vi "TLB Native Dynamic Events ver 0.18a.vi"() -> ()   [LabVIEW 2018]
uses:
  Labview Training Phase 2/Enum Controls/States for Action Engine.ctl
  TLB Type Definitions/State Type Definitions.ctl
  TLB Type Definitions/Intruction Type Definitions.ctl
  TLB Type Definitions/Encoder cluster.ctl
  TLB Type Definitions/PING CLUSTER.ctl
  <vilib>/Studica/Studica Toolkit/NavX/NavX.lvlib
  <vilib>/Studica/Studica Toolkit/Background/DIO Channel.ctl
  Underlying VI's/NavX VI/navX type def.ctl
  <vilib>/Studica/Studica Toolkit/Background/I2C Channel.ctl
  TLB Type Definitions/Vision cluster.ctl
  <vilib>/NI_Real-Time Target Support.lvlib
  TLB Type Definitions/Stepper cluster.ctl
  Experimental VI's/Archived VI's/MOTOR CONTROL NO PID Type Def.ctl
  Underlying VI's/I2C Master VI/I2C MASTER Type Def.ctl
  Underlying VI's/I2C Master VI/I2C_MASTER_WRITE_NEW Type Def.ctl
  <vilib>/userdefined/High Color/IMAQdx.ctl
  Underlying VI's/I2C Master VI/Arduino_Interfacing.ctl
  TLB Type Definitions/Yaw Cluster.ctl
  TLB Type Definitions/Time cluster.ctl
  TLB Type Definitions/Y Stepper cluster.ctl
  Underlying VI's/Modified webcam FGV/Webcam AE.ctl
  Underlying VI's/Elasped Timer/Elapsed timer control.ctl
  Underlying VI's/Motor Control VI with PID/MOTOR CONTROL WITH PID AE DATA MODE TYPE DEF.ctl
  Underlying VI's/Motor Control VI with PID/MOTOR CONTROL WITH PID AE DIRECTION TYPE DEF.ctl
  TLB Type Definitions/IR Sensor Type Def.ctl
  <vilib>/myRIO/Common/Instrument Driver Framework/myRIO v1.0/AI/typedefs/AI Channels Enum.ctl
  <vilib>/myRIO/Common/Instrument Driver Framework/myRIO v1.0/AI/typedefs/AI Channels List.ctl
  TLB Type Definitions/Motor Speed Cluster.ctl
  Underlying VI's/IMAQ Create Reference AE/IMAQ Reference AE.ctl
  <vilib>/Utility/RT CPU Load.ctl
panel:
  out "Arm IR Sensor":dbl
  out "Table obstruct":bool
  out "x-y":dbl
  out "Left IR Sensor":dbl
  out "Obstacle detected":bool
  out "Speed & distance":T1
  out "Object Center Coordinates":cluster{"x":sgl, "y":sgl}
  out "Object detection cluster":T2
  out "Time up flag":bool
  out "Task selection":u8
  in  "Object recognition mode":enum16{"Ball", "Soap", "Gel", "Pipe", "None"}(ring)
  out "NavX Readings":T3
  out "Arduino Data":T4
  out "CPU loads":T5[](array[typedef]) {"ISR (%)" format="%#.2f"; "Idle (%)" format="%#.2f"; "Background (%)" format="%#.2f"; "Normal (%)" format="%#.2f"; "Above Normal (%)" format="%#.2f"; "High (%)" format="%#.2g"; "Timed Structures (%)" format="%#.2g"; "Time Critical (%)" format="%#.2g"; "Total (%)" format="%#.2g"}
  out "TASK ENABLE":bool
  out "Rising Edge":bool
  in  "Green LED":bool
  out "I2C Error":errorcluster
  out "State Logic":T6=enum."Startup"
  out "elements":T7[](array[typedef])
  in  "STOP TASK":bool
  in  "OK Button":bool
  in  "STOP":bool
  out "error out":errorcluster
  out "Action Queue Items":i32
  out "State Logic Queue Items":i32
  out "Action Queues items":string[](array[string])=["Hardware reset", "Software reset", ""]
  out "Action State":string
  # "System Health Status Update"
  # "VISION"
  # "TLB FRAMEWORK STATUS"
  # "Test Programme written by Calvin Loke    Dated: 28 Aug 2019\nTest Programme revised by Dr Alex See   Dated 30 Aug 2019\n\nRevision date: 20/03/2020\nProgramme version:   TLB Native Dynamic Events ver 0.14a"
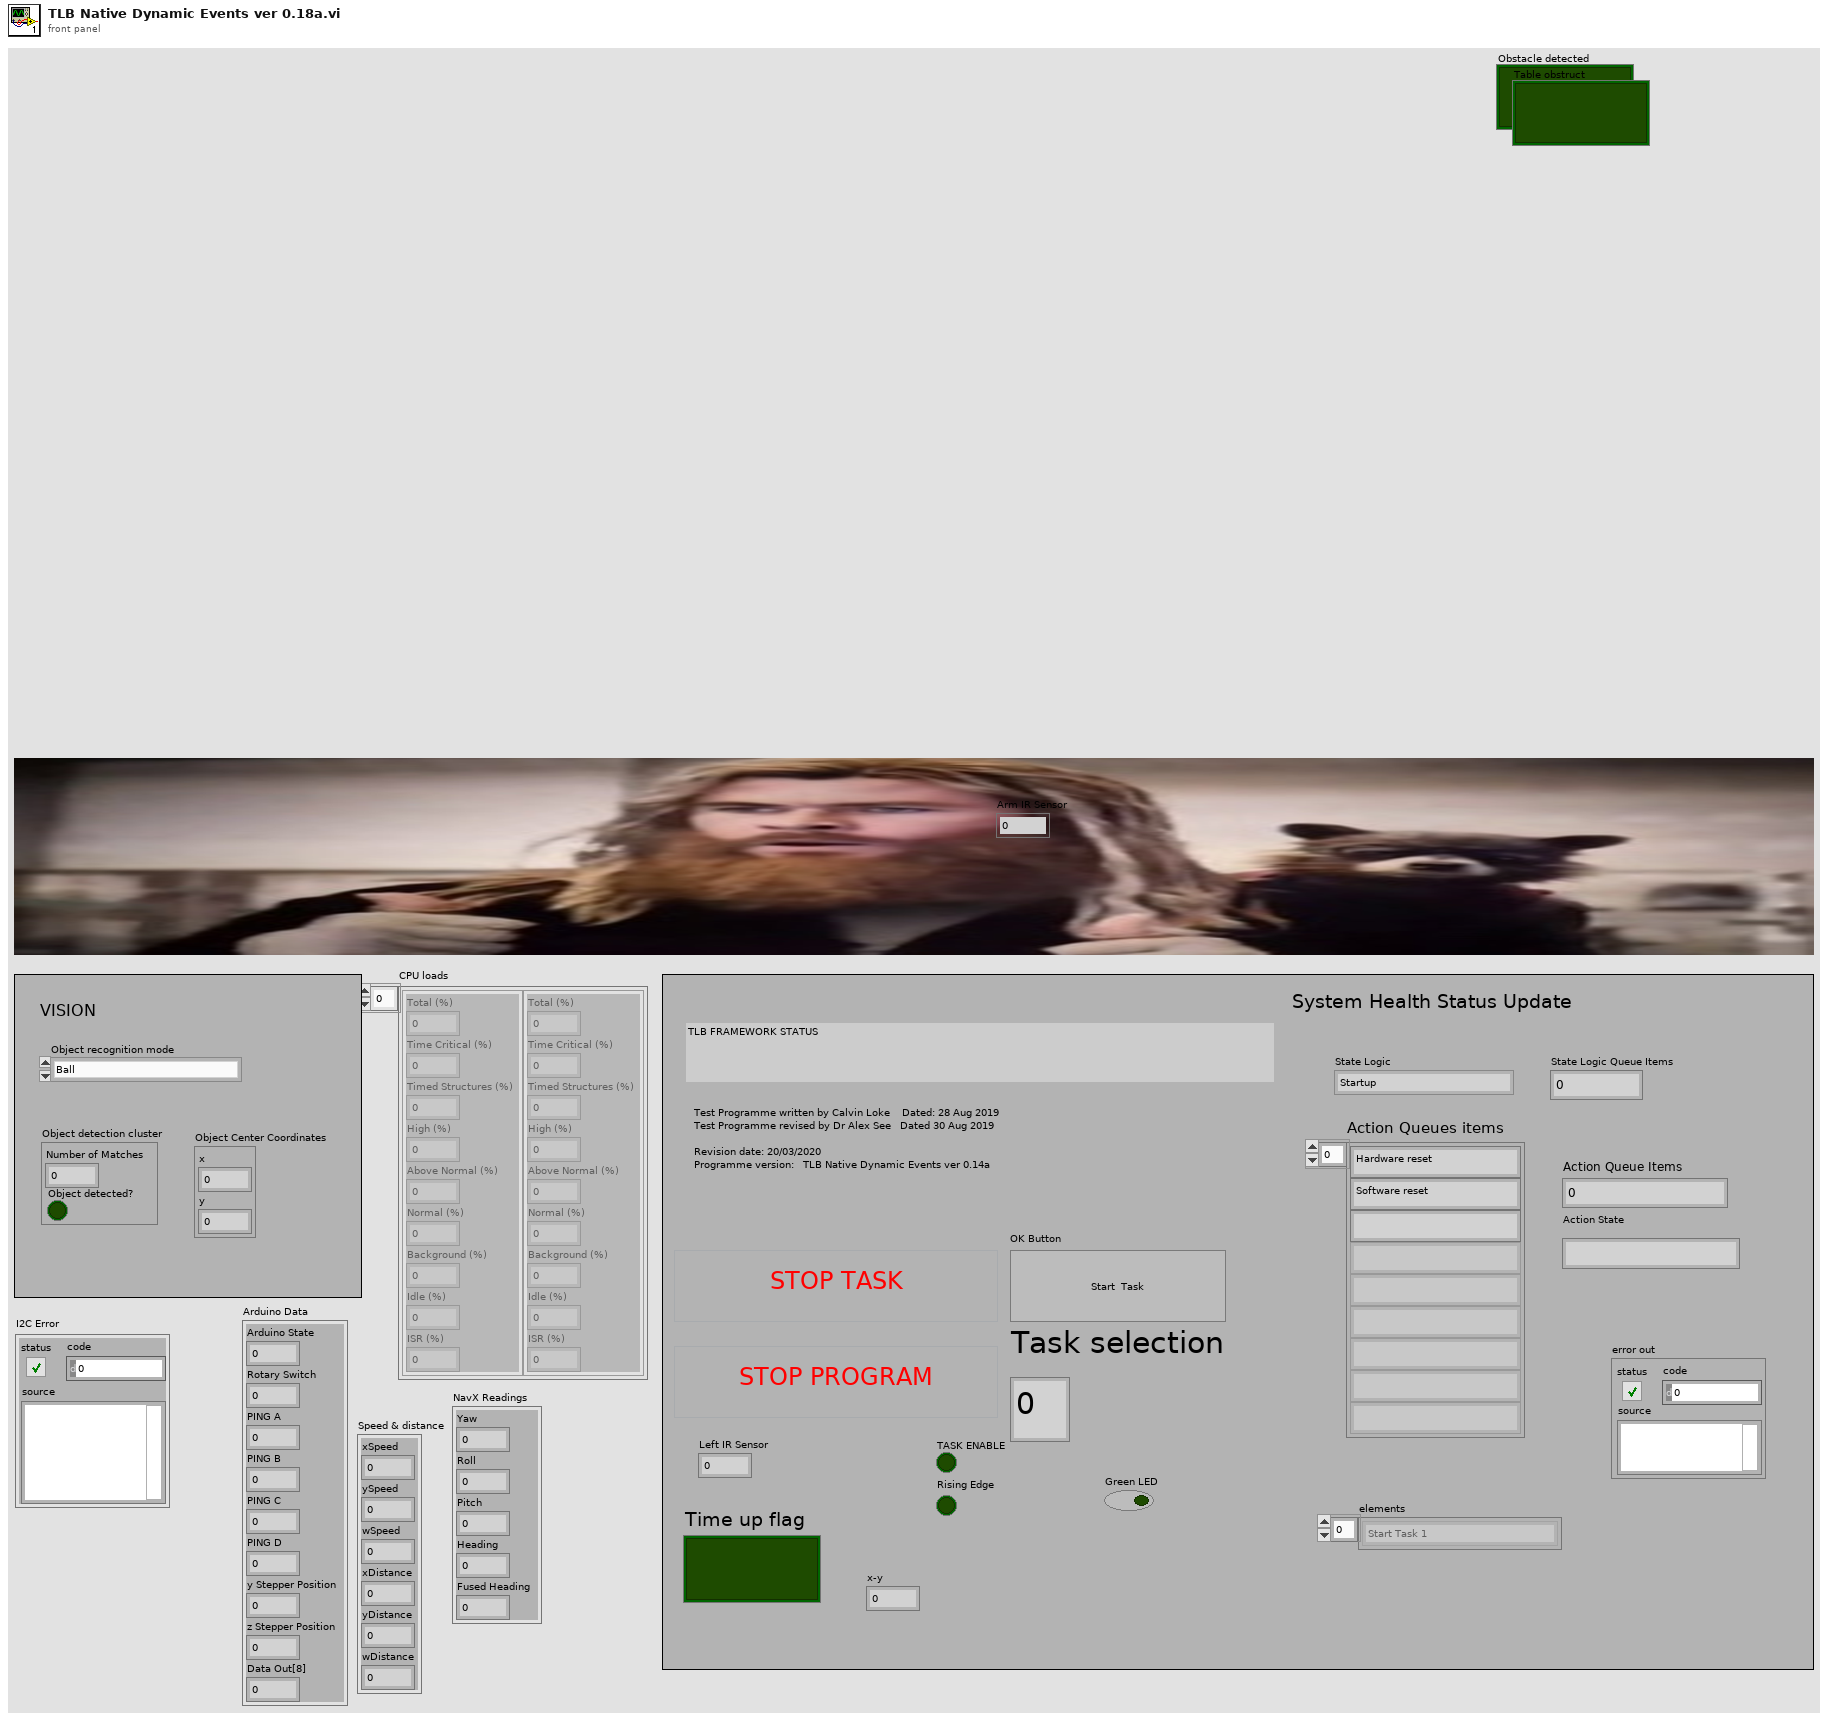
[diagram p1: front panel]
types:
  T1 = cluster{"xSpeed":dbl, "ySpeed":dbl, "wSpeed":dbl, "xDistance":dbl, "yDistance":dbl, "wDistance":dbl}
  T2 = cluster{"Number of Matches":i32, "Object detected?":bool}
  T3 = cluster{"Yaw":dbl, "Roll":dbl, "Pitch":dbl, "Heading":dbl, "Fused Heading":dbl}
  T4 = cluster{"Arduino State":u8, "Rotary Switch":u8, "PING A":u8, "PING B":u8, "PING C":u8, "PING D":u8, "y Stepper Position":u8, "z Stepper Position":u8, "Data Out[8]":u8}
  T5 = typedef "NI_Real-Time Target Support.lvlib/RT CPU Load.ctl" = cluster{"Total (%)":dbl, "Time Critical (%)":dbl, "Timed Structures (%)":dbl, "High (%)":dbl, "Above Normal (%)":dbl, "Normal (%)":dbl, "Background (%)":dbl, "Idle (%)":dbl, "ISR (%)":dbl}
  T6 = typedef "State Type Definitions.ctl" = enum16{"None", "Startup", "Move to Angle", "True Stop", "Idle", "Shutdown", "Task 1A", "Task 1B", "Task 2:Raise Arm", "Task 2:Sensor Mode", "Task 2:Reverse Mode", "Task 3", "Task 4_A", "Task 4_B", "Task 4_C", "Task 4_D", "Task 5A", "Task 5B", "Task 5C", "Task 5D", "Task 5E: POSITION ARM", "Task 5F: ARM GRAB HEIGHT", "Task 5G: CLOSE CLAW", "Task 5H: RAISE ARM", "Task 6_A", "Task 6_B", "Task 7", "Task 8A: RAISE ARM", "Task 8B: MOVE TO BOX", "Task 8C: CAM BURST", "Task 8D: PROCESS IMAGE", "Task 8E: ROBOT ADJUST", "Task 8F: CAM BURST 2", "Task 8G: PROCESS IMAGE 2", "Task 8H: ARM ADJUST", "Task 8I: ARM GRAB HEIGHT", "Task 8J: CLOSE CLAW", "Task 8K: RAISE MY SWORD", "Task 9A: Raise Arm", "Task 9B: Rotate to Angle", "Task 9C: Detect Box", "Task 9D: MOVE FORWARD", "Task 9E: MOVE LEFT", "Task 9F: SCAN IMAGE", "Task 9G: PROCESS COLOUR", "Task 9H: MOVE RIGHT", "Task 9I: SCAN IMAGE", "Task 9J: PROCESS COLOUR", "Task 9K: ROTATE 90 CW", "Task 9L: MOVE FORWARD", "Task 9M: MOVE RIGHT", "Task 9N: SCAN IMAGE", "Task 9O: PROCESS COLOUR", "Task 9P: MOVE RIGHT", "Task 9Q: SCAN IMAGE", "Task 9R: PROCESS COLOUR", "Task A1: Raise Arm", "Task A2: Rotate to Angle", "Task A3: Move Forward", "Task A4: Rotate CW 90"}
  T7 = typedef "Intruction Type Definitions.ctl" = enum16{"None", "Start Task 1", "Start Task 2", "Start Task 3", "Start Task 4", "Start Task 5", "Start Task 6", "Start Task 7", "Start Task 8 - BALL", "Start Task 8 - Gel", "Start Task 8 - Pipe", "Start Task 8 - Soap", "Start Task 9", "Start Task A", "Start Task B", "Exit"}
  T8 = typedef "Motor Speed Cluster.ctl" = cluster{"ySpeed":dbl, "xSpeed":dbl, "wSpeed":dbl}
  T9 = typedef "IR Sensor Type Def.ctl" = cluster{"Left IR Sensor":dbl, "Arm IR Sensor":dbl, "Bottom IR Sensor":dbl}
  T10 = typedef "Y Stepper cluster.ctl" = cluster{"yStepper desired":u8}
  T11 = typedef "Time cluster.ctl" = cluster{"Time up flag":bool, "SET TIME TO CHECK":dbl}
  T12 = typedef "Yaw Cluster.ctl" = cluster{"Yaw":dbl, "Compass":dbl}
  T13 = typedef "Stepper cluster.ctl" = cluster{"y Stepper Position":u8, "z Stepper Position":u8}
  T14 = typedef "DIO Channel.ctl" = enum16{"Not Connected", "A/DIO1", "A/DIO2", "A/DIO3", "A/DIO4", "A/DIO5", "A/DIO6", "A/DIO7", "A/DIO13", "B/DIO1", "B/DIO2", "B/DIO3", "B/DIO4", "B/DIO5", "B/DIO6", "B/DIO7", "B/DIO13", "C/DIO0", "C/DIO1", "C/DIO2", "C/DIO3", "C/DIO4", "C/DIO5", "C/DIO6", "C/DIO7"}
  T15 = typedef "Vision cluster.ctl" = cluster{"Recognized Object":bool, "Object X coordinate":dbl, "Object Y coordinate":dbl}
  T16 = typedef "PING CLUSTER.ctl" = cluster{"PING_A":u8, "PING_B":u8, "PING_C":u8, "PING_D":u8}
  T17 = typedef "Encoder cluster.ctl" = cluster{"xDistance":dbl, "yDistance":dbl, "wDistance":dbl}
  T18 = cluster{"DIO Channel":T14, "FPGA VI Reference Out":refnum<k20>}
  T19 = typedef "navX type def.ctl" = enum16{"Get i2C reference", "Read Values", "Zero Yaw"}
  T20 = typedef "Arduino_Interfacing.ctl" = enum16{"Initialize", "Write to Arduino", "Read From Arduino"}
  T21 = typedef "I2C Channel.ctl" = enum16{"Not Connected", "A", "B"}
  T22 = typedef "States for Action Engine.ctl" = enum16{"Initialize", "Write", "Read"}
  T23 = cluster{"I2C Ref Out":cluster{"I2C Channel":T21, "FPGA VI Reference Out":refnum<k20>}, "Connected":bool, "Slave Address (7-bit)":u8, "Registry":u8[]}
  T24 = typedef "Intruction Type Definitions.ctl" = enum16{"None", "Start Task 1", "Start Task 2", "Start Task 3", "Start Task 4", "Start Task 5", "Start Task 6", "Start Task 7", "Start Task 8", "Start Task 9", "Start Task A", "Start Task B", "Exit"}
  T25 = typedef "State Type Definitions.ctl" = enum16{"None", "Startup", "Move to Angle", "True Stop", "Idle", "Shutdown", "Task 1", "Task 2:Raise Arm", "Task 2:Sensor Mode", "Task 2:Reverse Mode", "Task 3", "Task 4_A", "Task 4_B", "Task 4_C", "Task 4_D", "Task 5A: ARM CAM HEIGHT", "Task 5B: MOVE TO BOX", "Task 5C: CAM BURST", "Task 5D: PROCESS IMAGE", "Task 5E: POSITION ARM", "Task 5F: ARM GRAB HEIGHT", "Task 5G: CLOSE CLAW", "Task 5H: RAISE ARM", "Task 6_A", "Task 6_B", "Task 7", "Task 8A: RAISE ARM", "Task 8B: MOVE TO BOX", "Task 8C: CAM BURST", "Task 8D: PROCESS IMAGE", "Task 8E: ROBOT ADJUST", "Task 8F: CAM BURST 2", "Task 8G: PROCESS IMAGE 2", "Task 8H: ARM ADJUST", "Task 8I: ARM GRAB HEIGHT", "Task 8J: CLOSE CLAW", "Task 8K: RAISE MY SWORD", "Task 9A: Raise Arm", "Task 9B: Rotate to Angle", "Task 9C: Rotation alignmnet", "Task A: RAISE ARM TO HEIGHT", "Task A: MOVE FORWARD"}
  T26 = typedef "MOTOR CONTROL WITH PID AE DIRECTION TYPE DEF.ctl" = enum16{"y-axis movement", "x-axis movement", "rotation", "stop", "reset encoders"}
  T27 = typedef "MOTOR CONTROL WITH PID AE DATA MODE TYPE DEF.ctl" = enum16{"Init AE", "Write to AE", "Read from AE"}
  T28 = typedef "IMAQ Reference AE.ctl" = enum16{"Initialize AE", "Get IMAQ Reference", "Dispose Processing Buffer"}
  T29 = typedef "Elapsed timer control.ctl" = enum16{"Start", "Pause", "Initialize"}
  T30 = typedef "I2C_MASTER_WRITE_NEW Type Def.ctl" = enum16{"Ultrasonic sensors", "Stepper origin", "zStepper 13.3k", "zStepper 13k", "zStepper 12k", "zStepper 11k", "zStepper 10k", "zStepper 9k", "zStepper 8k", "zStepper 7k", "zStepper 6k", "zStepper 5k", "zStepper 4k", "zStepper 3k", "zStepper 2k", "zStepper 1k", "zStepper 900", "zStepper 800", "zStepper 700", "zStepper 600", "zStepper 500", "zStepper 400", "zStepper 300", "zStepper 200", "zStepper 100", "zStepper 0", "yStepper control", "Open Claw", "Close Claw", "Soft Reset"}
  T31 = typedef "Webcam AE.ctl" = enum16{"Initialize Camera", "Open Camera", "Continuous Acquisition", "Close Camera", "Retrieve Image", "Dispose Camera Image Buffer"}
  T32 = typedef "IMAQdx.ctl" = refnum<k21>
  T33 = typedef "Webcam AE.ctl" = enum16{"Initialize Camera", "Open Camera", "Continuous Acquisition", "Close Camera", "Retrieve Image", "Dispose Image Buffers"}
  T34 = typedef "IMAQ Reference AE.ctl" = enum16{"Initialize AE", "Get IMAQ Reference", "Destroy ALL IMAQ"}
  T35 = typedef "MOTOR CONTROL NO PID Type Def.ctl" = enum16{"Init", "Front Back", "Left Right", "Rotate", "Stop", "Latch"}
  T36 = typedef "AI Channels List.ctl" = T37[]
  T37 = typedef "AI Channels Enum.ctl" = enum16{"Not Connected", "AudioIn/Left", "AudioIn/Right", "C/AI0", "C/AI1", "A/AI0", "A/AI1", "A/AI2", "A/AI3", "A/AI4", "A/AI5", "A/AI6", "A/AI7", "B/AI0", "B/AI1", "B/AI2", "B/AI3", "B/AI4", "B/AI5", "B/AI6", "B/AI7", "AI/AI0", "AI/AI1", "AI/AI2", "AI/AI3", "A/AI0 (DIFF)", "A/AI1 (DIFF)", "A/AI2 (DIFF)", "A/AI3 (DIFF)", "B/AI0 (DIFF)", "B/AI1 (DIFF)", "B/AI2 (DIFF)", "B/AI3 (DIFF)"}
  T38 = typedef "I2C MASTER Type Def.ctl" = enum16{"Last State", "Mode 0", "Mode 1", "Mode 2", "Mode 3", "Mode 4", "Mode 5", "Mode 6", "Mode 7", "Mode 8", "Mode 9", "Mode 10"}
  T39 = typedef "IMAQ Image.ctl" = refnum<image>
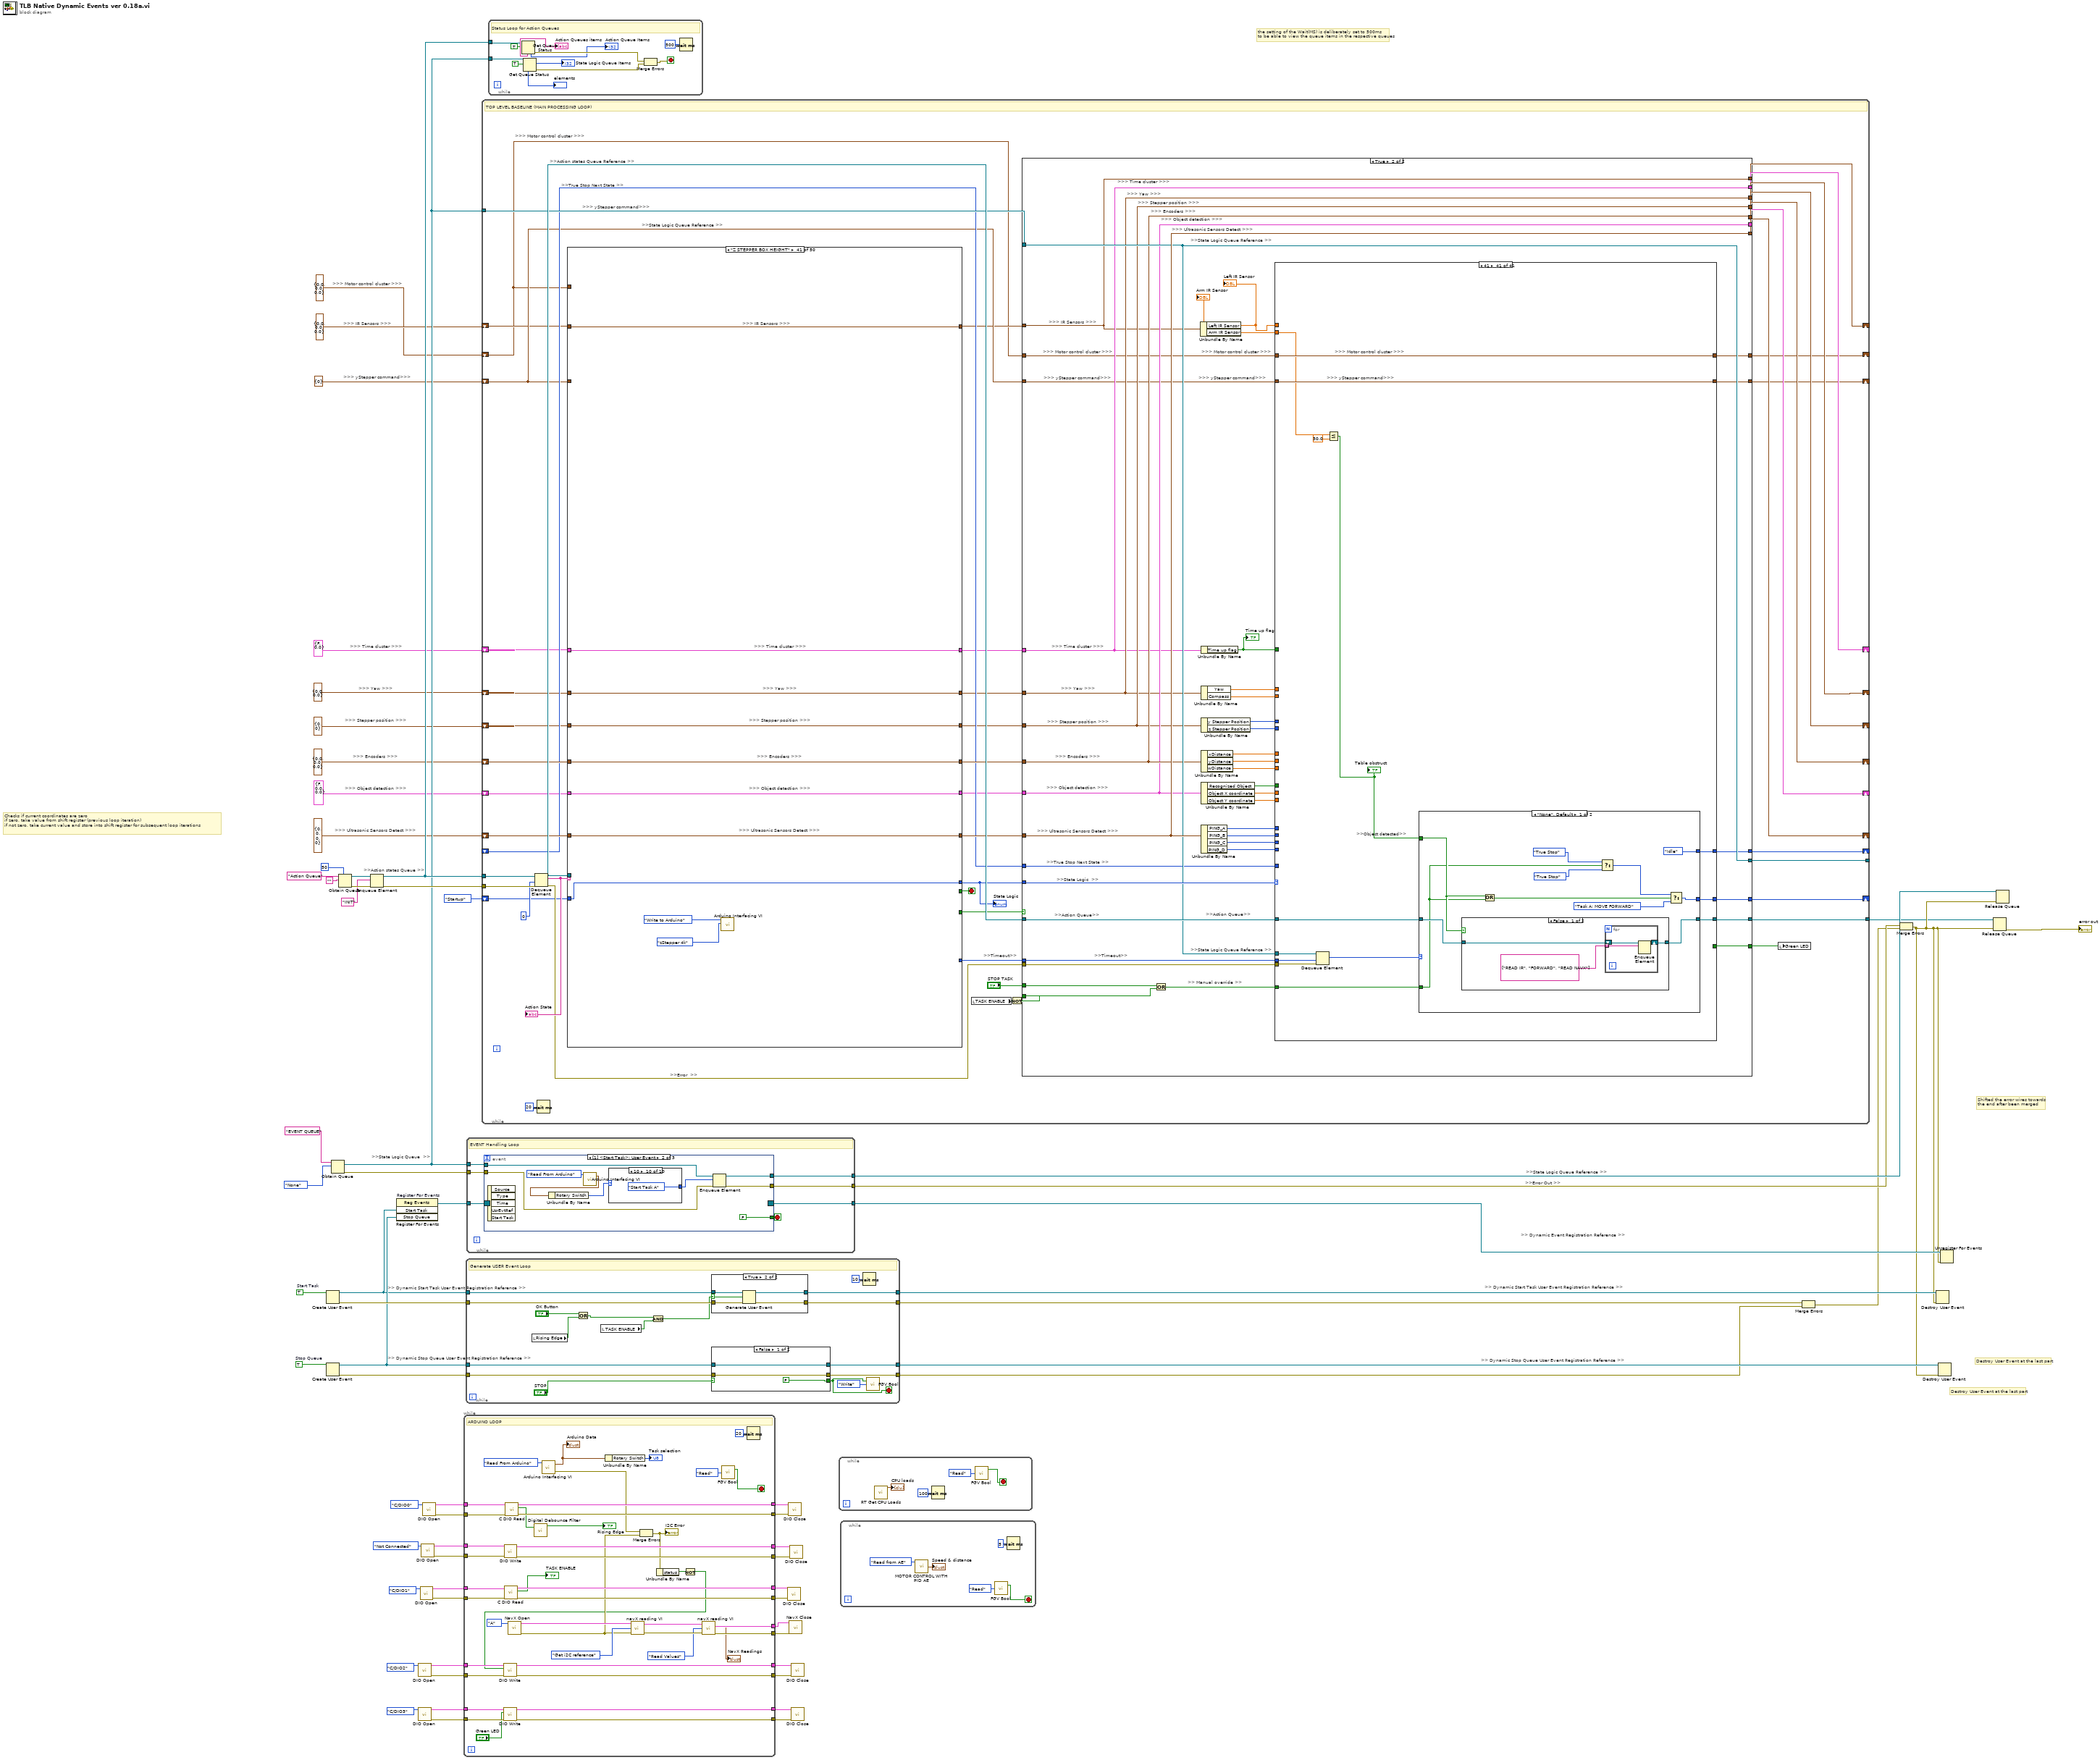
[diagram p0: block diagram]
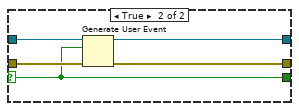
[diagram p2: hidden frame]
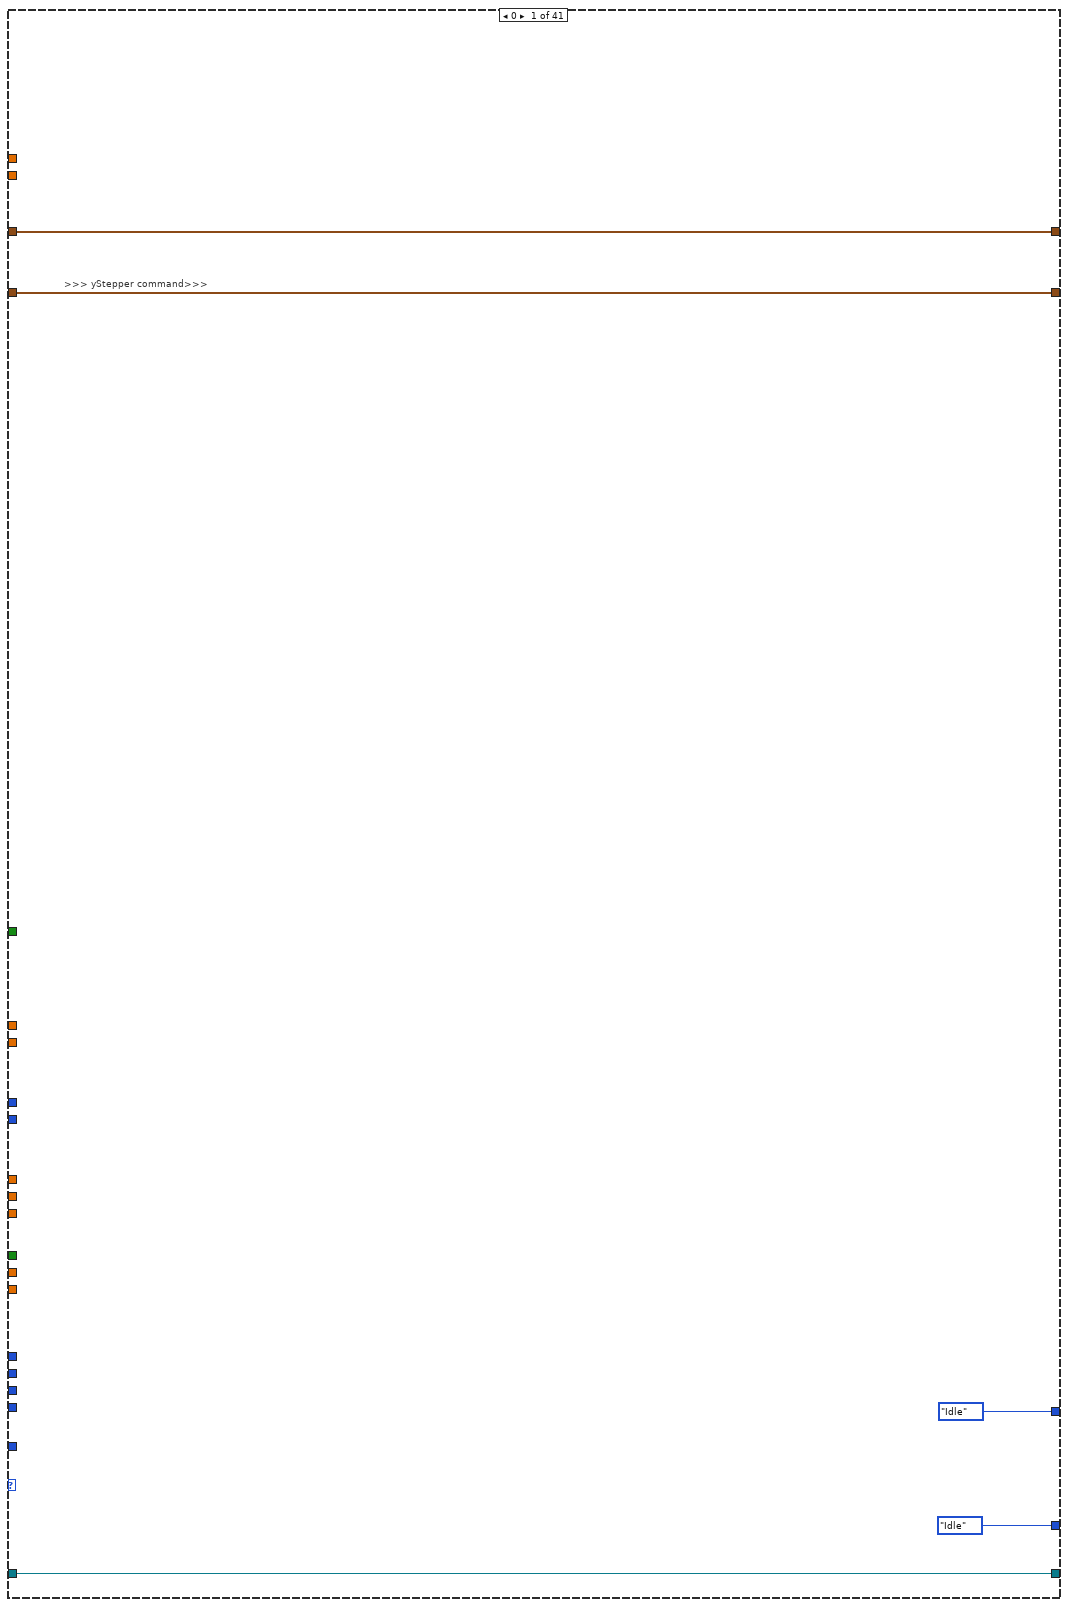
[diagram p5: hidden frame]
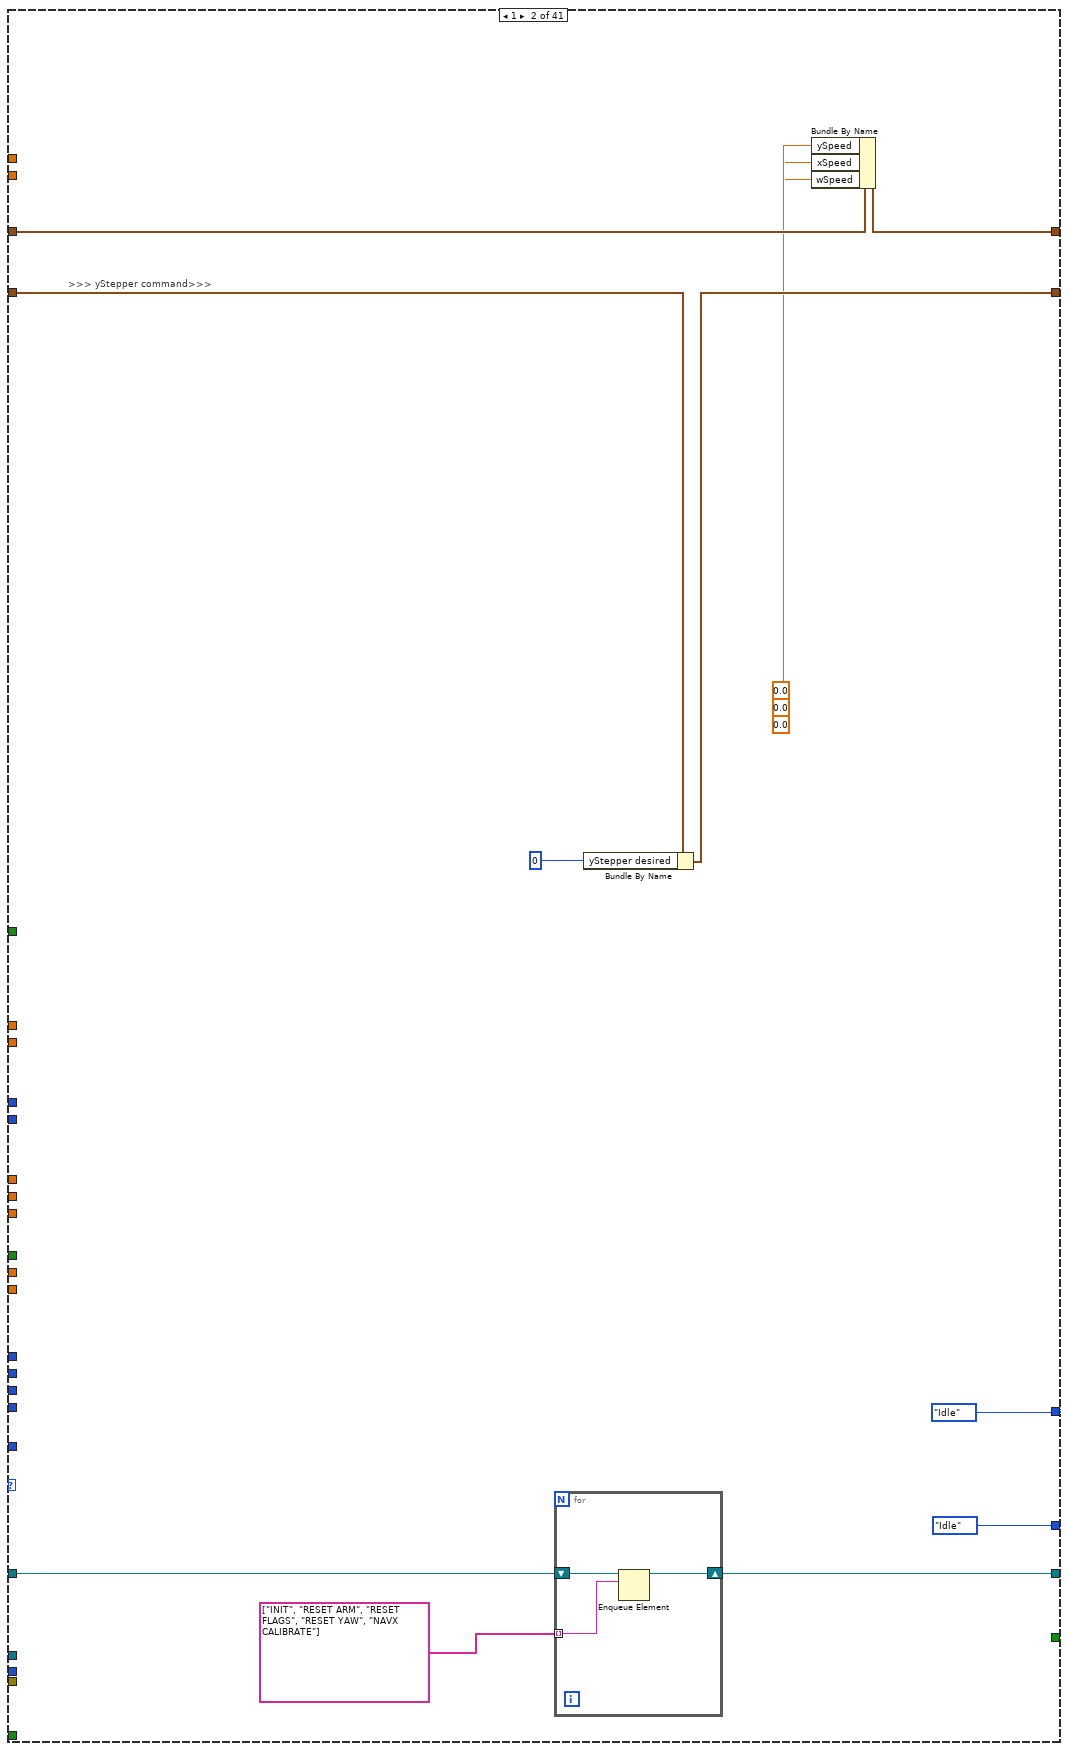
[diagram p6: hidden frame]
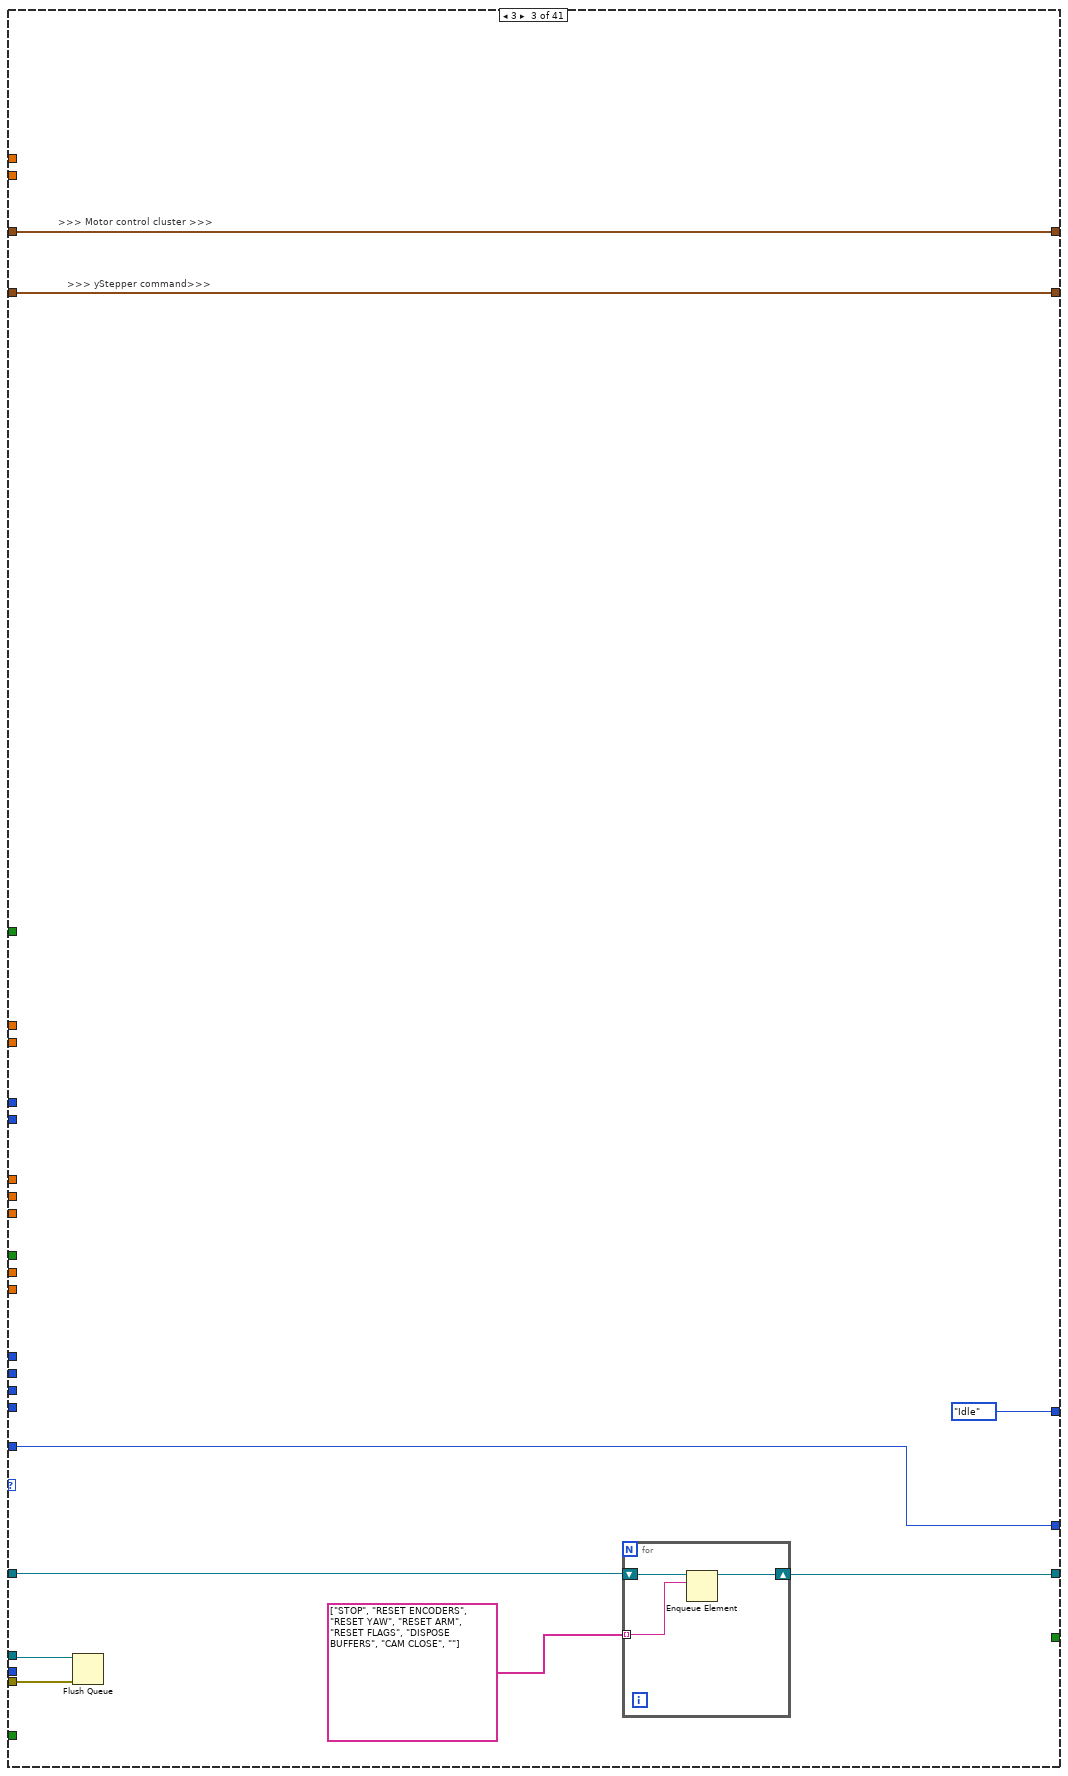
[diagram p7: hidden frame]
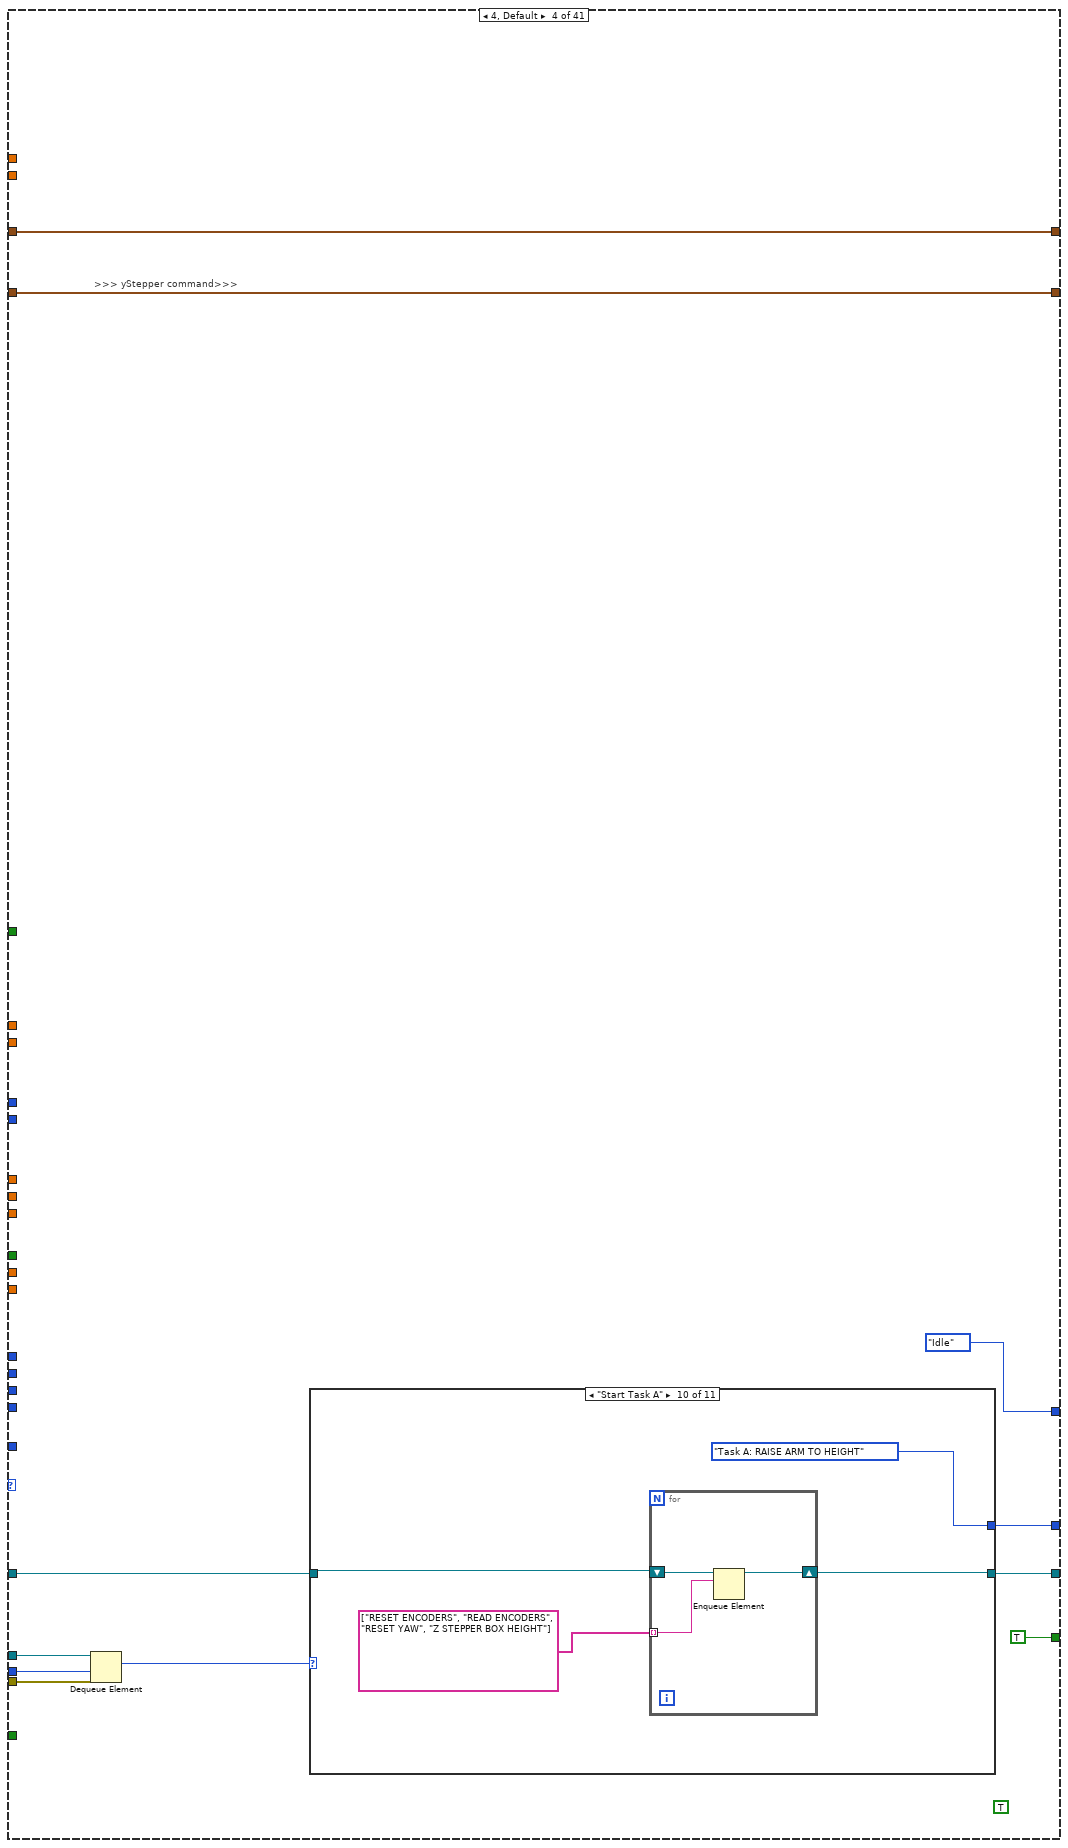
[diagram p8: hidden frame]
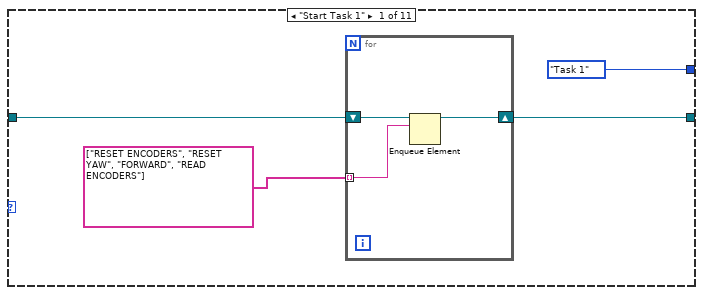
[diagram p9: hidden frame]
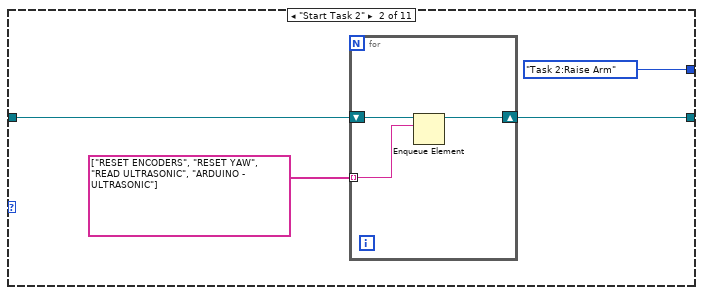
[diagram p10: hidden frame]
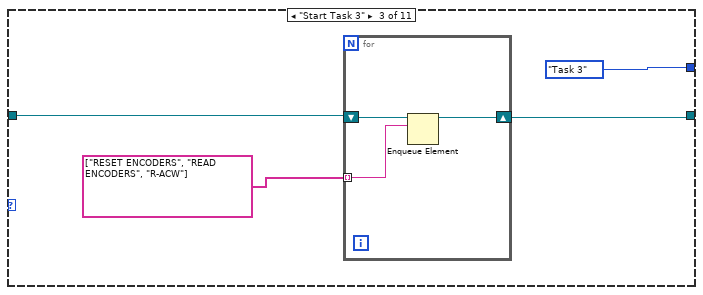
[diagram p11: hidden frame]
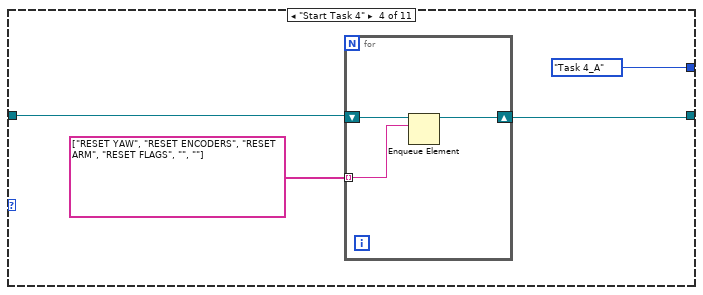
[diagram p12: hidden frame]
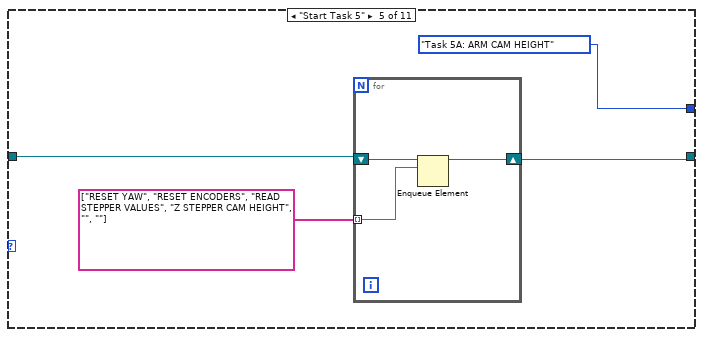
[diagram p13: hidden frame]
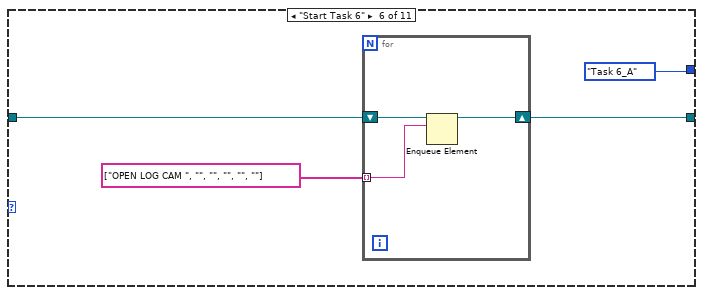
[diagram p14: hidden frame]
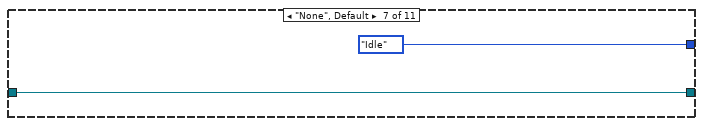
[diagram p15: hidden frame]
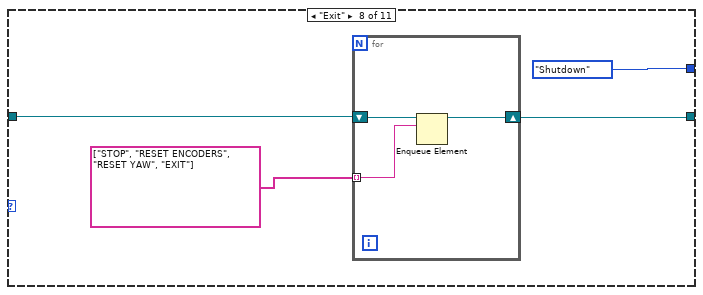
[diagram p16: hidden frame]
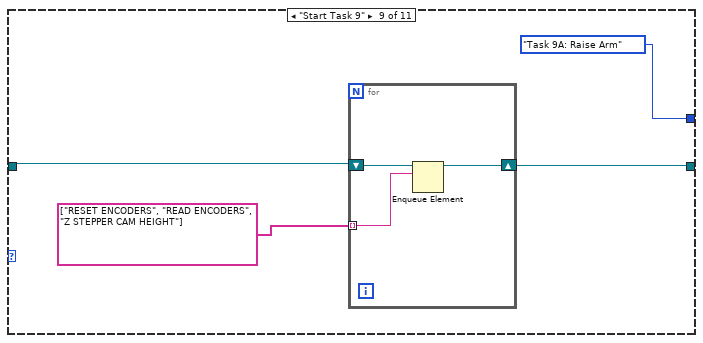
[diagram p17: hidden frame]
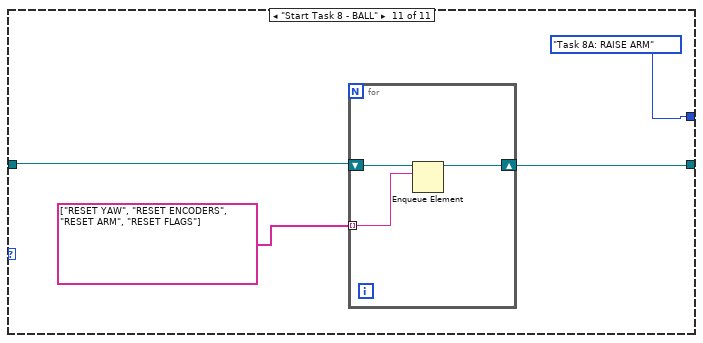
[diagram p18: hidden frame]
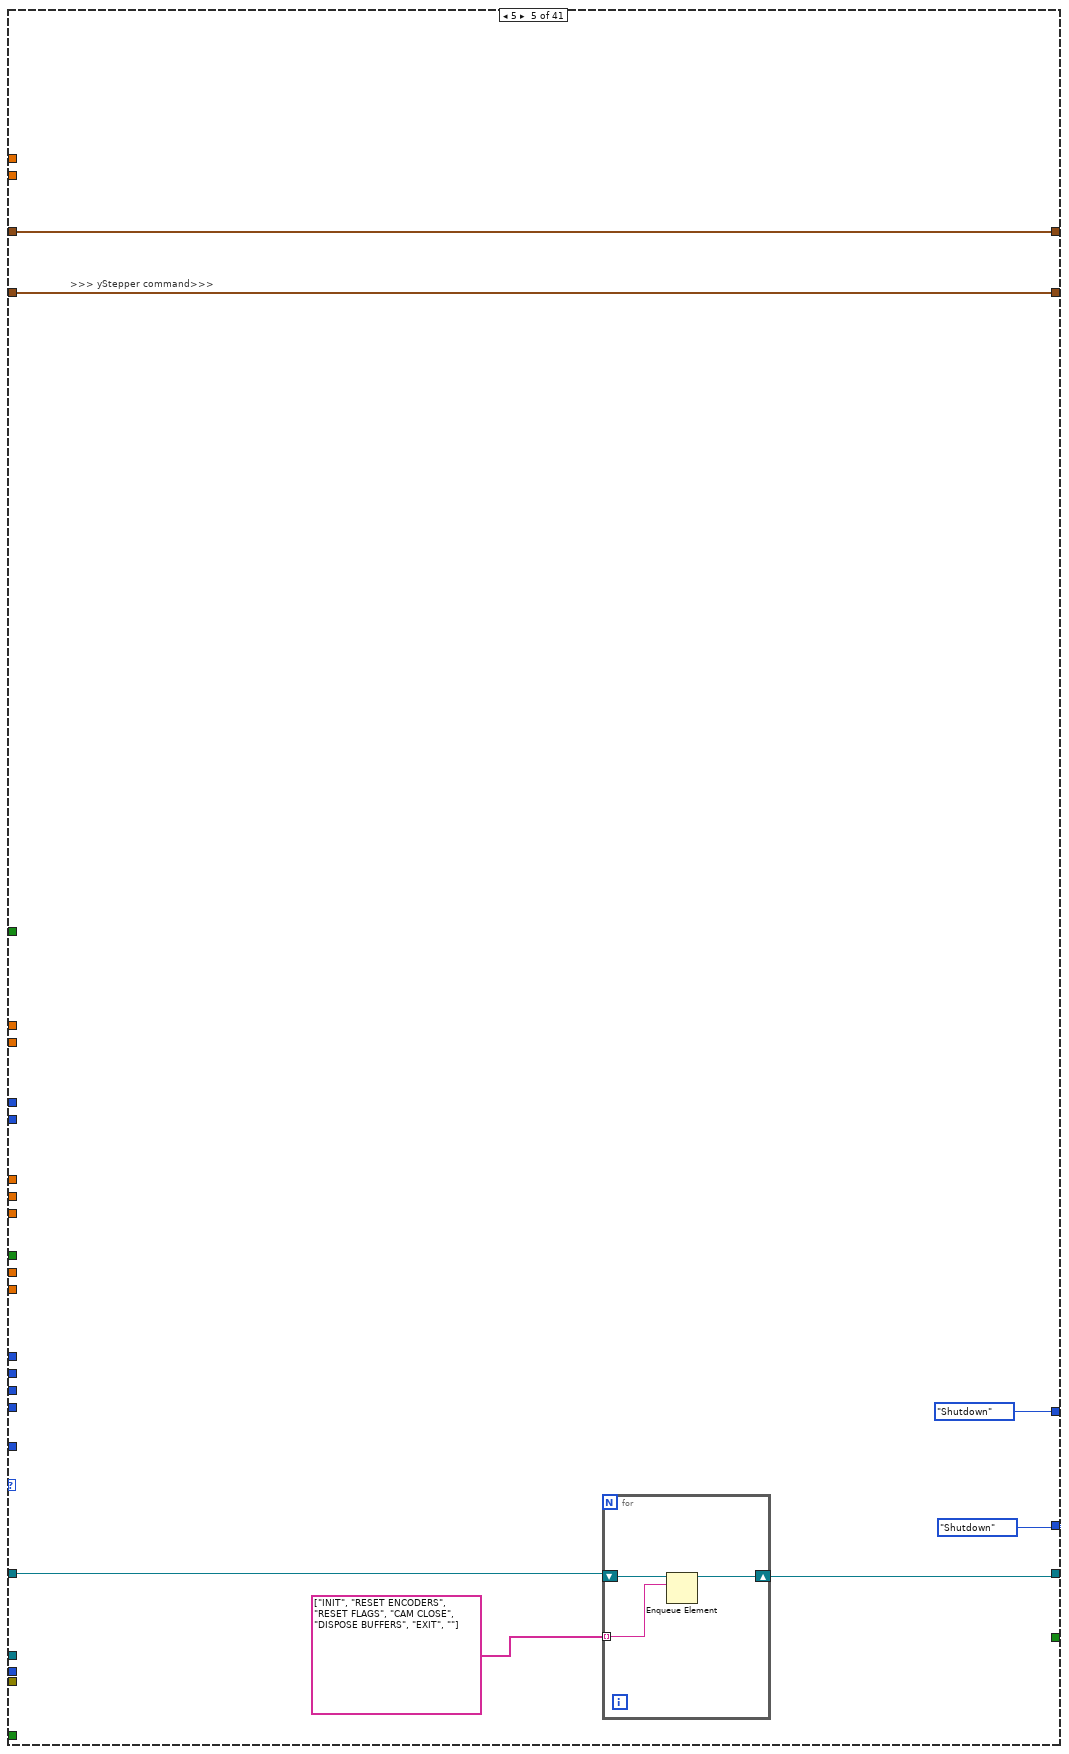
[diagram p19: hidden frame]
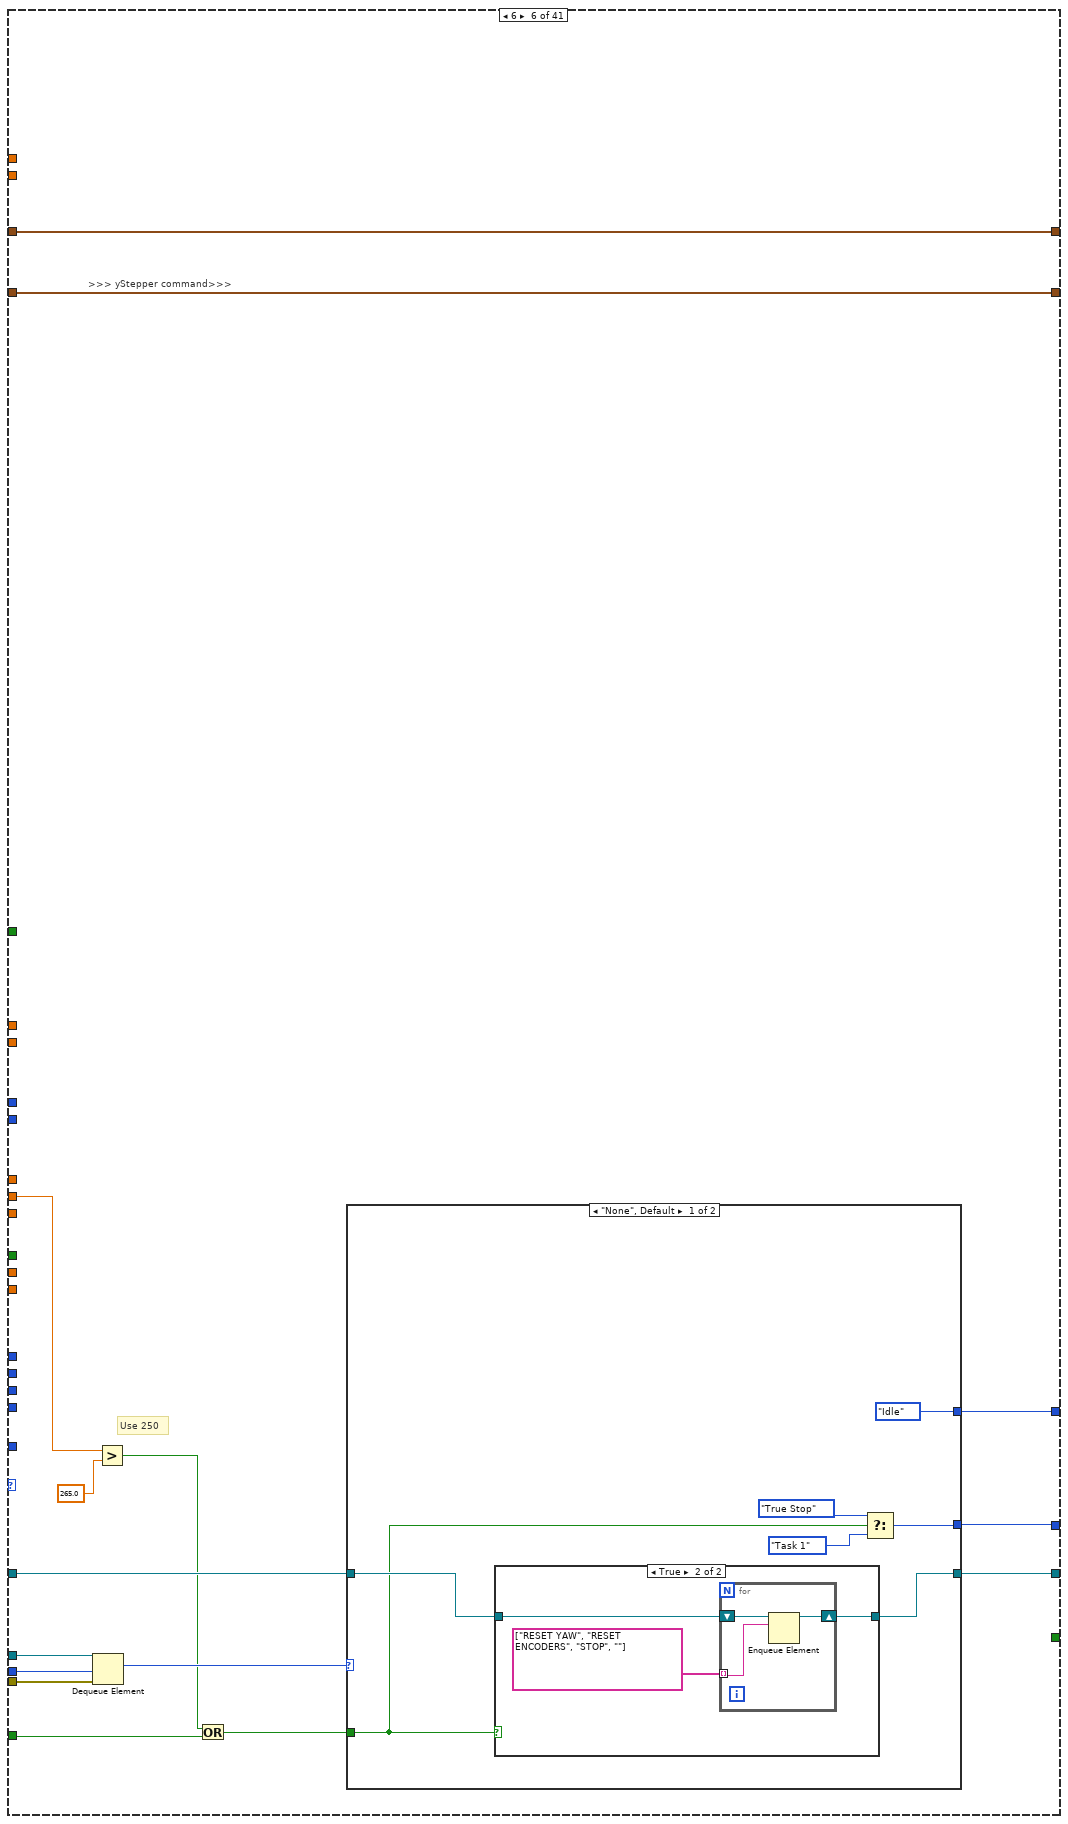
[diagram p20: hidden frame]
diagram:
  w67 = TRUE  # Stop Queue
  w66 = TRUE  # Start Task
  # ">>> Motor control cluster >>>"
  # ">>> IR Sensors >>>"
  # "Checks if current coordinates are zero\nif zero, take value from shift register (previous loop iteration)\nif not zero, take current value and store into shift register for subsequent loop iterations"
  # ">>> yStepper command>>>"
  # ">>> Time cluster >>>"
  # ">>> Yaw >>>"
  # ">>> Stepper position >>>"
  # ">>> Encoders >>>"
  # ">>> Object detection >>>"
  # ">>> Ultrasonic Sensors Detect >>>"
  # "the setting of the Wait(MS) is deliberately set to 500ms\nto be able to view the queue items in the respective queues"
  # ">>Error Out >>"
  # ">> Dynamic Stop Queue User Event Registration Reference >>"
  # ">> Dynamic Start Task User Event Registration Reference >>"
  # ">> Dynamic Stop Queue User Event Registration Reference >>"
  # ">> Dynamic Start Task User Event Registration Reference >>"
  # ">> Dynamic Event Registration Reference >>"
  # ">>Action states Queue >>"
  # ">>State Logic Queue  >>"
  # ">>State Logic Queue Reference >>"
  # "Destroy User Event at the last part"
  # "Destroy User Event at the last part"
  # "Shifted the error wires towards\nthe end after been merged"
  n1 = Create User Event(user event datatype=w66) -> (user event=w58:refnum<user-event>, error out=w63:errorcluster)  [unwired: 1 in]
  n2 = Create User Event(user event datatype=w67) -> (user event=w59:refnum<user-event>, error out=w62:errorcluster)  [unwired: 1 in]
  n3 = Obtain Queue(name (unnamed)="EVENT QUEUE", element data type=Intruction_Type_Definitions."None" ("Enum")) -> (queue out=w44:refnum<queue>, error out=w50:errorcluster)  [unwired: 3 in, 1 out]
  n4 = Obtain Queue(max queue size (-1, unlimited)=50, name (unnamed)="Action Queue", element data type="") -> (queue out=w53:refnum<queue>, error out=w49:errorcluster)  [unwired: 2 in, 1 out]
  n5 = Enqueue Element(queue=w53, element="INIT", error in (no error)=w49) -> (queue out=w45:refnum<queue>, error out=w48:errorcluster)  [unwired: 1 in, 1 out]
  n6 = register-events "Register For Events"(w58, w59) -> (reference out=w57:refnum<event-registration>)  [unwired: 2 in, 1 out]
  n7 = call <vilib>:"DIO Open.vi"("DIO Channel"=DIO_Channel."C/DIO2") -> ("error out"=w17:errorcluster, "DIO Info Out"=w18:T18)  [unwired: 9 in]
  n8 = call <vilib>:"DIO Open.vi"("DIO Channel"=DIO_Channel."C/DIO3") -> ("error out"=w12:errorcluster, "DIO Info Out"=w13:T18)  [unwired: 9 in]
  n9 = call <vilib>:"DIO Open.vi"("DIO Channel"=DIO_Channel."C/DIO1") -> ("error out"=w22:errorcluster, "DIO Info Out"=w23:T18)  [unwired: 9 in]
  n10 = call <vilib>:"DIO Open.vi"("DIO Channel"=DIO_Channel."Not Connected") -> ("error out"=w27:errorcluster, "DIO Info Out"=w29:T18)  [unwired: 9 in]
  n11 = call <vilib>:"DIO Open.vi"("DIO Channel"=DIO_Channel."C/DIO0") -> ("error out"=w32:errorcluster, "DIO Info Out"=w35:T18)  [unwired: 9 in]
  n12 = while {
    tunnel: w35 -> [w108]
    tunnel: [w107] -> w33
    tunnel: w32 -> [w106]
    tunnel: [w105] -> w31
    tunnel: w29 -> [w102]
    tunnel: [w101] -> w28
    tunnel: w27 -> [w100]
    tunnel: [w99] -> w26
    tunnel: [w98] -> w24
    tunnel: w23 -> [w97]
    tunnel: w22 -> [w96]
    tunnel: [w95] -> w21
    tunnel: w18 -> [w89]
    tunnel: w17 -> [w88]
    tunnel: [w87] -> w16
    tunnel: [w86] -> w15
    tunnel: w13 -> [w85]
    tunnel: w12 -> [w84]
    tunnel: [w83] -> w11
    tunnel: [w82] -> w10
    tunnel: [w76] -> w7
    tunnel: [w75] -> w8
    stop <- w110 stop-if-true
    # "ARDUINO LOOP"
    n13 = call <vilib>:"DIO Write.vi"("error in (no error)"=w84, "Input"="Green LED", "DIO Info In"=w85) -> ("error out"=w82:errorcluster, "DIO Info Out"=w83:T18)  [unwired: 7 in]
    n14 = call <vilib>:"DIO Write.vi"("error in (no error)"=w100, "DIO Info In"=w102) -> ("error out"=w99:errorcluster, "DIO Info Out"=w101:T18)  [unwired: 8 in]
    n15 = call <vilib>:"C DIO Read.vi"("error in (no error)"=w96, "DIO Info In in"=w97) -> ("error out"=w95:errorcluster, "IN"=→"TASK ENABLE":bool, "DIO Info In out"=w98:T18)  [unwired: 7 in]
    n16 = call <vilib>:"C DIO Read.vi"("error in (no error)"=w106, "DIO Info In in"=w108) -> ("error out"=w105:errorcluster, "IN"=w104:bool, "DIO Info In out"=w107:T18)  [unwired: 7 in]
    n17 = call <vilib>:"NavX Open.vi"("I2C Channel"=I2C_Channel."A") -> ("error out"=w91:errorcluster, "NavX Info"=w93:T23)  [unwired: 9 in]
    n18 = call "Digital Debounce Filter.vi"("Boolean input"=w104) -> ("Rising Edge"=→"Rising Edge":bool)  [unwired: 1 in, 2 out]
    n19 = call "Arduino Interfacing VI.vi"("AE Mode"=Arduino_Interfacing."Read From Arduino") -> ("error out"=w79:errorcluster, "Arduino Data"=w72:T4)  [unwired: 3 in]
    "Arduino Data" <- w72
    n20 = Unbundle By Name(w72) -> ("Rotary Switch"=→"Task selection":u8)
    n21 = call "navX reading VI.vi"("NavX Info In"=w93, "Mode"=navX_type_def."Get i2C reference", "error in (no error)"=w91) -> ("NavX Info Out"=w78:T23, "Error Out"=w77:errorcluster)  [unwired: 2 out]
    n22 = Merge Errors(w79, w91) -> (w70:errorcluster)
    "I2C Error" <- w70
    n23 = Unbundle By Name(w70) -> ("status"=w69:bool)
    n24 = Not(x=w69) -> (.not. x?=w68:bool)
    n25 = call <vilib>:"DIO Write.vi"("error in (no error)"=w88, "Input"=w68, "DIO Info In"=w89) -> ("error out"=w86:errorcluster, "DIO Info Out"=w87:T18)  [unwired: 7 in]
    n26 = call "navX reading VI.vi"("NavX Info In"=w78, "Mode"=navX_type_def."Read Values", "error in (no error)"=w77) -> ("NavX Info Out"=w76:T23, "NavX Readings"=→"NavX Readings":T3, "Error Out"=w75:errorcluster)  [unwired: 1 out]
    n27 = call "FGV Bool.vi"("Init/Read/Write State"=States_for_Action_Engine."Read") -> ("Output node"=w110:bool)  [unwired: 2 in, 1 out]
    n28 = Wait (ms)(milliseconds to wait=u32 20) -> ()  [unwired: 1 out]
  }
  n29 = while {
    tunnel: w58 -> [w128]
    tunnel: w59 -> [w127]
    tunnel: [w126] -> w65
    tunnel: [w125] -> w64
    tunnel: w63 -> [w124]
    tunnel: [w123] -> w61
    tunnel: w62 -> [w122]
    tunnel: [w121] -> w60
    stop <- w119 stop-if-true
    # "Generate USER Event Loop"
    n30 = local read "Rising Edge"() -> (w116:bool)
    n31 = Or(x="OK Button", y=w116) -> (x .or. y?=w115:bool)
    n32 = local read "TASK ENABLE"() -> (w114:bool)
    n33 = And(x=w115, y=w114) -> (x .and. y?=w113:bool)
    n34 = case shown="True" w113 {
      selector: w113 -> [_ w139]
      tunnel: w128 -> [w138 w143]
      tunnel: [w138 w142] -> w125
      tunnel: w124 -> [w137 w141]
      tunnel: [w137 w140] -> w123
      frame False {
      }
      frame True {
        n35 = Generate User Event(user event=w143, event data cluster=w139, error in=w141) -> (user event out=w142:refnum<user-event>, error out=w140:errorcluster)  [unwired: 1 in]
      }
    }
    n36 = case shown="False" "STOP" {
      selector: "STOP" -> [_ w132]
      tunnel: w127 -> [w131 w136]
      tunnel: [w131 w135] -> w126
      tunnel: w122 -> [w130 w134]
      tunnel: [w130 w133] -> w121
      tunnel: [FALSE w132] -> w119
      frame False {
      }
      frame True {
        n37 = Generate User Event(user event=w136, event data cluster=w132, error in=w134) -> (user event out=w135:refnum<user-event>, error out=w133:errorcluster)  [unwired: 1 in]
      }
    }
    n38 = Wait (ms)(milliseconds to wait=u32 10) -> ()  [unwired: 1 out]
    n39 = call "FGV Bool.vi"("Init/Read/Write State"=States_for_Action_Engine."Write", "Input Node"=w119) -> ()  [unwired: 1 in, 2 out]
  }
  n40 = while {
    tunnel: w57 -> [w150]
    tunnel: [w149] -> w56
    tunnel: w44 -> [w147]
    tunnel: [w146] -> w55
    tunnel: w50 -> [w145]
    tunnel: [w144] -> w47
    stop <- w148 stop-if-true
    # "EVENT Handling Loop"
    n41 = event shown="[1] <Start Task>: User Event" {
      selector: w150 -> [_ _ _]
      dyn-events: [_ _ _] -> w149
      timeout: _ -> [_ _ _]
      tunnel: [FALSE FALSE w181] -> w148
      tunnel: w147 -> [w155 w164 w179]
      tunnel: [w154 w163 w180] -> w146
      tunnel: w145 -> [w153 w162 w178]
      tunnel: [w152 w161 w177] -> w144
      event Timeout {
        n42 = event-data() -> ()  [unwired: 1 in, 3 out]
        n43 = Enqueue Element(queue=w155, element=Intruction_Type_Definitions."None" ("Enum"), error in (no error)=w153) -> (queue out=w154:refnum<queue>, error out=w152:errorcluster)  [unwired: 1 in, 1 out]
      }
      event User Event {
        n44 = event-data() -> ()  [unwired: 1 in, 5 out]
        n45 = call "Arduino Interfacing VI.vi"("AE Mode"=Arduino_Interfacing."Read From Arduino") -> ("Arduino Data"=w158:T4)  [unwired: 3 in, 1 out]
        n46 = Unbundle By Name(w158) -> ("Rotary Switch"=w157:u8)
        n47 = case shown="10" w157 {
          tunnel: [Intruction_Type_Definitions."None" ("Enum") Intruction_Type_Definitions."Start Task 1" ("Enum") Intruction_Type_Definitions."Start Task 2" ("Enum") Intruction_Type_Definitions."Start Task 3" ("Enum") Intruction_Type_Definitions."Start Task 4" ("Enum") Intruction_Type_Definitions."Start Task 5" ("Enum") Intruction_Type_Definitions."Start Task 6" ("Enum") Intruction_Type_Definitions."Start Task 8" ("Enum") Intruction_Type_Definitions."Start Task 9" ("Enum") Intruction_Type_Definitions."Start Task A" ("Enum")] -> w160
          frame 0, Default {
          }
          frame 1 {
          }
          frame 2 {
          }
          frame 3 {
          }
          frame 4 {
          }
          frame 5 {
          }
          frame 6 {
          }
          frame 8 {
          }
          frame 9 {
          }
          frame 10 {
          }
        }
        n48 = Enqueue Element(queue=w164, element=w160, error in (no error)=w162) -> (queue out=w163:refnum<queue>, error out=w161:errorcluster)  [unwired: 1 in, 1 out]
      }
      event User Event {
        n49 = event-data() -> ("Stop Queue"=w181:bool)  [unwired: 1 in, 4 out]
        n50 = Enqueue Element At Opposite End(queue=w179, element=Intruction_Type_Definitions."Exit" ("Enum"), error in (no error)=w178) -> (queue out=w180:refnum<queue>, error out=w177:errorcluster)  [unwired: 1 in, 1 out]
      }
    }
  }
  n51 = while {
    tunnel: w44 -> [w216]
    tunnel: w45 -> [w228]
    tunnel: w48 -> [w226]
    tunnel: [w225] -> _
    tunnel: [w224] -> w38
    shift-right: [w217] -> _
    shift-left: T16 {"PING_A"=0, "PING_B"=0, "PING_C"=0, "PING_D"=0} -> [w219]
    shift-right: [w210] -> _
    shift-left: State_Type_Definitions."Startup" ("Enum") -> [w213]
    shift-right: [w206] -> _
    shift-left: T17 {"xDistance"=0.0, "yDistance"=0.0, "wDistance"=0.0} -> [w208]
    shift-right: [w203] -> _
    shift-left: _ -> [w202]
    shift-right: [w199] -> _
    shift-left: T15 {"Recognized Object"=FALSE, "Object X coordinate"=0.0, "Object Y coordinate"=0.0} -> [w201]
    shift-right: [w196] -> _
    shift-left: T13 {"y Stepper Position"=0, "z Stepper Position"=0} -> [w198]
    shift-right: [w193] -> _
    shift-left: T12 {"Yaw"=0.0, "Compass"=0.0} -> [w195]
    shift-right: [w190] -> _
    shift-left: T11 {"Time up flag"=FALSE, "SET TIME TO CHECK"=0.0} -> [w192]
    shift-right: [w188] -> _
    shift-left: T10 {"yStepper desired"=0} -> [w189]
    shift-right: [w184] -> _
    shift-left: T9 {"Left IR Sensor"=0.0, "Arm IR Sensor"=0.0, "Bottom IR Sensor"=0.0} -> [w186]
    shift-right: [w182] -> _
    shift-left: T8 {"ySpeed"=0.0, "xSpeed"=0.0, "wSpeed"=0.0} -> [w183]
    stop <- w215 stop-if-true
    # ">>> Motor control cluster >>>"
    # ">>> yStepper command>>>"
    # ">>True Stop Next State >>"
    # ">>Error  >>"
    # ">>Timeout>>"
    # ">>Action states Queue Reference >>"
    # ">>State Logic Queue Reference >>"
    # "TOP LEVEL BASELINE (MAIN PROCESSING LOOP)"
    n52 = Dequeue Element(queue=w228, timeout in ms (-1)=0, error in (no error)=w226) -> (queue out=w220:refnum<queue>, element=w227:string, error out=w221:errorcluster)  [unwired: 1 out]
    "Action State" <- w227
    n53 = Wait (ms)(milliseconds to wait=u32 20) -> ()  [unwired: 1 out]
    n54 = case shown="\"Z STEPPER BOX HEIGHT\"" w227 {
      tunnel: [_ _ _ _ _ _ _ _ _ _ _ _ _ _ _ _ _ _ _ 0 w2245 _ _ _ _ _ _ _ _ _ _ _ _ _ _ _ _ _ _ _ _ _ _ _ _ _ _ _ _ _] -> w223
      tunnel: w220 -> [_ _ _ _ _ _ _ _ _ _ _ _ _ _ _ _ _ _ _ _ _ _ _ _ _ _ _ _ _ _ _ _ _ _ _ _ _ _ _ _ _ _ _ _ _ _ _ _ _ _]
      tunnel: w219 -> [w2000 w2009 w2021 w2032 w2049 w2060 w2071 w2083 w2096 w2108 w2119 w2126 w2141 w2155 w2167 w2177 w2189 w2215 w2225 w2236 w2246 w2255 w2265 w2295 w2306 w2314 w2323 w2333 w2345 w2358 w2367 w2376 w2393 w2401 w2414 w2421 w2431 w2441 w2451 w2458 w2473 w2480 w2496 w2502 w2514 w2526 w2538 w2550 w2562 w2573]
      tunnel: [w2000 w2009 w2021 w2032 w2049 w2060 w2071 w2083 w2096 w2108 w2119 w2126 w2141 w2156 w2167 w2177 w2189 w2216 w2225 w2236 w2246 w2255 w2265 w2294 w2306 w2314 w2323 w2333 w2345 w2358 w2367 w2376 w2393 w2401 w2414 w2421 w2431 w2441 w2451 w2458 w2473 w2480 w2496 w2502 w2514 w2526 w2538 w2550 w2562 w2573] -> w218
      tunnel: [TRUE TRUE _ _ _ _ _ _ _ _ _ _ _ _ _ _ _ _ _ _ _ _ _ _ _ _ _ _ _ _ _ _ _ _ _ _ _ _ _ _ _ _ _ _ _ _ _ _ _ _] -> w215
      tunnel: w213 -> [w1998 w2007 w2020 w2031 w2048 w2059 w2070 w2082 w2095 w2107 w2118 w2125 w2140 w2154 w2166 w2175 w2188 w2214 w2224 w2233 w2243 w2254 w2264 w2293 w2305 w2313 w2322 w2325 w2344 w2357 w2366 w2375 w2392 w2400 w2408 w2420 w2430 w2440 w2450 w2457 w2464 w2479 w2495 w2501 w2513 w2525 w2537 w2549 w2561 w2572]
      tunnel: [_ _ _ _ _ _ _ _ _ _ _ _ _ _ _ _ _ _ _ _ TRUE _ _ _ _ _ _ _ _ _ _ _ _ _ _ _ _ _ _ _ _ _ _ _ _ _ _ _ _ _] -> w212
      tunnel: [w1998 w2007 w2020 w2031 w2048 w2059 w2070 w2082 w2095 w2107 w2118 w2125 w2140 w2154 w2166 w2175 w2188 w2214 w2224 w2233 w2243 w2254 w2264 w2293 w2305 w2313 w2322 w2325 w2344 w2357 w2366 w2375 w2392 w2400 w2408 w2420 w2430 w2440 w2450 w2457 w2464 w2479 w2495 w2501 w2513 w2525 w2537 w2549 w2561 w2572] -> w211
      tunnel: w208 -> [w1997 w2006 w2019 w2034 w2047 w2058 w2069 w2081 w2094 w2106 w2117 w2127 w2139 w2153 w2168 w2179 w2190 w2213 w2226 w2232 w2242 w2256 w2266 w2283 w2304 w2316 w2324 w2330 w2346 w2359 w2368 w2377 w2394 w2403 w2412 w2423 w2433 w2443 w2453 w2460 w2468 w2482 w2498 w2504 w2516 w2528 w2540 w2552 w2564 w2575]
      tunnel: [w1997 w2006 w2019 w2034 w2047 w2058 w2069 w2081 w2094 w2106 w2117 w2127 w2138 w2153 w2168 w2179 w2190 w2212 w2226 w2232 w2242 w2256 w2266 w2282 w2304 w2316 w2324 w2330 w2346 w2359 w2368 w2377 w2394 w2403 w2412 w2423 w2433 w2443 w2453 w2460 w2468 w2482 w2498 w2504 w2516 w2528 w2540 w2552 w2564 w2575] -> w207
      tunnel: w201 -> [w1996 w2005 w2018 w2033 w2046 w2057 w2068 w2080 w2093 w2105 w2115 w2124 w2137 w2152 w2161 w2178 w2187 w2204 w2223 w2231 w2241 w2253 w2263 w2288 w2302 w2315 w2321 w2331 w2343 w2356 w2362 w2374 w2387 w2402 w2413 w2422 w2432 w2442 w2452 w2459 w2467 w2481 w2497 w2503 w2515 w2527 w2539 w2551 w2563 w2574]
      tunnel: [w1996 w2005 w2018 w2033 w2046 w2057 w2068 w2080 w2093 w2105 w2115 w2124 w2137 w2152 w2161 w2178 w2187 w2203 w2223 w2231 w2241 w2253 w2263 w2287 w2302 w2315 w2321 w2331 w2343 w2356 w2362 w2374 w2386 w2402 w2413 w2422 w2432 w2442 w2452 w2459 w2467 w2481 w2497 w2503 w2515 w2527 w2539 w2551 w2563 w2574] -> w200
      tunnel: w198 -> [w1995 w2004 w2017 w2035 w2045 w2056 w2067 w2079 w2092 w2104 w2114 w2123 w2136 w2151 w2169 w2180 w2186 w2209 w2222 w2230 w2240 w2252 w2262 w2278 w2301 w2312 w2320 w2329 w2342 w2355 w2365 w2373 w2395 w2404 w2411 w2419 w2429 w2439 w2449 w2461 w2469 w2483 w2494 w2505 w2517 w2529 w2541 w2553 w2565 w2576]
      tunnel: [w1995 w2004 w2017 w2035 w2045 w2056 w2067 w2079 w2092 w2104 w2114 w2123 w2136 w2151 w2169 w2180 w2186 w2208 w2222 w2230 w2240 w2252 w2262 w2277 w2301 w2312 w2320 w2329 w2342 w2355 w2365 w2373 w2395 w2404 w2411 w2419 w2429 w2439 w2449 w2461 w2469 w2483 w2493 w2505 w2517 w2529 w2541 w2553 w2565 w2576] -> w197
      tunnel: w195 -> [w1994 w2003 w2015 w2036 w2043 w2054 w2066 w2077 w2090 w2102 w2113 w2122 w2135 w2144 w2164 w2181 w2185 w2199 w2221 w2229 w2239 w2251 w2261 w2274 w2300 w2309 w2319 w2328 w2341 w2354 w2364 w2372 w2396 w2405 w2410 w2418 w2426 w2436 w2446 w2462 w2470 w2484 w2488 w2506 w2518 w2530 w2542 w2554 w2566 w2577]
      tunnel: [w1994 w2003 w2015 w2036 w2043 w2054 w2066 w2077 w2090 w2102 w2113 w2122 w2135 w2144 w2163 w2181 w2185 w2198 w2221 w2229 w2239 w2251 w2261 w2273 w2300 w2309 w2319 w2328 w2341 w2354 w2364 w2372 w2396 w2405 w2410 w2418 w2426 w2436 w2446 w2462 w2470 w2484 w2488 w2506 w2518 w2530 w2542 w2554 w2566 w2577] -> w194
      tunnel: w192 -> [w1992 w2002 w2016 w2037 w2044 w2055 w2065 w2078 w2091 w2103 w2112 w2121 w2134 w2143 w2160 w2182 w2184 w2195 w2218 w2228 w2238 w2250 w2260 w2271 w2298 w2308 w2318 w2327 w2340 w2353 w2363 w2371 w2397 w2406 w2409 w2417 w2425 w2435 w2445 w2463 w2471 w2485 w2487 w2500 w2512 w2524 w2536 w2548 w2560 w2571]
      tunnel: [w1992 w2002 w2016 w2037 w2044 w2055 w2065 w2078 w2091 w2103 w2112 w2121 w2134 w2143 w2160 w2182 w2184 w2195 w2218 w2228 w2238 w2250 w2260 w2270 w2298 w2308 w2318 w2327 w2340 w2353 w2363 w2371 w2397 w2406 w2409 w2417 w2425 w2435 w2445 w2463 w2471 w2485 w2487 w2500 w2510 w2522 w2534 w2546 w2558 w2570] -> w191
      tunnel: w189 -> [_ _ _ _ _ _ _ _ _ _ _ _ _ _ _ _ _ _ _ _ _ _ _ _ _ _ _ _ _ _ _ _ _ _ _ _ _ _ _ _ _ w2476 _ _ _ _ _ _ _ _]
      tunnel: [w1991 w2001 w2010 w2027 w2038 w2050 w2061 w2072 w2086 w2097 w2109 w2120 w2128 w2142 w2157 w2173 w2183 w2192 w2217 w2227 w2237 w2249 w2257 w2267 w2297 w2307 w2317 w2332 w2334 w2347 w2360 w2369 w2380 w2398 w2415 w2416 w2424 w2434 w2444 w2454 w2472 w2474 w2486 w2499 w2507 w2519 w2531 w2543 w2555 w2567] -> w185
      tunnel: w186 -> [w1991 w2001 w2010 w2027 w2038 w2050 w2061 w2072 w2086 w2097 w2109 w2120 w2128 w2142 w2157 w2174 w2183 w2192 w2217 w2227 w2237 w2249 w2257 w2267 w2297 w2307 w2317 w2332 w2334 w2347 w2360 w2369 w2380 w2398 w2415 w2416 w2424 w2434 w2444 w2454 w2472 w2474 w2486 w2499 w2507 w2519 w2531 w2543 w2555 w2567]
      tunnel: w183 -> [_ _ _ _ _ _ _ _ w2085 _ _ _ _ _ _ _ _ _ _ _ _ _ _ _ _ _ _ _ _ _ _ _ _ _ _ _ _ _ _ _ _ _ _ _ _ _ _ _ _ _]
      frame "Exit" {
        # ">>State Logic  >>"
        # ">>> Time cluster >>>"
        # ">>> Yaw >>>"
        # ">>> Stepper position >>>"
        # ">>> Encoders >>>"
        # ">>> Object detection >>>"
        # ">>> Ultrasonic Sensors Detect >>>"
        n55 = call "Imaq Dispose"("All Images? (No)"=TRUE) -> ()  [unwired: 5 in, 1 out]
      }
      frame "----Movement States----" {
        # ">>State Logic  >>"
        # ">>> Time cluster >>>"
        # ">>> Yaw >>>"
        # ">>> Stepper position >>>"
        # ">>> Encoders >>>"
        # ">>> Object detection >>>"
        # ">>> Ultrasonic Sensors Detect >>>"
      }
      frame "FORWARD" {
        # ">>State Logic  >>"
        # ">>> Time cluster >>>"
        # ">>> Yaw >>>"
        # ">>> Stepper position >>>"
        # ">>> Encoders >>>"
        # ">>> Object detection >>>"
        # ">>> Ultrasonic Sensors Detect >>>"
        n56 = Unbundle By Name(w2015) -> ("Yaw"=w2011:dbl)
        n57 = call "MOTOR CONTROL WITH PID AE.vi"("Yaw"=w2011, "Speed"=50.0, "Direction"=MOTOR_CONTROL_WITH_PID_AE_DIRECTION_TYPE_DEF."y-axis movement", "AE Mode"=MOTOR_CONTROL_WITH_PID_AE_DATA_MODE_TYPE_DEF."Write to AE") -> ()  [unwired: 1 out]
      }
      frame "FORWARD - IR ASSIST" {
        # ">>State Logic  >>"
        # ">>> Time cluster >>>"
        # ">>> Yaw >>>"
        # ">>> Stepper position >>>"
        # ">>> Encoders >>>"
        # ">>> Object detection >>>"
        # ">>> Ultrasonic Sensors Detect >>>"
        n58 = Unbundle By Name(w2027) -> ("Left IR Sensor"=w2026:dbl)
        n59 = Subtract(x=w2026, y=15.0) -> (x-y=w2024:dbl)
        n60 = Multiply(x=w2024, y=0.5) -> (x*y=w2022:dbl)
        n61 = call "MOTOR CONTROL WITH PID AE.vi"("Yaw"=w2022, "Speed"=30.0, "Direction"=MOTOR_CONTROL_WITH_PID_AE_DIRECTION_TYPE_DEF."y-axis movement", "AE Mode"=MOTOR_CONTROL_WITH_PID_AE_DATA_MODE_TYPE_DEF."Write to AE") -> ()  [unwired: 1 out]
      }
      frame "LEFT" {
        # ">>State Logic  >>"
        # ">>> Time cluster >>>"
        # ">>> Yaw >>>"
        # ">>> Stepper position >>>"
        # ">>> Encoders >>>"
        # ">>> Object detection >>>"
        # ">>> Ultrasonic Sensors Detect >>>"
        n62 = Unbundle By Name(w2043) -> ("Yaw"=w2040:dbl)
        n63 = call "MOTOR CONTROL WITH PID AE.vi"("Yaw"=w2040, "Speed"=-25.0, "Direction"=MOTOR_CONTROL_WITH_PID_AE_DIRECTION_TYPE_DEF."x-axis movement", "AE Mode"=MOTOR_CONTROL_WITH_PID_AE_DATA_MODE_TYPE_DEF."Write to AE") -> ()  [unwired: 1 out]
      }
      frame "R-ACW" {
        # ">>> IR Sensors >>>"
        # ">>> Time cluster >>>"
        # ">>> Yaw >>>"
        # ">>> Stepper position >>>"
        # ">>> Encoders >>>"
        # ">>> Object detection >>>"
        # ">>> Ultrasonic Sensors Detect >>>"
        n64 = call "MOTOR CONTROL WITH PID AE.vi"("Speed"=-10.0, "Direction"=MOTOR_CONTROL_WITH_PID_AE_DIRECTION_TYPE_DEF."rotation", "AE Mode"=MOTOR_CONTROL_WITH_PID_AE_DATA_MODE_TYPE_DEF."Write to AE") -> ()  [unwired: 1 in, 1 out]
      }
      frame "R-CW" {
        (unwired) -0.2 ("Speed")
        # ">>> Time cluster >>>"
        # ">>> Yaw >>>"
        # ">>> Stepper position >>>"
        # ">>> Encoders >>>"
        # ">>> Object detection >>>"
        # ">>> Ultrasonic Sensors Detect >>>"
        n65 = call "MOTOR CONTROL WITH PID AE.vi"("Speed"=10.0, "Direction"=MOTOR_CONTROL_WITH_PID_AE_DIRECTION_TYPE_DEF."rotation", "AE Mode"=MOTOR_CONTROL_WITH_PID_AE_DATA_MODE_TYPE_DEF."Write to AE") -> ()  [unwired: 1 in, 1 out]
      }
      frame "RIGHT" {
        # ">>> Time cluster >>>"
        # ">>> Yaw >>>"
        # ">>> Stepper position >>>"
        # ">>> Encoders >>>"
        # ">>> Object detection >>>"
        # ">>> Ultrasonic Sensors Detect >>>"
        n66 = Unbundle By Name(w2077) -> ("Yaw"=w2073:dbl)
        n67 = call "MOTOR CONTROL WITH PID AE.vi"("Yaw"=w2073, "Speed"=50.0, "Direction"=MOTOR_CONTROL_WITH_PID_AE_DIRECTION_TYPE_DEF."x-axis movement", "AE Mode"=MOTOR_CONTROL_WITH_PID_AE_DATA_MODE_TYPE_DEF."Write to AE") -> ()  [unwired: 1 out]
      }
      frame "X AXIS - SLOW" {
        # ">>> IR Sensors >>>"
        # ">>> Time cluster >>>"
        # ">>> Yaw >>>"
        # ">>> Stepper position >>>"
        # ">>> Encoders >>>"
        # ">>> Object detection >>>"
        # ">>> Ultrasonic Sensors Detect >>>"
        n68 = Unbundle By Name(w2085) -> ("xSpeed"=w2084:dbl)
        n69 = Unbundle By Name(w2090) -> ("Yaw"=w2087:dbl)
        n70 = call "MOTOR CONTROL WITH PID AE.vi"("Yaw"=w2087, "Speed"=w2084, "Direction"=MOTOR_CONTROL_WITH_PID_AE_DIRECTION_TYPE_DEF."x-axis movement", "AE Mode"=MOTOR_CONTROL_WITH_PID_AE_DATA_MODE_TYPE_DEF."Write to AE") -> ()  [unwired: 1 out]
      }
      frame "REVERSE" {
        # ">>> Time cluster >>>"
        # ">>> Yaw >>>"
        # ">>> Stepper position >>>"
        # ">>> Encoders >>>"
        # ">>> Object detection >>>"
        # ">>> Ultrasonic Sensors Detect >>>"
        n71 = Unbundle By Name(w2102) -> ("Yaw"=w2098:dbl)
        n72 = call "MOTOR CONTROL WITH PID AE.vi"("Yaw"=w2098, "Speed"=-50.0, "Direction"=MOTOR_CONTROL_WITH_PID_AE_DIRECTION_TYPE_DEF."y-axis movement", "AE Mode"=MOTOR_CONTROL_WITH_PID_AE_DATA_MODE_TYPE_DEF."Write to AE") -> ()  [unwired: 1 out]
      }
      frame "STOP" {
        n73 = Wait (ms)(milliseconds to wait=u32 100) -> ()  [unwired: 1 out]
        n74 = call "MOTOR CONTROL WITH PID AE.vi"("Direction"=MOTOR_CONTROL_WITH_PID_AE_DIRECTION_TYPE_DEF."stop", "AE Mode"=MOTOR_CONTROL_WITH_PID_AE_DATA_MODE_TYPE_DEF."Write to AE") -> ()  [unwired: 2 in, 1 out]
      }
      frame "----SENSOR READING---- " {
      }
      frame "READ ENCODERS" {
        # ">>> Time cluster >>>"
        # ">>> Yaw >>>"
        # ">>> Stepper position >>>"
        # ">>> Object detection >>>"
        # ">>> Current encoder distance >>>"
        # ">>> Ultrasonic Sensors Detect >>>"
        n75 = call "MOTOR CONTROL WITH PID AE.vi"("AE Mode"=MOTOR_CONTROL_WITH_PID_AE_DATA_MODE_TYPE_DEF."Read from AE") -> ("Speed & distance"=w2132:T1)  [unwired: 3 in]
        n76 = Unbundle By Name(w2132) -> ("xDistance"=w2131:dbl, "yDistance"=w2130:dbl, "wDistance"=w2129:dbl)
        n77 = Bundle By Name(cluster=w2139, "xDistance"=w2131, "yDistance"=w2130, "wDistance"=w2129) -> (w2138:T17)
      }
      frame "READ ULTRASONIC" {
        (unwired) navX_type_def."Read Values" ("Mode")
        (unwired) MOTOR_CONTROL_NO_PID_Type_Def."Latch" ("Direction")
        # ">>State Logic  >>"
        # ">>> Time cluster >>>"
        # ">>> Ultrasonic Sensors Detect >>>"
        # ">>> Object detection >>>"
        # ">>> Encoders >>>"
        # ">>> Stepper position >>>"
        # ">>> Yaw >>>"
        n78 = call "Arduino Interfacing VI.vi"("AE Mode"=Arduino_Interfacing."Read From Arduino") -> ("Arduino Data"=w2149:T4)  [unwired: 3 in, 1 out]
        n79 = Unbundle By Name(w2149) -> ("PING A"=w2148:u8, "PING B"=w2147:u8, "PING C"=w2146:u8, "PING D"=w2145:u8)
        n80 = Bundle By Name(cluster=w2155, "PING_A"=w2148, "PING_B"=w2147, "PING_C"=w2146, "PING_D"=w2145) -> (w2156:T16)
      }
      frame "READ NAVX" {
        # ">>> Time cluster >>>"
        # ">>> Yaw >>>"
        # ">>> Ultrasonic Sensors Detect >>>"
        # ">>> Object detection >>>"
        # ">>> Encoders >>>"
        # ">>> Stepper position >>>"
        n81 = call "navX reading VI.vi"("Mode"=navX_type_def."Read Values") -> ("NavX Readings"=w2159:T3)  [unwired: 2 in, 3 out]
        n82 = Unbundle By Name(w2159) -> ("Heading"=w2158:dbl)
        n83 = Unbundle By Name(w2159) -> ("Yaw"=w2162:dbl)
        n84 = Bundle By Name(cluster=w2164, "Yaw"=w2162, "Compass"=w2158) -> (w2163:T12)
      }
      frame "READ IR" {
        w2171 = T36 [enum."B/AI1"] items=["Not Connected", "AudioIn/Left", "AudioIn/Right", "C/AI0", "C/AI1", "A/AI0", "A/AI1", "A/AI2", "A/AI3", "A/AI4", "A/AI5", "A/AI6", "A/AI7", "B/AI0", "B/AI1", "B/AI2", "B/AI3", "B/AI4", "B/AI5", "B/AI6", "B/AI7", "AI/AI0", "AI/AI1", "AI/AI2", "AI/AI3", "A/AI0 (DIFF)", "A/AI1 (DIFF)", "A/AI2 (DIFF)", "A/AI3 (DIFF)", "B/AI0 (DIFF)", "B/AI1 (DIFF)", "B/AI2 (DIFF)", "B/AI3 (DIFF)"] ("AI Channel")
        w2176 = T36 [enum."B/AI0"] items=["Not Connected", "AudioIn/Left", "AudioIn/Right", "C/AI0", "C/AI1", "A/AI0", "A/AI1", "A/AI2", "A/AI3", "A/AI4", "A/AI5", "A/AI6", "A/AI7", "B/AI0", "B/AI1", "B/AI2", "B/AI3", "B/AI4", "B/AI5", "B/AI6", "B/AI7", "AI/AI0", "AI/AI1", "AI/AI2", "AI/AI3", "A/AI0 (DIFF)", "A/AI1 (DIFF)", "A/AI2 (DIFF)", "A/AI3 (DIFF)", "B/AI0 (DIFF)", "B/AI1 (DIFF)", "B/AI2 (DIFF)", "B/AI3 (DIFF)"] ("AI Channel")
        # ">>State Logic  >>"
        # ">>> Time cluster >>>"
        # ">>> Ultrasonic Sensors Detect >>>"
        # ">>> Object detection >>>"
        # ">>> Encoders >>>"
        # ">>> Stepper position >>>"
        # ">>> Yaw >>>"
        n85 = call <vilib>:"Sharp IR.vi"("AI Channel"=w2176) -> ("Sharp IR Distance"=w2172:dbl)  [unwired: 8 in, 2 out]
        n86 = call <vilib>:"Sharp IR.vi"("AI Channel"=w2171) -> ("Sharp IR Distance"=w2170:dbl)  [unwired: 8 in, 2 out]
        n87 = Bundle By Name(cluster=w2174, "Left IR Sensor"=w2172, "Arm IR Sensor"=w2170) -> (w2173:T9)
      }
      frame "----SYSTEM MODES----" {
        (unwired) I2C_MASTER_Type_Def."Last State" ("Arduino Mode")
        # ">>> Object detection >>>"
        # ">>> Yaw >>>"
        # ">>> Ultrasonic Sensors Detect >>>"
        # ">>> Encoders >>>"
        # ">>> Stepper position >>>"
      }
      frame "INIT" {
        w2210 = u8 0
        w2211 = 0.0
        # ">>> Time cluster >>>"
        # ">>> Object detection >>>"
        # ">>> Yaw >>>"
        # ">>> Ultrasonic Sensors Detect >>>"
        # ">>> Encoders >>>"
        # ">>> Stepper position >>>"
        # ">>State Logic  >>"
        n88 = call "Arduino Interfacing VI.vi"("AE Mode"=Arduino_Interfacing."Initialize") -> ()  [unwired: 3 in, 2 out]
        n89 = call "FGV Bool.vi"("Init/Read/Write State"=States_for_Action_Engine."Initialize") -> ()  [unwired: 2 in, 2 out]
        n90 = call "Elasped Timer.vi"("Action"=Elapsed_timer_control."Initialize") -> ()  [unwired: 7 in, 4 out]
        n91 = call "MOTOR CONTROL WITH PID AE.vi"("AE Mode"=MOTOR_CONTROL_WITH_PID_AE_DATA_MODE_TYPE_DEF."Init AE") -> ()  [unwired: 3 in, 1 out]
        n92 = call "IMAQ Reference AE.vi"("IMAQ AE States"=IMAQ_Reference_AE."Initialize AE") -> ()  [unwired: 1 in, 2 out]
        n93 = Bundle By Name(cluster=w2204, "Recognized Object"=FALSE, "Object X coordinate"=0.0, "Object Y coordinate"=0.0) -> (w2203:T15)
        n94 = Bundle By Name(cluster=w2209, "y Stepper Position"=u8 0, "z Stepper Position"=u8 0) -> (w2208:T13)
        n95 = Bundle By Name(cluster=w2213, "xDistance"=w2211, "yDistance"=w2211, "wDistance"=w2211) -> (w2212:T17)
        n96 = Bundle By Name(cluster=w2215, "PING_A"=w2210, "PING_B"=w2210, "PING_C"=w2210, "PING_D"=w2210) -> (w2216:T16)
        n97 = Bundle By Name(cluster=w2199, "Yaw"=0.0) -> (w2198:T12)
      }
      frame "ARDUINO - ULTRASONIC" {
        # ">>> Object detection >>>"
        # ">>> Yaw >>>"
        # ">>> Ultrasonic Sensors Detect >>>"
        # ">>> Encoders >>>"
        # ">>> Stepper position >>>"
        # ">>State Logic  >>"
        n98 = call "Arduino Interfacing VI.vi"("Data to Write"=I2C_MASTER_WRITE_NEW_Type_Def."Ultrasonic sensors", "AE Mode"=Arduino_Interfacing."Write to Arduino") -> ()  [unwired: 2 in, 2 out]
      }
      frame "NAVX CALIBRATE" {
        # ">>> Object detection >>>"
        # ">>> Yaw >>>"
        # ">>> Ultrasonic Sensors Detect >>>"
        # ">>> Encoders >>>"
        # ">>> Stepper position >>>"
        # ">>State Logic  >>"
        # "Adds a 15 second delay to the startup process \nfor the NavX to calibrate"
        n99 = Wait (ms)(milliseconds to wait=u32 1000) -> ()  [unwired: 1 out]
      }
      frame "NO ACTION", Default {
        (unwired) u8 0 ("y Stepper value")
        (unwired) TRUE ("Latch")
        (unwired) navX_type_def."Read Values" ("Mode")
        (unwired) MOTOR_CONTROL_NO_PID_Type_Def."Latch" ("Direction")
        # ">>> Object detection >>>"
        # ">>> Yaw >>>"
        # ">>> Ultrasonic Sensors Detect >>>"
        # ">>> Encoders >>>"
        # ">>> Stepper position >>>"
        # ">>State Logic  >>"
        n100 = case shown="4" w2243 {
          tunnel: [0 100] -> w2245
          frame 1, Default {
          }
          frame 4 {
          }
        }
      }
      frame "----RESET CASES----" {
        (unwired) I2C_MASTER_Type_Def."Last State" ("Arduino Mode")
        # ">>> Object detection >>>"
        # ">>> Yaw >>>"
        # ">>> Ultrasonic Sensors Detect >>>"
        # ">>> Encoders >>>"
        # ">>> Stepper position >>>"
        # ">>State Logic  >>"
      }
      frame "RESET ENCODERS" {
        # ">>> Object detection >>>"
        # ">>> Yaw >>>"
        # ">>> Ultrasonic Sensors Detect >>>"
        # ">>> Encoders >>>"
        # ">>> Stepper position >>>"
        # ">>State Logic  >>"
        n101 = call "MOTOR CONTROL WITH PID AE.vi"("Direction"=MOTOR_CONTROL_WITH_PID_AE_DIRECTION_TYPE_DEF."reset encoders", "AE Mode"=MOTOR_CONTROL_WITH_PID_AE_DATA_MODE_TYPE_DEF."Write to AE") -> ()  [unwired: 2 in, 1 out]
      }
      frame "RESET FLAGS" {
        (unwired) I2C_MASTER_Type_Def."Last State" ("Arduino Mode")
        # "Resets any software variables\nand/or non-critical states"
        n102 = Wait (ms)(milliseconds to wait=u32 20) -> ()  [unwired: 1 out]
        n103 = Bundle By Name(cluster=w2271, "Time up flag"=FALSE, "SET TIME TO CHECK"=0.0) -> (w2270:T11)
        n104 = Bundle By Name(cluster=w2288, "Recognized Object"=FALSE, "Object X coordinate"=0.0, "Object Y coordinate"=0.0) -> (w2287:T15)
        n105 = Bundle By Name(cluster=w2278, "y Stepper Position"=u8 0, "z Stepper Position"=u8 0) -> (w2277:T13)
        n106 = Bundle By Name(cluster=w2283, "xDistance"=0.0, "yDistance"=0.0, "wDistance"=0.0) -> (w2282:T17)
        n107 = Bundle By Name(cluster=w2295, "PING_A"=u8 0, "PING_B"=u8 0, "PING_C"=u8 0, "PING_D"=u8 0) -> (w2294:T16)
        n108 = Bundle By Name(cluster=w2274, "Yaw"=0.0) -> (w2273:T12)
      }
      frame "RESET YAW" {
        n109 = Wait (ms)(milliseconds to wait=u32 100) -> ()  [unwired: 1 out]
        n110 = call "navX reading VI.vi"("Mode"=navX_type_def."Zero Yaw") -> ()  [unwired: 2 in, 4 out]
      }
      frame "RESET ARM" {
        n111 = call "Arduino Interfacing VI.vi"("Data to Write"=I2C_MASTER_WRITE_NEW_Type_Def."Soft Reset", "AE Mode"=Arduino_Interfacing."Write to Arduino") -> ()  [unwired: 2 in, 2 out]
      }
      frame "--------CAM STATES-------" {
      }
      frame "OPEN IMAQ REF" {
        # ">>State Logic  >>"
        # ">>> Time cluster >>>"
        # ">>> Object detection >>>"
        # ">>> Yaw >>>"
        # ">>> Ultrasonic Sensors Detect >>>"
        # ">>> Encoders >>>"
        # ">>> Stepper position >>>"
        # ">>> IR Sensors >>>"
        n112 = call "IMAQ Reference AE.vi"("IMAQ AE States"=IMAQ_Reference_AE."Initialize AE") -> ()  [unwired: 1 in, 2 out]
      }
      frame "OPEN LOG CAM" {
        n113 = call "Webcam AE.vi"("Session In"=T32 "cam0", "Camera states"=Webcam_AE."Initialize Camera") -> ("error out"=w2337:errorcluster, "Session Out"=w2336:T32)  [unwired: 1 in, 1 out]
        n114 = call "Webcam AE.vi"("error in (no error)"=w2337, "Session In"=w2336, "Camera states"=Webcam_AE."Open Camera") -> ()  [unwired: 3 out]
      }
      frame "OPEN LIFE CAM" {
        n115 = call "Webcam AE.vi"("Session In"=T32 "cam1", "Camera states"=Webcam_AE."Initialize Camera") -> ("error out"=w2350:errorcluster, "Session Out"=w2349:T32)  [unwired: 1 in, 1 out]
        n116 = call "Webcam AE.vi"("error in (no error)"=w2350, "Session In"=w2349, "Camera states"=Webcam_AE."Open Camera") -> ()  [unwired: 3 out]
      }
      frame "CAM ACQ" {
        # ">>State Logic  >>"
        # ">>> Time cluster >>>"
        # ">>> Yaw >>>"
        # ">>> Stepper position >>>"
        # ">>> Encoders >>>"
        # ">>> Object detection >>>"
        # ">>> Ultrasonic Sensors Detect >>>"
        n117 = call "Webcam AE.vi"("Camera states"=Webcam_AE."Continuous Acquisition") -> ()  [unwired: 2 in, 3 out]
      }
      frame "CAM CLOSE" {
        # ">>State Logic  >>"
        # ">>> Time cluster >>>"
        # ">>> Yaw >>>"
        # ">>> Stepper position >>>"
        # ">>> Encoders >>>"
        # ">>> Object detection >>>"
        # ">>> Ultrasonic Sensors Detect >>>"
        n118 = call "Webcam AE.vi"("Camera states"=Webcam_AE."Close Camera") -> ()  [unwired: 2 in, 3 out]
      }
      frame "PROCESS IMAGE" {
        # ">>State Logic  >>"
        # ">>> Time cluster >>>"
        # ">>> Yaw >>>"
        # ">>> Stepper position >>>"
        # ">>> Encoders >>>"
        # ">>> Object detection >>>"
        # ">>> Ultrasonic Sensors Detect >>>"
        n119 = call "Webcam AE.vi"("Camera states"=Webcam_AE."Retrieve Image") -> ("error out"=w2388:errorcluster, "Image Out"=w2390:T39)  [unwired: 2 in, 1 out]
        n120 = call "IMAQ Reference AE.vi"("IMAQ AE States"=IMAQ_Reference_AE."Get IMAQ Reference") -> ("Image Out"=w2378:T39)  [unwired: 1 in, 1 out]
        n121 = call "Object Detection SubVI.vi"("Error In"=w2388, "Mode"="Object recognition mode", "Image Dest"=w2378, "Image in"=w2390) -> ("Object Center Coordinates"=w2385:cluster{"x":sgl, "y":sgl}, "Object detection cluster"=w2381:T2)  [unwired: 2 out]
        "Object detection cluster" <- w2381
        "Object Center Coordinates" <- w2385
        n122 = Unbundle By Name(w2381) -> ("Object detected?"=w2382:bool)
        n123 = Unbundle By Name(w2385) -> ("x"=w2384:sgl, "y"=w2383:sgl)
        n124 = Bundle By Name(cluster=w2387, "Recognized Object"=w2382, "Object X coordinate"=w2384, "Object Y coordinate"=w2383) -> (w2386:T15)
      }
      frame "DISPOSE BUFFERS" {
        # ">>> IR Sensors >>>"
        # ">>State Logic  >>"
        # ">>> Time cluster >>>"
        # ">>> Yaw >>>"
        # ">>> Stepper position >>>"
        # ">>> Encoders >>>"
        # ">>> Object detection >>>"
        # ">>> Ultrasonic Sensors Detect >>>"
        n125 = call "Webcam AE.vi"("Camera states"=Webcam_AE."Dispose Image Buffers") -> ()  [unwired: 2 in, 3 out]
      }
      frame "DISPOSE ALL BUFFERS" {
        # ">>State Logic  >>"
        # ">>> IR Sensors >>>"
        # ">>> Time cluster >>>"
        # ">>> Object detection >>>"
        # ">>> Yaw >>>"
        # ">>> Ultrasonic Sensors Detect >>>"
        # ">>> Encoders >>>"
        # ">>> Stepper position >>>"
        n126 = call "IMAQ Reference AE.vi"("IMAQ AE States"=IMAQ_Reference_AE."Destroy ALL IMAQ") -> ()  [unwired: 1 in, 2 out]
      }
      frame "-----ARM ACTIONS-----" {
      }
      frame "CLOSE CLAW" {
        n127 = call "Arduino Interfacing VI.vi"("Data to Write"=I2C_MASTER_WRITE_NEW_Type_Def."Close Claw", "AE Mode"=Arduino_Interfacing."Write to Arduino") -> ()  [unwired: 2 in, 2 out]
      }
      frame "OPEN CLAW" {
        n128 = call "Arduino Interfacing VI.vi"("Data to Write"=I2C_MASTER_WRITE_NEW_Type_Def."Open Claw", "AE Mode"=Arduino_Interfacing."Write to Arduino") -> ()  [unwired: 2 in, 2 out]
      }
      frame "Z STEPPER CAM HEIGHT" {
        n129 = call "Arduino Interfacing VI.vi"("Data to Write"=I2C_MASTER_WRITE_NEW_Type_Def."zStepper 6k", "AE Mode"=Arduino_Interfacing."Write to Arduino") -> ()  [unwired: 2 in, 2 out]
      }
      frame "Z STEPPER GRAB HEIGHT" {
        # ">>State Logic  >>"
        # ">>> Time cluster >>>"
        # ">>> Yaw >>>"
        # ">>> Stepper position >>>"
        # ">>> Encoders >>>"
        # ">>> Object detection >>>"
        # ">>> Ultrasonic Sensors Detect >>>"
        n130 = call "Arduino Interfacing VI.vi"("Data to Write"=I2C_MASTER_WRITE_NEW_Type_Def."zStepper 100", "AE Mode"=Arduino_Interfacing."Write to Arduino") -> ()  [unwired: 2 in, 2 out]
      }
      frame "Z STEPPER BOX HEIGHT" {
        # ">>> IR Sensors >>>"
        # ">>> Time cluster >>>"
        # ">>> Yaw >>>"
        # ">>> Stepper position >>>"
        # ">>> Encoders >>>"
        # ">>> Object detection >>>"
        # ">>> Ultrasonic Sensors Detect >>>"
        n131 = call "Arduino Interfacing VI.vi"("Data to Write"=I2C_MASTER_WRITE_NEW_Type_Def."zStepper 4k", "AE Mode"=Arduino_Interfacing."Write to Arduino") -> ()  [unwired: 2 in, 2 out]
      }
      frame "Y STEPPER CONTROL" {
        # ">>State Logic  >>"
        # ">>> yStepper command>>>"
        # ">>> Time cluster >>>"
        # ">>> Yaw >>>"
        # ">>> Stepper position >>>"
        # ">>> Encoders >>>"
        # ">>> Object detection >>>"
        # ">>> Ultrasonic Sensors Detect >>>"
        n132 = Unbundle By Name(w2476) -> ("yStepper desired"=w2475:u8)
        n133 = call "Arduino Interfacing VI.vi"("y Stepper value"=w2475, "Data to Write"=I2C_MASTER_WRITE_NEW_Type_Def."yStepper control", "AE Mode"=Arduino_Interfacing."Write to Arduino") -> ()  [unwired: 1 in, 2 out]
      }
      frame "READ STEPPER VALUES" {
        # ">>State Logic  >>"
        # ">>> Time cluster >>>"
        # ">>> Yaw >>>"
        # ">>> Stepper position >>>"
        # ">>> Encoders >>>"
        # ">>> Object detection >>>"
        # ">>> Ultrasonic Sensors Detect >>>"
        n134 = call "Arduino Interfacing VI.vi"("AE Mode"=Arduino_Interfacing."Read From Arduino") -> ("Arduino Data"=w2491:T4)  [unwired: 3 in, 1 out]
        n135 = Unbundle By Name(w2491) -> ("y Stepper Position"=w2490:u8, "z Stepper Position"=w2489:u8)
        n136 = Bundle By Name(cluster=w2494, "y Stepper Position"=w2490, "z Stepper Position"=w2489) -> (w2493:T13)
      }
      frame " -----TIMING-----" {
        # ">>State Logic  >>"
        # ">>> Time cluster >>>"
        # ">>> Yaw >>>"
        # ">>> Stepper position >>>"
        # ">>> Encoders >>>"
        # ">>> Object detection >>>"
        # ">>> Ultrasonic Sensors Detect >>>"
      }
      frame "SET TIMER 1" {
        # ">>State Logic  >>"
        # ">>> Time cluster >>>"
        # ">>> Yaw >>>"
        # ">>> Stepper position >>>"
        # ">>> Encoders >>>"
        # ">>> Object detection >>>"
        # ">>> Ultrasonic Sensors Detect >>>"
        n137 = call "Elasped Timer.vi"("Time Setting"=1.0, "Action"=Elapsed_timer_control."Initialize") -> ()  [unwired: 6 in, 4 out]
        n138 = Bundle By Name(cluster=w2512, "Time up flag"=FALSE) -> (w2510:T11)
      }
      frame "SET TIMER 2" {
        # ">>State Logic  >>"
        # ">>> Time cluster >>>"
        # ">>> Yaw >>>"
        # ">>> Stepper position >>>"
        # ">>> Encoders >>>"
        # ">>> Object detection >>>"
        # ">>> Ultrasonic Sensors Detect >>>"
        n139 = call "Elasped Timer.vi"("Time Setting"=2.0, "Action"=Elapsed_timer_control."Initialize") -> ()  [unwired: 6 in, 4 out]
        n140 = Bundle By Name(cluster=w2524, "Time up flag"=FALSE) -> (w2522:T11)
      }
      frame "SET TIMER 3" {
        # ">>State Logic  >>"
        # ">>> Time cluster >>>"
        # ">>> Yaw >>>"
        # ">>> Stepper position >>>"
        # ">>> Encoders >>>"
        # ">>> Object detection >>>"
        # ">>> Ultrasonic Sensors Detect >>>"
        n141 = call "Elasped Timer.vi"("Time Setting"=3.0, "Action"=Elapsed_timer_control."Initialize") -> ()  [unwired: 6 in, 4 out]
        n142 = Bundle By Name(cluster=w2536, "Time up flag"=FALSE) -> (w2534:T11)
      }
      frame "SET TIMER 4" {
        # ">>State Logic  >>"
        # ">>> Time cluster >>>"
        # ">>> Yaw >>>"
        # ">>> Stepper position >>>"
        # ">>> Encoders >>>"
        # ">>> Object detection >>>"
        # ">>> Ultrasonic Sensors Detect >>>"
        n143 = call "Elasped Timer.vi"("Time Setting"=4.0, "Action"=Elapsed_timer_control."Initialize") -> ()  [unwired: 6 in, 4 out]
        n144 = Bundle By Name(cluster=w2548, "Time up flag"=FALSE) -> (w2546:T11)
      }
      frame "SET TIMER 5" {
        # ">>State Logic  >>"
        # ">>> Time cluster >>>"
        # ">>> Yaw >>>"
        # ">>> Stepper position >>>"
        # ">>> Encoders >>>"
        # ">>> Object detection >>>"
        # ">>> Ultrasonic Sensors Detect >>>"
        n145 = call "Elasped Timer.vi"("Time Setting"=5.0, "Action"=Elapsed_timer_control."Initialize") -> ()  [unwired: 6 in, 4 out]
        n146 = Bundle By Name(cluster=w2560, "Time up flag"=FALSE) -> (w2558:T11)
      }
      frame "START TIMER" {
        # ">>State Logic  >>"
        # ">>> Time cluster >>>"
        # ">>> Yaw >>>"
        # ">>> Stepper position >>>"
        # ">>> Encoders >>>"
        # ">>> Object detection >>>"
        # ">>> Ultrasonic Sensors Detect >>>"
        n147 = call "Elasped Timer.vi"("Action"=Elapsed_timer_control."Start") -> ("Time Out?!"=w2568:bool)  [unwired: 7 in, 3 out]
        n148 = Bundle By Name(cluster=w2571, "Time up flag"=w2568) -> (w2570:T11)
      }
    }
    "State Logic" <- w211
    n149 = local read "TASK ENABLE"() -> (w205:bool)
    n150 = Not(x=w205) -> (.not. x?=w204:bool)
    n151 = case shown="True" w212 {
      tunnel: w216 -> [w241 w277]
      tunnel: w220 -> [w237 w279]
      tunnel: [w241 w277] -> w225
      tunnel: [w237 w280] -> w224
      tunnel: w221 -> [_ w275]
      tunnel: w223 -> [_ w276]
      tunnel: w218 -> [w240 w282]
      tunnel: [w240 w282] -> w217
      tunnel: "STOP TASK" -> [_ w265]
      tunnel: w211 -> [w239 w281]
      tunnel: [w239 w278] -> w210
      tunnel: w207 -> [w238 w271]
      tunnel: [w238 w271] -> w206
      tunnel: w204 -> [_ w266]
      tunnel: [w236 w263] -> w203
      tunnel: w202 -> [w236 w262]
      tunnel: w200 -> [w235 w259]
      tunnel: [w235 w259] -> w199
      tunnel: w197 -> [w234 w255]
      tunnel: [w234 w255] -> w196
      tunnel: w194 -> [w233 w253]
      tunnel: [w233 w253] -> w193
      tunnel: w191 -> [w232 w251]
      tunnel: [w232 w251] -> w190
      tunnel: w189 -> [w231 w250]
      tunnel: [w231 w249] -> w188
      tunnel: [_ w247] -> w187
      tunnel: w185 -> [w230 w245]
      tunnel: [w230 w245] -> w184
      tunnel: w183 -> [w229 w244]
      tunnel: [w229 w243] -> w182
      frame False {
        # ">>> Motor control cluster >>>"
        # ">>> yStepper command>>>"
        # ">>> Motor control cluster >>>"
        # ">>> yStepper command>>>"
        # ">>> Motor control cluster >>>"
        # ">>> IR Sensors >>>"
        # ">>> IR Sensors >>>"
        # ">>> yStepper command>>>"
        # ">>> Time cluster >>>"
        # ">>> Yaw >>>"
        # ">>> Stepper position >>>"
        # ">>> Encoders >>>"
        # ">>> Object detection >>>"
        # ">>> Ultrasonic Sensors Detect >>>"
        # ">>> Time cluster >>>"
        # ">>> Yaw >>>"
        # ">>> Stepper position >>>"
        # ">>> Encoders >>>"
        # ">>> Object detection >>>"
        # ">>> Ultrasonic Sensors Detect >>>"
      }
      frame True {
        # ">>> Motor control cluster >>>"
        # ">>> yStepper command>>>"
        # ">>> IR Sensors >>>"
        # ">>> Motor control cluster >>>"
        # ">>State Logic Queue Reference >>"
        # ">>Timeout>>"
        # ">>> yStepper command>>>"
        # ">>> Time cluster >>>"
        # ">>> Object detection >>>"
        # ">>> Yaw >>>"
        # ">>> Ultrasonic Sensors Detect >>>"
        # ">>> Encoders >>>"
        # ">>> Stepper position >>>"
        # ">>State Logic  >>"
        # ">>True Stop Next State >>"
        # ">>Action Queue>>"
        # ">> Manual override >>"
        # ">>> Time cluster >>>"
        # ">>> Yaw >>>"
        # ">>> Stepper position >>>"
        # ">>> Encoders >>>"
        # ">>> Object detection >>>"
        # ">>> Ultrasonic Sensors Detect >>>"
        # ">>Action Queue>>"
        # ">>State Logic Queue Reference >>"
        n152 = Or(x=w265, y=w266) -> (x .or. y?=w264:bool)
        n153 = Unbundle By Name(w245) -> ("Left IR Sensor"=w246:dbl, "Arm IR Sensor"=w242:dbl)
        "Left IR Sensor" <- w246
        "Arm IR Sensor" <- w242
        n154 = Unbundle By Name(w251) -> ("Time up flag"=w252:bool)
        "Time up flag" <- w252
        n155 = Unbundle By Name(w253) -> ("Yaw"=w254:dbl, "Compass"=w248:dbl)
        n156 = Unbundle By Name(w255) -> ("y Stepper Position"=w257:u8, "z Stepper Position"=w256:u8)
        n157 = Unbundle By Name(w271) -> ("xDistance"=w268:dbl, "yDistance"=w269:dbl, "wDistance"=w270:dbl)
        n158 = Unbundle By Name(w259) -> ("Recognized Object"=w258:bool, "Object X coordinate"=w261:dbl, "Object Y coordinate"=w260:dbl)
        n159 = Unbundle By Name(w282) -> ("PING_A"=w274:u8, "PING_B"=w273:u8, "PING_C"=w272:u8, "PING_D"=w267:u8)
        n160 = case shown="41" w281 {
          tunnel: [w286 w297 w310 w320 w402 w416 w452 w505 w547 w594 w637 w691 w738 w778 w838 w883 w923 w971 w1013 w1065 w1102 w1153 w1196 w1239 w1268 w1285 w1330 w1370 w1418 w1470 w1508 w1556 w1598 w1650 w1687 w1738 w1773 w1821 w1862 w1903 w1957] -> w280
          tunnel: w279 -> [w286 w300 w311 w323 w404 w417 w461 w503 w551 w595 w643 w684 w741 w785 w828 w886 w929 w970 w1016 w1055 w1108 w1143 w1191 w1230 w1268 w1275 w1333 w1376 w1417 w1469 w1514 w1555 w1601 w1640 w1693 w1728 w1777 w1828 w1867 w1907 w1955]
          tunnel: [State_Type_Definitions."Idle" ("Enum") State_Type_Definitions."Idle" ("Enum") w306 w322 State_Type_Definitions."Shutdown" ("Enum") w418 w459 w506 w548 w593 w638 w690 w739 w780 w837 w884 w930 w972 w1015 w1064 w1109 w1152 w1197 w1231 State_Type_Definitions."Idle" ("Enum") w1284 w1331 w1377 w1419 w1471 w1515 w1557 w1600 w1649 w1694 w1737 w1774 w1822 w1863 w1904 w1958] -> w278
          tunnel: w277 -> [_ _ w309 w326 _ w423 w455 w502 w552 w602 w642 w688 w742 w784 w835 w881 w928 w968 w1017 w1062 w1107 w1150 w1194 w1238 _ w1282 w1328 w1375 w1415 w1467 w1513 w1553 w1602 w1647 w1692 w1735 w1781 w1827 w1870 w1911 w1954]
          tunnel: w276 -> [_ _ _ w325 _ w422 w454 w501 w553 w601 w641 w687 w735 w783 w834 w880 w927 w967 w1018 w1061 w1106 w1149 w1193 w1236 _ w1281 w1327 w1374 w1414 w1466 w1512 w1552 w1603 w1646 w1691 w1734 w1776 w1826 w1869 w1906 w1953]
          tunnel: w275 -> [_ _ w308 w321 _ w421 w453 w500 w554 w600 w640 w686 w734 w782 w836 w882 w926 w966 w1019 w1063 w1105 w1151 w1192 w1237 _ w1283 w1329 w1373 w1413 w1465 w1511 w1551 w1604 w1648 w1690 w1736 w1780 w1825 w1868 w1910 w1952]
          tunnel: w264 -> [_ _ _ _ _ w415 w460 w499 w555 w597 w636 w689 w740 w786 w829 w887 w924 w969 w1020 w1056 w1103 w1144 w1195 w1234 _ w1276 w1334 w1371 w1416 w1468 w1509 w1554 w1605 w1641 w1688 w1729 w1779 w1820 w1866 w1909 w1951]
          tunnel: w274 -> [_ _ _ _ _ _ _ _ _ _ _ _ _ _ _ _ _ _ _ _ _ _ _ _ _ _ _ _ _ _ _ _ _ _ _ _ _ _ _ _ _]
          tunnel: w273 -> [_ _ _ _ _ _ _ w498 _ _ _ w680 w723 w776 _ w873 _ _ _ _ _ _ _ _ _ _ w1320 _ _ _ _ _ _ _ _ _ _ _ _ _ _]
          tunnel: w272 -> [_ _ _ _ _ _ _ w497 _ _ _ w681 w724 w777 _ w874 _ _ _ _ _ _ _ _ _ _ w1321 _ _ _ _ _ _ _ _ _ _ _ _ _ _]
          tunnel: w270 -> [_ _ _ _ _ _ _ _ _ w599 _ _ _ _ _ _ _ _ _ _ _ _ _ _ _ _ _ _ _ _ _ _ _ _ _ _ _ _ _ _ _]
          tunnel: w269 -> [_ _ _ _ _ w414 _ _ w546 _ _ _ _ w781 _ _ _ _ _ _ _ _ _ _ _ _ _ _ _ _ _ _ _ _ _ _ _ _ _ _ _]
          tunnel: w268 -> [_ _ _ _ _ _ _ _ _ _ _ _ w729 _ _ _ _ _ _ _ _ _ _ _ _ _ _ _ _ w1456 _ _ _ _ _ _ _ _ _ _ _]
          tunnel: w267 -> [_ _ _ _ _ _ _ _ _ _ _ _ _ _ _ _ _ _ _ _ _ _ _ _ _ _ _ _ _ _ _ _ _ _ _ _ _ _ _ _ _]
          tunnel: [State_Type_Definitions."Idle" ("Enum") State_Type_Definitions."Idle" ("Enum") State_Type_Definitions."Idle" ("Enum") State_Type_Definitions."Idle" ("Enum") State_Type_Definitions."Shutdown" ("Enum") w411 w458 w504 w549 w590 w635 w683 w737 w779 w839 w885 w922 w973 w1014 w1066 w1101 w1154 w1198 w1232 w1270 w1286 w1332 w1369 w1420 w1472 w1507 w1558 w1599 w1651 w1686 w1739 w1775 w1823 w1865 w1905 w1956] -> w263
          tunnel: w262 -> [_ _ w306 _ _ _ _ _ _ _ _ _ _ _ _ _ _ _ _ _ _ _ _ _ w1270 _ _ _ _ _ _ _ _ _ _ _ _ _ _ _ _]
          tunnel: w258 -> [_ _ _ _ _ _ _ _ _ _ _ _ _ _ _ _ _ _ _ _ _ _ _ w1233 _ _ _ _ _ _ _ _ _ _ _ _ _ _ _ _ _]
          tunnel: w261 -> [_ _ _ _ _ _ _ _ _ _ _ _ _ _ _ _ _ _ _ _ _ _ _ _ _ _ _ _ _ w1462 _ _ _ _ _ _ _ _ _ _ _]
          tunnel: w260 -> [_ _ _ _ _ _ _ _ _ _ _ _ _ _ _ _ _ _ w1009 _ _ _ _ _ _ _ _ _ _ _ _ _ w1594 _ _ _ _ _ _ _ _]
          tunnel: w257 -> [_ _ _ _ _ _ _ _ _ _ _ _ _ _ _ _ _ _ w1008 _ _ _ _ _ _ _ _ _ _ _ _ _ w1593 _ _ _ _ _ _ _ _]
          tunnel: w256 -> [_ _ _ _ _ _ w457 _ _ _ w633 _ _ _ w832 _ _ _ _ w1059 _ w1147 w1190 _ _ w1279 _ _ _ _ _ _ _ w1644 _ w1732 w1778 _ _ w1908 _]
          tunnel: w254 -> [_ _ _ _ _ _ _ _ _ _ _ _ _ _ _ _ _ _ _ _ _ _ _ _ _ _ _ _ _ _ _ _ _ _ _ _ _ _ _ _ _]
          tunnel: w252 -> [_ _ _ _ _ _ _ _ _ _ _ _ _ _ _ _ w920 w963 _ _ w1099 _ _ _ _ _ _ w1367 w1410 _ w1505 w1548 _ _ w1684 _ _ _ _ _ _]
          tunnel: w250 -> [w284 w295 w305 w318 w400 w410 w456 w496 w550 w589 w634 w682 w733 w775 w827 w878 w921 w964 w1011 w1054 w1100 w1142 w1187 w1229 w1271 w1274 w1325 w1368 w1411 w1463 w1506 w1549 w1596 w1639 w1685 w1727 w1772 w1824 w1864 w1902 w1950]
          tunnel: [w284 w294 w305 w318 w400 w410 w456 w496 w550 w589 w634 w682 w733 w775 w827 w878 w921 w964 w1010 w1054 w1100 w1142 w1187 w1229 w1271 w1274 w1325 w1368 w1411 w1463 w1506 w1549 w1595 w1639 w1685 w1727 w1772 w1824 w1864 w1902 w1950] -> w249
          tunnel: w248 -> [_ _ _ _ _ _ _ _ _ _ _ _ _ _ _ _ _ _ _ _ _ _ _ _ _ _ _ _ _ _ _ _ _ _ _ _ _ w1819 _ _ _]
          tunnel: [_ _ _ TRUE _ _ _ _ _ _ _ _ _ _ _ _ _ _ _ _ _ _ _ _ _ _ _ _ _ _ _ _ _ _ _ _ _ _ _ _ _] -> w247
          tunnel: w246 -> [_ _ _ _ _ _ _ _ _ _ _ _ _ _ _ _ _ _ _ _ _ _ _ _ _ _ _ _ _ _ _ _ _ _ _ _ _ _ _ _ _]
          tunnel: w244 -> [w283 w292 w304 w316 w399 w409 w451 w495 w543 w588 w630 w675 w722 w774 w826 w871 w919 w962 w1005 w1053 w1098 w1141 w1186 w1228 w1272 w1273 w1318 w1366 w1409 w1459 w1504 w1547 w1590 w1638 w1683 w1726 w1771 w1815 w1861 w1901 w1949]
          tunnel: [w283 w291 w304 w316 w399 w409 w451 w495 w543 w588 w630 w675 w722 w774 w826 w871 w919 w962 w1005 w1053 w1098 w1141 w1186 w1228 w1272 w1273 w1318 w1366 w1409 w1458 w1504 w1547 w1590 w1638 w1683 w1726 w1771 w1815 w1861 w1901 w1949] -> w243
          tunnel: w242 -> [_ _ _ _ _ _ _ _ _ _ _ _ _ _ _ _ _ _ _ _ _ _ _ _ _ _ _ _ _ _ _ _ _ _ _ _ _ _ _ _ w1948]
          frame 0 {
            # ">>> yStepper command>>>"
          }
          frame 1 {
            # ">>> yStepper command>>>"
            n161 = for {
              shift-right: [w303] -> w297
              shift-left: w300 -> [w302]
              tunnel: string[] ["INIT", "RESET ARM", "RESET FLAGS", "RESET YAW", "NAVX CALIBRATE"] -> [w301] mode=indexing
              n162 = Enqueue Element(queue=w302, element=w301) -> (queue out=w303:refnum<queue>)  [unwired: 2 in, 2 out]
            }
            n163 = Bundle By Name(cluster=w295, "yStepper desired"=u8 0) -> (w294:T10)
            n164 = Bundle By Name(cluster=w292, "ySpeed"=0.0, "xSpeed"=0.0, "wSpeed"=0.0) -> (w291:T8)
          }
          frame 3 {
            # ">>> Motor control cluster >>>"
            # ">>> yStepper command>>>"
            n165 = Flush Queue(queue=w309, error in (no error)=w308) -> ()  [unwired: 3 out]
            n166 = for {
              shift-right: [w315] -> w310
              shift-left: w311 -> [w314]
              tunnel: string[] ["STOP", "RESET ENCODERS", "RESET YAW", "RESET ARM", "RESET FLAGS", "DISPOSE BUFFERS", "CAM CLOSE", ""] -> [w313] mode=indexing
              n167 = Enqueue Element(queue=w314, element=w313) -> (queue out=w315:refnum<queue>)  [unwired: 2 in, 2 out]
            }
          }
          frame 4, Default {
            (unwired) TRUE ("Green LED")
            # ">>> yStepper command>>>"
            n168 = Dequeue Element(queue=w326, timeout in ms (-1)=w325, error in (no error)=w321) -> (element=w324:T7)  [unwired: 3 out]
            n169 = case shown="\"Start Task A\"" w324 {
              tunnel: [w328 w335 w342 w349 w356 w363 w370 w372 w380 w387 w393] -> w320
              tunnel: w323 -> [w329 w336 w343 w350 w357 w364 w370 w373 w379 w386 w394]
              tunnel: [State_Type_Definitions."Task 1" ("Enum") State_Type_Definitions."Task 2:Raise Arm" ("Enum") State_Type_Definitions."Task 3" ("Enum") State_Type_Definitions."Task 4_A" ("Enum") State_Type_Definitions."Task 5A: ARM CAM HEIGHT" ("Enum") State_Type_Definitions."Task 6_A" ("Enum") State_Type_Definitions."Idle" ("Enum") State_Type_Definitions."Shutdown" ("Enum") State_Type_Definitions."Task 9A: Raise Arm" ("Enum") State_Type_Definitions."Task A: RAISE ARM TO HEIGHT" ("Enum") State_Type_Definitions."Task 8A: RAISE ARM" ("Enum")] -> w322
              frame "Start Task 1" {
                n170 = for {
                  shift-right: [w333] -> w328
                  shift-left: w329 -> [w332]
                  tunnel: string[] ["RESET ENCODERS", "RESET YAW", "FORWARD", "READ ENCODERS"] -> [w331] mode=indexing
                  n171 = Enqueue Element(queue=w332, element=w331) -> (queue out=w333:refnum<queue>)  [unwired: 2 in, 2 out]
                }
              }
              frame "Start Task 2" {
                n172 = for {
                  shift-right: [w340] -> w335
                  shift-left: w336 -> [w339]
                  tunnel: string[] ["RESET ENCODERS", "RESET YAW", "READ ULTRASONIC", "ARDUINO - ULTRASONIC"] -> [w338] mode=indexing
                  n173 = Enqueue Element(queue=w339, element=w338) -> (queue out=w340:refnum<queue>)  [unwired: 2 in, 2 out]
                }
              }
              frame "Start Task 3" {
                n174 = for {
                  shift-right: [w347] -> w342
                  shift-left: w343 -> [w346]
                  tunnel: string[] ["RESET ENCODERS", "READ ENCODERS", "R-ACW"] -> [w345] mode=indexing
                  n175 = Enqueue Element(queue=w346, element=w345) -> (queue out=w347:refnum<queue>)  [unwired: 2 in, 2 out]
                }
              }
              frame "Start Task 4" {
                n176 = for {
                  shift-right: [w354] -> w349
                  shift-left: w350 -> [w353]
                  tunnel: string[] ["RESET YAW", "RESET ENCODERS", "RESET ARM", "RESET FLAGS", "", ""] -> [w352] mode=indexing
                  n177 = Enqueue Element(queue=w353, element=w352) -> (queue out=w354:refnum<queue>)  [unwired: 2 in, 2 out]
                }
              }
              frame "Start Task 5" {
                n178 = for {
                  shift-right: [w361] -> w356
                  shift-left: w357 -> [w360]
                  tunnel: string[] ["RESET YAW", "RESET ENCODERS", "READ STEPPER VALUES", "Z STEPPER CAM HEIGHT", "", ""] -> [w359] mode=indexing
                  n179 = Enqueue Element(queue=w360, element=w359) -> (queue out=w361:refnum<queue>)  [unwired: 2 in, 2 out]
                }
              }
              frame "Start Task 6" {
                n180 = for {
                  shift-right: [w368] -> w363
                  shift-left: w364 -> [w367]
                  tunnel: string[] ["OPEN LOG CAM ", "", "", "", "", ""] -> [w366] mode=indexing
                  n181 = Enqueue Element(queue=w367, element=w366) -> (queue out=w368:refnum<queue>)  [unwired: 2 in, 2 out]
                }
              }
              frame "None", Default {
              }
              frame "Exit" {
                n182 = for {
                  shift-right: [w377] -> w372
                  shift-left: w373 -> [w376]
                  tunnel: string[] ["STOP", "RESET ENCODERS", "RESET YAW", "EXIT"] -> [w375] mode=indexing
                  n183 = Enqueue Element(queue=w376, element=w375) -> (queue out=w377:refnum<queue>)  [unwired: 2 in, 2 out]
                }
              }
              frame "Start Task 9" {
                n184 = for {
                  shift-right: [w384] -> w380
                  shift-left: w379 -> [w383]
                  tunnel: string[] ["RESET ENCODERS", "READ ENCODERS", "Z STEPPER CAM HEIGHT"] -> [w382] mode=indexing
                  n185 = Enqueue Element(queue=w383, element=w382) -> (queue out=w384:refnum<queue>)  [unwired: 2 in, 2 out]
                }
              }
              frame "Start Task A" {
                n186 = for {
                  shift-right: [w391] -> w387
                  shift-left: w386 -> [w390]
                  tunnel: string[] ["RESET ENCODERS", "READ ENCODERS", "RESET YAW", "Z STEPPER BOX HEIGHT"] -> [w389] mode=indexing
                  n187 = Enqueue Element(queue=w390, element=w389) -> (queue out=w391:refnum<queue>)  [unwired: 2 in, 2 out]
                }
              }
              frame "Start Task 8 - BALL" {
                n188 = for {
                  shift-right: [w398] -> w393
                  shift-left: w394 -> [w397]
                  tunnel: string[] ["RESET YAW", "RESET ENCODERS", "RESET ARM", "RESET FLAGS"] -> [w396] mode=indexing
                  n189 = Enqueue Element(queue=w397, element=w396) -> (queue out=w398:refnum<queue>)  [unwired: 2 in, 2 out]
                }
              }
            }
          }
          frame 5 {
            # ">>> yStepper command>>>"
            n190 = for {
              shift-right: [w408] -> w402
              shift-left: w404 -> [w407]
              tunnel: string[] ["INIT", "RESET ENCODERS", "RESET FLAGS", "CAM CLOSE", "DISPOSE BUFFERS", "EXIT", ""] -> [w406] mode=indexing
              n191 = Enqueue Element(queue=w407, element=w406) -> (queue out=w408:refnum<queue>)  [unwired: 2 in, 2 out]
            }
          }
          frame 6 {
            # ">>> yStepper command>>>"
            # "Use 250"
            n192 = Dequeue Element(queue=w423, timeout in ms (-1)=w422, error in (no error)=w421) -> (element=w420:T7)  [unwired: 3 out]
            n193 = Greater?(x=w414, y=265.0) -> (0:w412:bool)
            n194 = Or(x=w412, y=w415) -> (x .or. y?=w419:bool)
            n195 = case shown="\"None\", Default" w420 {
              tunnel: w419 -> [w426 _]
              tunnel: [w430 State_Type_Definitions."True Stop" ("Enum")] -> w418
              tunnel: w417 -> [w427 w445]
              tunnel: [w425 w444] -> w416
              tunnel: [State_Type_Definitions."Idle" ("Enum") State_Type_Definitions."Shutdown" ("Enum")] -> w411
              frame "None", Default {
                n196 = case shown="True" w426 {
                  tunnel: w427 -> [w433 w439]
                  tunnel: [w432 w437] -> w425
                  frame False {
                    n197 = for {
                      shift-right: [w435] -> w432
                      shift-left: w433 -> [w436]
                      tunnel: string[] ["READ ENCODERS", "READ NAVX", "FORWARD"] ("element") -> [w434] mode=indexing
                      n198 = Enqueue Element(queue=w436, element=w434) -> (queue out=w435:refnum<queue>)  [unwired: 2 in, 2 out]
                    }
                  }
                  frame True {
                    n199 = for {
                      shift-right: [w441] -> w437
                      shift-left: w439 -> [w442]
                      tunnel: string[] ["RESET YAW", "RESET ENCODERS", "STOP", ""] -> [w440] mode=indexing
                      n200 = Enqueue Element(queue=w442, element=w440) -> (queue out=w441:refnum<queue>)  [unwired: 2 in, 2 out]
                    }
                  }
                }
                n201 = Select(t=State_Type_Definitions."True Stop" ("Enum"), s=w426, f=State_Type_Definitions."Task 1" ("Enum")) -> (s? t:f=w430:u16)
              }
              frame "Exit" {
                n202 = for {
                  shift-right: [w449] -> w444
                  shift-left: w445 -> [w450]
                  tunnel: string[] ["STOP", "RESET ENCODERS", "RESET YAW", ""] -> [w448] mode=indexing
                  n203 = Enqueue Element(queue=w450, element=w448) -> (queue out=w449:refnum<queue>)  [unwired: 2 in, 2 out]
                }
              }
            }
          }
          frame 8 {
            # ">> Stepper height reeached >>"
            # ">>> yStepper command>>>"
            # ">> Manual override >>"
            n204 = Dequeue Element(queue=w455, timeout in ms (-1)=w454, error in (no error)=w453) -> (element=w464:T7)  [unwired: 3 out]
            n205 = Equal?(x=w457, y=u8 60) -> (x = y?=w462:bool)
            n206 = case shown="\"None\", Default" w464 {
              tunnel: [w475 State_Type_Definitions."True Stop" ("Enum")] -> w459
              tunnel: [w473 w490] -> w452
              tunnel: w461 -> [w472 _]
              tunnel: w460 -> [w466 _]
              tunnel: [State_Type_Definitions."Idle" ("Enum") State_Type_Definitions."Shutdown" ("Enum")] -> w458
              tunnel: w462 -> [w465 _]
              frame "None", Default {
                # ">> WIill proceed to part ii if not manual override >>"
                # ">>If ENABLE or Trigger is set to true>>"
                n207 = Or(x=w465, y=w466) -> (x .or. y?=w467:bool)
                n208 = case shown="True" w465 {
                  tunnel: [w478 w484] -> w473
                  tunnel: w472 -> [w477 w483]
                  frame False {
                    n209 = for {
                      shift-right: [w480] -> w478
                      shift-left: w477 -> [w481]
                      tunnel: string[] ["Z STEPPER CAM HEIGHT", "READ STEPPER VALUES"] ("element") -> [w479] mode=indexing
                      n210 = Enqueue Element(queue=w481, element=w479) -> (queue out=w480:refnum<queue>)  [unwired: 2 in, 2 out]
                    }
                  }
                  frame True {
                    n211 = for {
                      shift-right: [w486] -> w484
                      shift-left: w483 -> [w487]
                      tunnel: string[] ["ARDUINO - ULTRASONIC", "READ ULTRASONIC", "", "", "", ""] -> [w485] mode=indexing
                      n212 = Enqueue Element(queue=w487, element=w485) -> (queue out=w486:refnum<queue>)  [unwired: 2 in, 2 out]
                    }
                  }
                }
                n213 = Select(t=State_Type_Definitions."True Stop" ("Enum"), s=w466, f=State_Type_Definitions."Task 2:Sensor Mode" ("Enum")) -> (s? t:f=w469:T6)
                n214 = Select(t=w469, s=w467, f=State_Type_Definitions."Task 2:Raise Arm" ("Enum")) -> (s? t:f=w475:T6)
              }
              frame "Exit" {
                n215 = for {
                  shift-right: [w493] -> w490
                  shift-left: _ -> [w494]
                  tunnel: string[] ["STOP", "RESET ENCODERS", "RESET YAW", ""] -> [w492] mode=indexing
                  n216 = Enqueue Element(queue=w494, element=w492) -> (queue out=w493:refnum<queue>)  [unwired: 2 in, 2 out]
                }
              }
            }
          }
          frame 9 {
            w510 = u8 20 ("y")
            # ">>> yStepper command>>>"
            # ">>Object detected>>"
            n217 = Dequeue Element(queue=w502, timeout in ms (-1)=w501, error in (no error)=w500) -> (element=w511:T7)  [unwired: 3 out]
            n218 = Less?(x=w498, y=w510) -> (x < y?=w509:bool)
            n219 = Less?(x=w497, y=w510) -> (x < y?=w508:bool)
            n220 = Or(x=w509, y=w508) -> (x .or. y?=w507:bool)
            "Obstacle detected" <- w507
            n221 = case shown="\"None\", Default" w511 {
              tunnel: w507 -> [w514 _]
              tunnel: [w521 State_Type_Definitions."True Stop" ("Enum")] -> w506
              tunnel: w499 -> [w513 _]
              tunnel: w503 -> [w520 w537]
              tunnel: [w519 w538] -> w505
              tunnel: [State_Type_Definitions."Idle" ("Enum") State_Type_Definitions."Shutdown" ("Enum")] -> w504
              frame "None", Default {
                n222 = case shown="True" w514 {
                  tunnel: w520 -> [w524 w531]
                  tunnel: [w525 w530] -> w519
                  frame False {
                    n223 = for {
                      tunnel: string[] ["READ ULTRASONIC", "STOP"] ("element") -> [w526] mode=indexing
                      shift-right: [w528] -> w525
                      shift-left: w524 -> [w527]
                      n224 = Enqueue Element(queue=w527, element=w526) -> (queue out=w528:refnum<queue>)  [unwired: 2 in, 2 out]
                    }
                  }
                  frame True {
                    n225 = for {
                      shift-right: [w533] -> w530
                      shift-left: w531 -> [w534]
                      tunnel: string[] ["RESET ENCODERS", "READ NAVX", "READ ENCODERS"] -> [w532] mode=indexing
                      n226 = Enqueue Element(queue=w534, element=w532) -> (queue out=w533:refnum<queue>)  [unwired: 2 in, 2 out]
                    }
                  }
                }
                n227 = Or(x=w514, y=w513) -> (x .or. y?=w512:bool)
                n228 = Select(t=State_Type_Definitions."True Stop" ("Enum"), s=w513, f=State_Type_Definitions."Task 2:Reverse Mode" ("Enum")) -> (s? t:f=w515:T6)
                n229 = Select(t=w515, s=w512, f=State_Type_Definitions."Task 2:Sensor Mode" ("Enum")) -> (s? t:f=w521:T6)
              }
              frame "Exit" {
                n230 = for {
                  shift-right: [w541] -> w538
                  shift-left: w537 -> [w542]
                  tunnel: string[] ["STOP", "RESET ENCODERS", "RESET YAW", "ARDUINO MODE 0"] -> [w540] mode=indexing
                  n231 = Enqueue Element(queue=w542, element=w540) -> (queue out=w541:refnum<queue>)  [unwired: 2 in, 2 out]
                }
              }
            }
          }
          frame 10 {
            # ">>> yStepper command>>>"
            n232 = Dequeue Element(queue=w552, timeout in ms (-1)=w553, error in (no error)=w554) -> (element=w556:T7)  [unwired: 3 out]
            n233 = Less?(x=w546, y=-50.0) -> (x < y?=w544:bool)
            n234 = case shown="\"None\", Default" w556 {
              tunnel: [w566 State_Type_Definitions."True Stop" ("Enum")] -> w548
              tunnel: w555 -> [w559 _]
              tunnel: w551 -> [w565 w582]
              tunnel: [w564 w583] -> w547
              tunnel: [State_Type_Definitions."Idle" ("Enum") State_Type_Definitions."Shutdown" ("Enum")] -> w549
              tunnel: w544 -> [w557 _]
              frame "None", Default {
                n235 = case shown="False" w557 {
                  tunnel: w565 -> [w569 w576]
                  tunnel: [w570 w575] -> w564
                  frame False {
                    n236 = for {
                      tunnel: string[] ["READ ENCODERS", "REVERSE", "READ NAVX"] ("element") -> [w571] mode=indexing
                      shift-right: [w573] -> w570
                      shift-left: w569 -> [w572]
                      n237 = Enqueue Element(queue=w572, element=w571) -> (queue out=w573:refnum<queue>)  [unwired: 2 in, 2 out]
                    }
                  }
                  frame True {
                    n238 = for {
                      shift-right: [w578] -> w575
                      shift-left: w576 -> [w579]
                      tunnel: string[] ["STOP", "ARDUINO - ULTRASONIC", "READ ULTRASONIC", "RESET ENCODERS"] -> [w577] mode=indexing
                      n239 = Enqueue Element(queue=w579, element=w577) -> (queue out=w578:refnum<queue>)  [unwired: 2 in, 2 out]
                    }
                  }
                }
                n240 = Or(x=w557, y=w559) -> (x .or. y?=w558:bool)
                n241 = Select(t=State_Type_Definitions."True Stop" ("Enum"), s=w559, f=State_Type_Definitions."Task 2:Sensor Mode" ("Enum")) -> (s? t:f=w560:T6)
                n242 = Select(t=w560, s=w558, f=State_Type_Definitions."Task 2:Reverse Mode" ("Enum")) -> (s? t:f=w566:T6)
              }
              frame "Exit" {
                n243 = for {
                  shift-right: [w586] -> w583
                  shift-left: w582 -> [w587]
                  tunnel: string[] ["STOP", "RESET ENCODERS", "RESET YAW", "ARDUINO MODE 0"] -> [w585] mode=indexing
                  n244 = Enqueue Element(queue=w587, element=w585) -> (queue out=w586:refnum<queue>)  [unwired: 2 in, 2 out]
                }
              }
            }
          }
          frame 11 {
            # ">>> yStepper command>>>"
            n245 = Dequeue Element(queue=w602, timeout in ms (-1)=w601, error in (no error)=w600) -> (element=w591:T7)  [unwired: 3 out]
            n246 = Greater?(x=w599, y=160.0) -> (0:w596:bool)
            n247 = Or(x=w596, y=w597) -> (x .or. y?=w592:bool)
            n248 = case shown="\"None\", Default" w591 {
              tunnel: w592 -> [w605 _]
              tunnel: [w609 State_Type_Definitions."True Stop" ("Enum")] -> w593
              tunnel: w595 -> [w606 w625]
              tunnel: [w604 w624] -> w594
              tunnel: [State_Type_Definitions."Idle" ("Enum") State_Type_Definitions."Shutdown" ("Enum")] -> w590
              frame "None", Default {
                n249 = case shown="False" w605 {
                  tunnel: w606 -> [w612 w618]
                  tunnel: [w611 w616] -> w604
                  frame False {
                    n250 = for {
                      shift-right: [w614] -> w611
                      shift-left: w612 -> [w615]
                      tunnel: string[] ["READ ENCODERS", "R-CW"] ("element") -> [w613] mode=indexing
                      n251 = Enqueue Element(queue=w615, element=w613) -> (queue out=w614:refnum<queue>)  [unwired: 2 in, 2 out]
                    }
                  }
                  frame True {
                    n252 = for {
                      shift-right: [w620] -> w616
                      shift-left: w618 -> [w621]
                      tunnel: string[] ["RESET YAW", "RESET ENCODERS", "STOP", "ARDUINO MODE 0"] -> [w619] mode=indexing
                      n253 = Enqueue Element(queue=w621, element=w619) -> (queue out=w620:refnum<queue>)  [unwired: 2 in, 2 out]
                    }
                  }
                }
                n254 = Select(t=State_Type_Definitions."True Stop" ("Enum"), s=w605, f=State_Type_Definitions."Task 3" ("Enum")) -> (s? t:f=w609:T6)
              }
              frame "Exit" {
                n255 = for {
                  shift-right: [w628] -> w624
                  shift-left: w625 -> [w629]
                  tunnel: string[] ["STOP", "RESET ENCODERS", "RESET YAW", ""] -> [w627] mode=indexing
                  n256 = Enqueue Element(queue=w629, element=w627) -> (queue out=w628:refnum<queue>)  [unwired: 2 in, 2 out]
                }
              }
            }
          }
          frame 12 {
            # ">> Stepper height reeached >>"
            # ">>> yStepper command>>>"
            # ">> Manual override >>"
            n257 = Dequeue Element(queue=w642, timeout in ms (-1)=w641, error in (no error)=w640) -> (element=w639:T7)  [unwired: 3 out]
            n258 = Equal?(x=w633, y=u8 60) -> (x = y?=w631:bool)
            n259 = case shown="\"Exit\"" w639 {
              tunnel: [w654 State_Type_Definitions."True Stop" ("Enum")] -> w638
              tunnel: [w652 w670] -> w637
              tunnel: w643 -> [w651 w667]
              tunnel: w636 -> [w645 _]
              tunnel: [State_Type_Definitions."Idle" ("Enum") State_Type_Definitions."Shutdown" ("Enum")] -> w635
              tunnel: w631 -> [w644 _]
              frame "None", Default {
                # ">> WIill proceed to part ii if not manual override >>"
                # ">>If ENABLE or Trigger is set to true>>"
                n260 = Or(x=w644, y=w645) -> (x .or. y?=w646:bool)
                n261 = case shown="False" w644 {
                  tunnel: [w657 w663] -> w652
                  tunnel: w651 -> [w656 w662]
                  frame False {
                    n262 = for {
                      shift-right: [w659] -> w657
                      shift-left: w656 -> [w660]
                      tunnel: string[] ["Z STEPPER CAM HEIGHT", "READ STEPPER VALUES"] ("element") -> [w658] mode=indexing
                      n263 = Enqueue Element(queue=w660, element=w658) -> (queue out=w659:refnum<queue>)  [unwired: 2 in, 2 out]
                    }
                  }
                  frame True {
                    n264 = for {
                      shift-right: [w665] -> w663
                      shift-left: w662 -> [w666]
                      tunnel: string[] ["ARDUINO - ULTRASONIC", "READ ULTRASONIC", "FORWARD", "", "", ""] -> [w664] mode=indexing
                      n265 = Enqueue Element(queue=w666, element=w664) -> (queue out=w665:refnum<queue>)  [unwired: 2 in, 2 out]
                    }
                  }
                }
                n266 = Select(t=State_Type_Definitions."True Stop" ("Enum"), s=w645, f=State_Type_Definitions."Task 4_B" ("Enum")) -> (s? t:f=w648:T6)
                n267 = Select(t=w648, s=w646, f=State_Type_Definitions."Task 4_A" ("Enum")) -> (s? t:f=w654:T6)
              }
              frame "Exit" {
                n268 = for {
                  shift-right: [w673] -> w670
                  shift-left: w667 -> [w674]
                  tunnel: string[] ["STOP", "RESET ENCODERS", "RESET YAW", ""] -> [w672] mode=indexing
                  n269 = Enqueue Element(queue=w674, element=w672) -> (queue out=w673:refnum<queue>)  [unwired: 2 in, 2 out]
                }
              }
            }
          }
          frame 13 {
            w679 = u8 20
            # ">> Path blocked >>"
            # ">>> yStepper command>>>"
            # ">> Manual override >>"
            n270 = Dequeue Element(queue=w688, timeout in ms (-1)=w687, error in (no error)=w686) -> (element=w685:T7)  [unwired: 3 out]
            n271 = Less?(x=w681, y=w679) -> (x < y?=w676:bool)
            n272 = Less?(x=w680, y=w679) -> (x < y?=w677:bool)
            n273 = And(x=w677, y=w676) -> (x .and. y?=w678:bool)
            n274 = case shown="\"None\", Default" w685 {
              tunnel: [w702 State_Type_Definitions."True Stop" ("Enum")] -> w690
              tunnel: [w700 w717] -> w691
              tunnel: w684 -> [w699 _]
              tunnel: w689 -> [w693 _]
              tunnel: [State_Type_Definitions."Idle" ("Enum") State_Type_Definitions."Shutdown" ("Enum")] -> w683
              tunnel: w678 -> [w692 _]
              frame "None", Default {
                # ">> Manual override forces program to true stop >>"
                # ">>If ENABLE or Trigger is set to true>>"
                n275 = Or(x=w692, y=w693) -> (x .or. y?=w698:bool)
                n276 = case shown="True" w692 {
                  tunnel: [w705 w710] -> w700
                  tunnel: w699 -> [w704 w709]
                  frame False {
                    n277 = for {
                      shift-right: [w707] -> w705
                      shift-left: w704 -> [w708]
                      tunnel: string[] ["FORWARD", "READ ULTRASONIC", "READ NAVX"] ("element") -> [w706] mode=indexing
                      n278 = Enqueue Element(queue=w708, element=w706) -> (queue out=w707:refnum<queue>)  [unwired: 2 in, 2 out]
                    }
                  }
                  frame True {
                    n279 = for {
                      shift-right: [w713] -> w710
                      shift-left: w709 -> [w714]
                      tunnel: string[] ["STOP", "RESET YAW", "RESET ENCODERS", "RESET FLAGS"] -> [w712] mode=indexing
                      n280 = Enqueue Element(queue=w714, element=w712) -> (queue out=w713:refnum<queue>)  [unwired: 2 in, 2 out]
                    }
                  }
                }
                n281 = Select(t=State_Type_Definitions."True Stop" ("Enum"), s=w693, f=State_Type_Definitions."Task 4_C" ("Enum")) -> (s? t:f=w695:T6)
                n282 = Select(t=w695, s=w698, f=State_Type_Definitions."Task 4_B" ("Enum")) -> (s? t:f=w702:T6)
              }
              frame "Exit" {
                n283 = for {
                  shift-right: [w720] -> w717
                  shift-left: _ -> [w721]
                  tunnel: string[] ["STOP", "RESET ENCODERS", "RESET YAW", ""] -> [w719] mode=indexing
                  n284 = Enqueue Element(queue=w721, element=w719) -> (queue out=w720:refnum<queue>)  [unwired: 2 in, 2 out]
                }
              }
            }
          }
          frame 14 {
            w732 = u8 20
            # ">> xDistance travelled>>"
            # ">> Path NOT blocked >>"
            # ">>> yStepper command>>>"
            # ">> Manual override >>"
            n285 = Dequeue Element(queue=w742, timeout in ms (-1)=w735, error in (no error)=w734) -> (element=w736:T7)  [unwired: 3 out]
            n286 = Greater?(x=w724, y=w732) -> (0:w730:bool)
            n287 = Greater?(x=w729, y=80.0) -> (0:w727:bool)
            n288 = Greater?(x=w723, y=w732) -> (0:w731:bool)
            n289 = And(x=w731, y=w730) -> (x .and. y?=w726:bool)
            n290 = And(x=w727, y=w726) -> (x .and. y?=w725:bool)
            n291 = case shown="\"Exit\"" w736 {
              tunnel: [w753 State_Type_Definitions."True Stop" ("Enum")] -> w739
              tunnel: [w751 w769] -> w738
              tunnel: w741 -> [w750 w766]
              tunnel: w740 -> [w744 _]
              tunnel: [State_Type_Definitions."Idle" ("t") State_Type_Definitions."Shutdown" ("Enum")] -> w737
              tunnel: w725 -> [w743 _]
              frame "None", Default {
                # ">> Manual override forces program to true stop >>"
                # ">>If ENABLE or Trigger is set to true>>"
                n292 = Or(x=w743, y=w744) -> (x .or. y?=w749:bool)
                n293 = case shown="False" w743 {
                  tunnel: [w756 w761] -> w751
                  tunnel: w750 -> [w754 w760]
                  frame False {
                    n294 = for {
                      shift-right: [w758] -> w756
                      shift-left: w754 -> [w759]
                      tunnel: string[] ["RIGHT", "READ NAVX", "READ ENCODERS", "READ ULTRASONIC"] ("element") -> [w757] mode=indexing
                      n295 = Enqueue Element(queue=w759, element=w757) -> (queue out=w758:refnum<queue>)  [unwired: 2 in, 2 out]
                    }
                  }
                  frame True {
                    n296 = for {
                      shift-right: [w764] -> w761
                      shift-left: w760 -> [w765]
                      tunnel: string[] ["STOP", "RESET YAW", "RESET ENCODERS", "ARDUINO - ULTRASONIC"] -> [w763] mode=indexing
                      n297 = Enqueue Element(queue=w765, element=w763) -> (queue out=w764:refnum<queue>)  [unwired: 2 in, 2 out]
                    }
                  }
                }
                n298 = Select(t=State_Type_Definitions."True Stop" ("Enum"), s=w744, f=State_Type_Definitions."Task 4_D" ("Enum")) -> (s? t:f=w745:T6)
                n299 = Select(t=w745, s=w749, f=State_Type_Definitions."Task 4_C" ("Enum")) -> (s? t:f=w753:T6)
              }
              frame "Exit" {
                n300 = for {
                  shift-right: [w772] -> w769
                  shift-left: w766 -> [w773]
                  tunnel: string[] ["STOP", "RESET ENCODERS", "RESET YAW", ""] -> [w771] mode=indexing
                  n301 = Enqueue Element(queue=w773, element=w771) -> (queue out=w772:refnum<queue>)  [unwired: 2 in, 2 out]
                }
              }
            }
          }
          frame 15 {
            w793 = u8 20
            # ">> yDistance travelled>>"
            # ">> Path blocked >>"
            # ">>> yStepper command>>>"
            # ">> Manual override >>"
            n302 = Dequeue Element(queue=w784, timeout in ms (-1)=w783, error in (no error)=w782) -> (element=w794:T7)  [unwired: 3 out]
            n303 = Less?(x=w777, y=w793) -> (x < y?=w791:bool)
            n304 = Greater?(x=w781, y=200.0) -> (0:w789:bool)
            n305 = Less?(x=w776, y=w793) -> (x < y?=w792:bool)
            n306 = And(x=w792, y=w791) -> (x .and. y?=w788:bool)
            n307 = Or(x=w789, y=w788) -> (x .or. y?=w787:bool)
            n308 = case shown="\"None\", Default" w794 {
              tunnel: [w805 State_Type_Definitions."True Stop" ("Enum")] -> w780
              tunnel: [w803 w821] -> w778
              tunnel: w785 -> [w802 w818]
              tunnel: w786 -> [w796 _]
              tunnel: [State_Type_Definitions."Idle" ("t") State_Type_Definitions."Shutdown" ("Enum")] -> w779
              tunnel: w787 -> [w795 _]
              frame "None", Default {
                # ">> Manual override forces program to true stop >>"
                # ">>If ENABLE or Trigger is set to true>>"
                n309 = Or(x=w795, y=w796) -> (x .or. y?=w801:bool)
                n310 = case shown="True" w795 {
                  tunnel: [w808 w813] -> w803
                  tunnel: w802 -> [w806 w812]
                  frame False {
                    n311 = for {
                      shift-right: [w810] -> w808
                      shift-left: w806 -> [w811]
                      tunnel: string[] ["FORWARD", "READ NAVX", "READ ENCODERS", "READ ULTRASONIC"] ("element") -> [w809] mode=indexing
                      n312 = Enqueue Element(queue=w811, element=w809) -> (queue out=w810:refnum<queue>)  [unwired: 2 in, 2 out]
                    }
                  }
                  frame True {
                    n313 = for {
                      shift-right: [w816] -> w813
                      shift-left: w812 -> [w817]
                      tunnel: string[] ["STOP", "RESET YAW", "RESET ENCODERS", "RESET FLAGS"] -> [w815] mode=indexing
                      n314 = Enqueue Element(queue=w817, element=w815) -> (queue out=w816:refnum<queue>)  [unwired: 2 in, 2 out]
                    }
                  }
                }
                n315 = Select(t=State_Type_Definitions."True Stop" ("Enum"), s=w796, f=State_Type_Definitions."True Stop" ("Enum")) -> (s? t:f=w797:T6)
                n316 = Select(t=w797, s=w801, f=State_Type_Definitions."Task 4_D" ("Enum")) -> (s? t:f=w805:T6)
              }
              frame "Exit" {
                n317 = for {
                  shift-right: [w824] -> w821
                  shift-left: w818 -> [w825]
                  tunnel: string[] ["STOP", "RESET ENCODERS", "RESET YAW", ""] -> [w823] mode=indexing
                  n318 = Enqueue Element(queue=w825, element=w823) -> (queue out=w824:refnum<queue>)  [unwired: 2 in, 2 out]
                }
              }
            }
          }
          frame 15 {
            # ">>> yStepper command>>>"
            # ">> Manual override >>"
            n319 = Dequeue Element(queue=w835, timeout in ms (-1)=w834, error in (no error)=w836) -> (element=w833:T7)  [unwired: 3 out]
            n320 = Equal?(x=w832, y=u8 60) -> (x = y?=w830:bool)
            n321 = case shown="\"None\", Default" w833 {
              tunnel: [w846 State_Type_Definitions."True Stop" ("Enum")] -> w837
              tunnel: [w849 w866] -> w838
              tunnel: [State_Type_Definitions."Idle" ("Enum") State_Type_Definitions."Shutdown" ("Enum")] -> w839
              tunnel: w830 -> [w845 _]
              tunnel: w829 -> [w844 _]
              tunnel: w828 -> [w840 w863]
              frame "None", Default {
                # "Stays in Task 5_A until stepper reaches desired \nheight"
                # "T: Go back to idle, F: Continue with task\""
                # ">> Manual override >>"
                n322 = case shown="True" w845 {
                  tunnel: [w853 w859] -> w849
                  tunnel: w840 -> [w851 w857]
                  frame False {
                    n323 = for {
                      tunnel: string[] ["Z STEPPER CAM HEIGHT", "READ STEPPER VALUES"] ("element") -> [w854] mode=indexing
                      shift-right: [w856] -> w853
                      shift-left: w851 -> [w855]
                      n324 = Enqueue Element(queue=w855, element=w854) -> (queue out=w856:refnum<queue>)  [unwired: 2 in, 2 out]
                    }
                  }
                  frame True {
                    n325 = for {
                      shift-right: [w861] -> w859
                      shift-left: w857 -> [w862]
                      tunnel: string[] ["ARDUINO - ULTRASONIC", "READ ULTRASONIC", ""] -> [w860] mode=indexing
                      n326 = Enqueue Element(queue=w862, element=w860) -> (queue out=w861:refnum<queue>)  [unwired: 2 in, 2 out]
                    }
                  }
                }
                n327 = Or(x=w845, y=w844) -> (x .or. y?=w847:bool)
                n328 = Select(t=State_Type_Definitions."True Stop" ("Enum"), s=w844, f=State_Type_Definitions."Task 5B: MOVE TO BOX" ("Enum")) -> (s? t:f=w841:u16)
                n329 = Select(t=w841, s=w847, f=State_Type_Definitions."Task 5A: ARM CAM HEIGHT" ("Enum")) -> (s? t:f=w846:u16)
              }
              frame "Exit" {
                n330 = for {
                  shift-right: [w869] -> w866
                  shift-left: w863 -> [w870]
                  tunnel: string[] ["STOP", "RESET ENCODERS", "RESET YAW", "ARDUINO MODE 0"] -> [w868] mode=indexing
                  n331 = Enqueue Element(queue=w870, element=w868) -> (queue out=w869:refnum<queue>)  [unwired: 2 in, 2 out]
                }
              }
            }
          }
          frame 16 {
            w877 = u8 20 ("y")
            # ">>> yStepper command>>>"
            n332 = Less?(x=w874, y=w877) -> (x < y?=w875:bool)
            n333 = Dequeue Element(queue=w881, timeout in ms (-1)=w880, error in (no error)=w882) -> (element=w879:T7)  [unwired: 3 out]
            n334 = Less?(x=w873, y=w877) -> (x < y?=w876:bool)
            n335 = And(x=w876, y=w875) -> (x .and. y?=w872:bool)
            n336 = case shown="\"None\", Default" w879 {
              tunnel: [w894 State_Type_Definitions."True Stop" ("Enum")] -> w884
              tunnel: [w897 w914] -> w883
              tunnel: [State_Type_Definitions."Idle" ("Enum") State_Type_Definitions."Shutdown" ("Enum")] -> w885
              tunnel: w887 -> [w893 _]
              tunnel: w886 -> [w889 w911]
              tunnel: w872 -> [w888 _]
              frame "None", Default {
                # "Stays in Task 5_B to capture image over 5 seconds"
                # "T: Go back to idle, F: Continue with task\""
                # ">> Manual override >>"
                n337 = case shown="True" w888 {
                  tunnel: [w901 w907] -> w897
                  tunnel: w889 -> [w899 w905]
                  frame False {
                    n338 = for {
                      tunnel: string[] ["FORWARD", "READ ULTRASONIC", "READ NAVX"] ("element") -> [w902] mode=indexing
                      shift-right: [w904] -> w901
                      shift-left: w899 -> [w903]
                      n339 = Enqueue Element(queue=w903, element=w902) -> (queue out=w904:refnum<queue>)  [unwired: 2 in, 2 out]
                    }
                  }
                  frame True {
                    n340 = for {
                      shift-right: [w909] -> w907
                      shift-left: w905 -> [w910]
                      tunnel: string[] ["STOP", "RESET ENCODERS", "OPEN LOG CAM", "SET TIMER 5"] -> [w908] mode=indexing
                      n341 = Enqueue Element(queue=w910, element=w908) -> (queue out=w909:refnum<queue>)  [unwired: 2 in, 2 out]
                    }
                  }
                }
                n342 = Or(x=w888, y=w893) -> (x .or. y?=w895:bool)
                n343 = Select(t=State_Type_Definitions."True Stop" ("Enum"), s=w893, f=State_Type_Definitions."Task 5C: CAM BURST" ("Enum")) -> (s? t:f=w890:u16)
                n344 = Select(t=w890, s=w895, f=State_Type_Definitions."Task 5B: MOVE TO BOX" ("Enum")) -> (s? t:f=w894:u16)
              }
              frame "Exit" {
                n345 = for {
                  shift-right: [w917] -> w914
                  shift-left: w911 -> [w918]
                  tunnel: string[] ["STOP", "RESET ENCODERS", "RESET YAW", "ARDUINO MODE 0"] -> [w916] mode=indexing
                  n346 = Enqueue Element(queue=w918, element=w916) -> (queue out=w917:refnum<queue>)  [unwired: 2 in, 2 out]
                }
              }
            }
          }
          frame 17 {
            # ">>> Motor control cluster >>>"
            # ">>> yStepper command>>>"
            # ">> Manual override >>"
            n347 = Dequeue Element(queue=w928, timeout in ms (-1)=w927, error in (no error)=w926) -> (element=w925:T7)  [unwired: 3 out]
            n348 = case shown="\"None\", Default" w925 {
              tunnel: [w937 State_Type_Definitions."True Stop" ("Enum")] -> w930
              tunnel: [w940 w957] -> w923
              tunnel: [State_Type_Definitions."Idle" ("Enum") State_Type_Definitions."Shutdown" ("Enum")] -> w922
              tunnel: w924 -> [w931 _]
              tunnel: w929 -> [w936 w954]
              tunnel: w920 -> [w935 _]
              frame "None", Default {
                # ">> Is time up? >>"
                # "Determines if object is in range to pick up"
                # ">> Manual override >>"
                n349 = case shown="False" w935 {
                  tunnel: [w944 w950] -> w940
                  tunnel: w936 -> [w942 w948]
                  frame False {
                    n350 = for {
                      tunnel: string[] ["CAM ACQ", "START TIMER"] ("element") -> [w945] mode=indexing
                      shift-right: [w947] -> w944
                      shift-left: w942 -> [w946]
                      n351 = Enqueue Element(queue=w946, element=w945) -> (queue out=w947:refnum<queue>)  [unwired: 2 in, 2 out]
                    }
                  }
                  frame True {
                    n352 = for {
                      shift-right: [w952] -> w950
                      shift-left: w948 -> [w953]
                      tunnel: string[] ["CAM CLOSE", "PROCESS IMAGE", "SET TIMER 5"] -> [w951] mode=indexing
                      n353 = Enqueue Element(queue=w953, element=w951) -> (queue out=w952:refnum<queue>)  [unwired: 2 in, 2 out]
                    }
                  }
                }
                n354 = Or(x=w935, y=w931) -> (x .or. y?=w938:bool)
                n355 = Select(t=State_Type_Definitions."True Stop" ("Enum"), s=w931, f=State_Type_Definitions."Task 5D: PROCESS IMAGE" ("Enum")) -> (s? t:f=w933:u16)
                n356 = Select(t=w933, s=w938, f=State_Type_Definitions."Task 5C: CAM BURST" ("Enum")) -> (s? t:f=w937:u16)
              }
              frame "Exit" {
                n357 = for {
                  shift-right: [w960] -> w957
                  shift-left: w954 -> [w961]
                  tunnel: string[] ["STOP", "RESET ENCODERS", "RESET YAW", "ARDUINO MODE 0"] -> [w959] mode=indexing
                  n358 = Enqueue Element(queue=w961, element=w959) -> (queue out=w960:refnum<queue>)  [unwired: 2 in, 2 out]
                }
              }
            }
          }
          frame 18 {
            # ">>> yStepper command>>>"
            n359 = Dequeue Element(queue=w968, timeout in ms (-1)=w967, error in (no error)=w966) -> (element=w965:T7)  [unwired: 3 out]
            n360 = case shown="\"None\", Default" w965 {
              tunnel: [w980 State_Type_Definitions."True Stop" ("Enum")] -> w972
              tunnel: [w983 w1000] -> w971
              tunnel: [State_Type_Definitions."Idle" ("Enum") State_Type_Definitions."Shutdown" ("Enum")] -> w973
              tunnel: w969 -> [w979 _]
              tunnel: w970 -> [w975 w997]
              tunnel: w963 -> [w974 _]
              frame "None", Default {
                # ">> T: Breaks out of state loop; F: Stays in loop>>"
                # ">> Manual override >>"
                # ">> Checks if time is up>>"
                # "Stays in Task 5D until the object is detected"
                # "T: Go back to idle, F: Continue with task\""
                # ">> Manual override >>"
                n361 = case shown="True" w974 {
                  tunnel: [w987 w993] -> w983
                  tunnel: w975 -> [w985 w991]
                  frame False {
                    n362 = for {
                      tunnel: string[] ["START TIMER", "PROCESS IMAGE", ""] ("element") -> [w988] mode=indexing
                      shift-right: [w990] -> w987
                      shift-left: w985 -> [w989]
                      n363 = Enqueue Element(queue=w989, element=w988) -> (queue out=w990:refnum<queue>)  [unwired: 2 in, 2 out]
                    }
                  }
                  frame True {
                    n364 = for {
                      shift-right: [w995] -> w993
                      shift-left: w991 -> [w996]
                      tunnel: string[] ["CAM CLOSE", "", ""] -> [w994] mode=indexing
                      n365 = Enqueue Element(queue=w996, element=w994) -> (queue out=w995:refnum<queue>)  [unwired: 2 in, 2 out]
                    }
                  }
                }
                n366 = Or(x=w974, y=w979) -> (x .or. y?=w981:bool)
                n367 = Select(t=State_Type_Definitions."True Stop" ("Enum"), s=w979, f=State_Type_Definitions."Task 5E: POSITION ARM" ("Enum")) -> (s? t:f=w976:T6)
                n368 = Select(t=w976, s=w981, f=State_Type_Definitions."Task 5D: PROCESS IMAGE" ("Enum")) -> (s? t:f=w980:u16)
              }
              frame "Exit" {
                n369 = for {
                  shift-right: [w1003] -> w1000
                  shift-left: w997 -> [w1004]
                  tunnel: string[] ["STOP", "RESET ENCODERS", "RESET YAW", "ARDUINO MODE 0"] -> [w1002] mode=indexing
                  n370 = Enqueue Element(queue=w1004, element=w1002) -> (queue out=w1003:refnum<queue>)  [unwired: 2 in, 2 out]
                }
              }
            }
          }
          frame 20 {
            # ">>> yStepper command>>>"
            n371 = Dequeue Element(queue=w1017, timeout in ms (-1)=w1018, error in (no error)=w1019) -> (element=w1021:T7)  [unwired: 3 out]
            n372 = formula code="if (pos < 100)\ny = 41;\n\nelse if (pos >= 100 && pos <= 140)\ny = 30;\n\nelse if (pos >= 141 && pos <= 170)\ny = 25;\n\nelse if (pos >= 171 &&pos <= 180) \ny = 20;\n\nelse if (pos >= 181&& pos <= 200)\ny = 15;\n\nelse if (pos >= 201 && pos <= 230)\ny = 10;\n\nelse if (pos >= 231 && pos <= 320)\ny = 8;\n\nelse if (pos > 320)\ny = 0;"("pos"=w1009) -> ("y"=w1012:dbl)
            n373 = To Unsigned Byte Integer(number=w1012) -> (unsigned 8bit integer=w1007:u8)
            n374 = Equal?(x=w1008, y=w1007) -> (x = y?=w1006:bool)
            n375 = case shown="\"None\", Default" w1021 {
              tunnel: [w1028 State_Type_Definitions."True Stop" ("Enum")] -> w1015
              tunnel: [w1031 w1048] -> w1013
              tunnel: [State_Type_Definitions."Idle" ("Enum") State_Type_Definitions."Shutdown" ("Enum")] -> w1014
              tunnel: w1020 -> [w1027 _]
              tunnel: w1016 -> [w1023 w1045]
              tunnel: w1006 -> [w1022 _]
              frame "None", Default {
                # ">> T: Breaks out of state loop; F: Stays in loop>>"
                # ">> Manual override >>"
                # ">> Checks if time is up>>"
                # "Stays in Task 5D until the object is detected"
                # "T: Go back to idle, F: Continue with task\""
                # ">> Manual override >>"
                n376 = case shown="False" w1022 {
                  tunnel: [w1035 w1041] -> w1031
                  tunnel: w1023 -> [w1033 w1039]
                  frame False {
                    n377 = for {
                      tunnel: string[] ["READ STEPPER VALUES", "Y STEPPER CONTROL", ""] ("element") -> [w1036] mode=indexing
                      shift-right: [w1038] -> w1035
                      shift-left: w1033 -> [w1037]
                      n378 = Enqueue Element(queue=w1037, element=w1036) -> (queue out=w1038:refnum<queue>)  [unwired: 2 in, 2 out]
                    }
                  }
                  frame True {
                    n379 = for {
                      shift-right: [w1043] -> w1041
                      shift-left: w1039 -> [w1044]
                      tunnel: string[] ["CAM CLOSE", "DISPOSE BUFFERS", ""] -> [w1042] mode=indexing
                      n380 = Enqueue Element(queue=w1044, element=w1042) -> (queue out=w1043:refnum<queue>)  [unwired: 2 in, 2 out]
                    }
                  }
                }
                n381 = Or(x=w1022, y=w1027) -> (x .or. y?=w1029:bool)
                n382 = Select(t=State_Type_Definitions."True Stop" ("Enum"), s=w1027, f=State_Type_Definitions."Task 5F: ARM GRAB HEIGHT" ("Enum")) -> (s? t:f=w1024:T6)
                n383 = Select(t=w1024, s=w1029, f=State_Type_Definitions."Task 5E: POSITION ARM" ("Enum")) -> (s? t:f=w1028:T6)
              }
              frame "Exit" {
                n384 = for {
                  shift-right: [w1051] -> w1048
                  shift-left: w1045 -> [w1052]
                  tunnel: string[] ["STOP", "RESET ENCODERS", "RESET YAW", "ARDUINO MODE 0"] -> [w1050] mode=indexing
                  n385 = Enqueue Element(queue=w1052, element=w1050) -> (queue out=w1051:refnum<queue>)  [unwired: 2 in, 2 out]
                }
              }
            }
            n386 = Bundle By Name(cluster=w1011, "yStepper desired"=w1007) -> (w1010:T10)
          }
          frame 21 {
            # ">>> Motor control cluster >>>"
            # ">>> yStepper command>>>"
            # ">> Manual override >>"
            n387 = Dequeue Element(queue=w1062, timeout in ms (-1)=w1061, error in (no error)=w1063) -> (element=w1060:T7)  [unwired: 3 out]
            n388 = Equal?(x=w1059, y=u8 1) -> (x = y?=w1057:bool)
            n389 = case shown="\"None\", Default" w1060 {
              tunnel: [w1073 State_Type_Definitions."True Stop" ("Enum")] -> w1064
              tunnel: [w1076 w1093] -> w1065
              tunnel: [State_Type_Definitions."Idle" ("Enum") State_Type_Definitions."Shutdown" ("Enum")] -> w1066
              tunnel: w1057 -> [w1072 _]
              tunnel: w1056 -> [w1071 _]
              tunnel: w1055 -> [w1067 w1090]
              frame "None", Default {
                # "Stays in Task 5F until stepper reaches desired \nheight"
                # "T: Go back to idle, F: Continue with task\""
                # ">> Manual override >>"
                n390 = case shown="True" w1072 {
                  tunnel: [w1080 w1086] -> w1076
                  tunnel: w1067 -> [w1078 w1084]
                  frame False {
                    n391 = for {
                      tunnel: string[] ["Z STEPPER GRAB HEIGHT", "READ STEPPER VALUES"] ("element") -> [w1081] mode=indexing
                      shift-right: [w1083] -> w1080
                      shift-left: w1078 -> [w1082]
                      n392 = Enqueue Element(queue=w1082, element=w1081) -> (queue out=w1083:refnum<queue>)  [unwired: 2 in, 2 out]
                    }
                  }
                  frame True {
                    n393 = for {
                      shift-right: [w1088] -> w1086
                      shift-left: w1084 -> [w1089]
                      tunnel: string[] ["SET TIMER 5", "CLOSE CLAW", ""] -> [w1087] mode=indexing
                      n394 = Enqueue Element(queue=w1089, element=w1087) -> (queue out=w1088:refnum<queue>)  [unwired: 2 in, 2 out]
                    }
                  }
                }
                n395 = Or(x=w1072, y=w1071) -> (x .or. y?=w1074:bool)
                n396 = Select(t=State_Type_Definitions."True Stop" ("Enum"), s=w1071, f=State_Type_Definitions."Task 5G: CLOSE CLAW" ("Enum")) -> (s? t:f=w1068:T6)
                n397 = Select(t=w1068, s=w1074, f=State_Type_Definitions."Task 5F: ARM GRAB HEIGHT" ("Enum")) -> (s? t:f=w1073:T6)
              }
              frame "Exit" {
                n398 = for {
                  shift-right: [w1096] -> w1093
                  shift-left: w1090 -> [w1097]
                  tunnel: string[] ["STOP", "RESET ENCODERS", "RESET YAW", "ARDUINO MODE 0"] -> [w1095] mode=indexing
                  n399 = Enqueue Element(queue=w1097, element=w1095) -> (queue out=w1096:refnum<queue>)  [unwired: 2 in, 2 out]
                }
              }
            }
          }
          frame 22 {
            # ">>> yStepper command>>>"
            # ">> Manual override >>"
            n400 = Dequeue Element(queue=w1107, timeout in ms (-1)=w1106, error in (no error)=w1105) -> (element=w1104:T7)  [unwired: 3 out]
            n401 = case shown="\"None\", Default" w1104 {
              tunnel: [w1116 State_Type_Definitions."True Stop" ("Enum")] -> w1109
              tunnel: [w1119 w1136] -> w1102
              tunnel: [State_Type_Definitions."Idle" ("Enum") State_Type_Definitions."Shutdown" ("Enum")] -> w1101
              tunnel: w1103 -> [w1110 _]
              tunnel: w1108 -> [w1115 w1133]
              tunnel: w1099 -> [w1114 _]
              frame "None", Default {
                # ">> Is time up? >>"
                # "Determines if object is in range to pick up"
                # ">> Manual override >>"
                n402 = case shown="True" w1114 {
                  tunnel: [w1123 w1129] -> w1119
                  tunnel: w1115 -> [w1121 w1127]
                  frame False {
                    n403 = for {
                      tunnel: string[] ["CLOSE CLAW", "START TIMER"] ("element") -> [w1124] mode=indexing
                      shift-right: [w1126] -> w1123
                      shift-left: w1121 -> [w1125]
                      n404 = Enqueue Element(queue=w1125, element=w1124) -> (queue out=w1126:refnum<queue>)  [unwired: 2 in, 2 out]
                    }
                  }
                  frame True {
                    n405 = for {
                      shift-right: [w1131] -> w1129
                      shift-left: w1127 -> [w1132]
                      tunnel: string[] ["READ STEPPER VALUES", "", ""] -> [w1130] mode=indexing
                      n406 = Enqueue Element(queue=w1132, element=w1130) -> (queue out=w1131:refnum<queue>)  [unwired: 2 in, 2 out]
                    }
                  }
                }
                n407 = Or(x=w1114, y=w1110) -> (x .or. y?=w1117:bool)
                n408 = Select(t=State_Type_Definitions."True Stop" ("Enum"), s=w1110, f=State_Type_Definitions."Task 5H: RAISE ARM" ("Enum")) -> (s? t:f=w1112:T6)
                n409 = Select(t=w1112, s=w1117, f=State_Type_Definitions."Task 5G: CLOSE CLAW" ("Enum")) -> (s? t:f=w1116:T6)
              }
              frame "Exit" {
                n410 = for {
                  shift-right: [w1139] -> w1136
                  shift-left: w1133 -> [w1140]
                  tunnel: string[] ["STOP", "RESET ENCODERS", "RESET YAW", "ARDUINO MODE 0"] -> [w1138] mode=indexing
                  n411 = Enqueue Element(queue=w1140, element=w1138) -> (queue out=w1139:refnum<queue>)  [unwired: 2 in, 2 out]
                }
              }
            }
          }
          frame 23 {
            # ">>> yStepper command>>>"
            # ">> Manual override >>"
            n412 = Dequeue Element(queue=w1150, timeout in ms (-1)=w1149, error in (no error)=w1151) -> (element=w1148:T7)  [unwired: 3 out]
            n413 = Equal?(x=w1147, y=u8 60) -> (x = y?=w1145:bool)
            n414 = case shown="\"None\", Default" w1148 {
              tunnel: [w1161 State_Type_Definitions."True Stop" ("Enum")] -> w1152
              tunnel: [w1164 w1181] -> w1153
              tunnel: [State_Type_Definitions."Idle" ("Enum") State_Type_Definitions."Shutdown" ("Enum")] -> w1154
              tunnel: w1145 -> [w1160 _]
              tunnel: w1144 -> [w1159 _]
              tunnel: w1143 -> [w1155 w1178]
              frame "None", Default {
                # "Stays in Task 5_A until stepper reaches desired \nheight"
                # "T: Go back to idle, F: Continue with task\""
                # ">> Manual override >>"
                n415 = case shown="False" w1160 {
                  tunnel: [w1168 w1174] -> w1164
                  tunnel: w1155 -> [w1166 w1172]
                  frame False {
                    n416 = for {
                      tunnel: string[] ["Z STEPPER CAM HEIGHT", "READ STEPPER VALUES"] ("element") -> [w1169] mode=indexing
                      shift-right: [w1171] -> w1168
                      shift-left: w1166 -> [w1170]
                      n417 = Enqueue Element(queue=w1170, element=w1169) -> (queue out=w1171:refnum<queue>)  [unwired: 2 in, 2 out]
                    }
                  }
                  frame True {
                    n418 = for {
                      shift-right: [w1176] -> w1174
                      shift-left: w1172 -> [w1177]
                      tunnel: string[] ["ARDUINO - ULTRASONIC", "READ ULTRASONIC", ""] -> [w1175] mode=indexing
                      n419 = Enqueue Element(queue=w1177, element=w1175) -> (queue out=w1176:refnum<queue>)  [unwired: 2 in, 2 out]
                    }
                  }
                }
                n420 = Or(x=w1160, y=w1159) -> (x .or. y?=w1162:bool)
                n421 = Select(t=State_Type_Definitions."True Stop" ("Enum"), s=w1159, f=State_Type_Definitions."True Stop" ("Enum")) -> (s? t:f=w1156:T6)
                n422 = Select(t=w1156, s=w1162, f=State_Type_Definitions."Task 5H: RAISE ARM" ("Enum")) -> (s? t:f=w1161:T6)
              }
              frame "Exit" {
                n423 = for {
                  shift-right: [w1184] -> w1181
                  shift-left: w1178 -> [w1185]
                  tunnel: string[] ["STOP", "RESET ENCODERS", "RESET YAW", "ARDUINO MODE 0"] -> [w1183] mode=indexing
                  n424 = Enqueue Element(queue=w1185, element=w1183) -> (queue out=w1184:refnum<queue>)  [unwired: 2 in, 2 out]
                }
              }
            }
          }
          frame 24 {
            # ">>> yStepper command>>>"
            n425 = Dequeue Element(queue=w1194, timeout in ms (-1)=w1193, error in (no error)=w1192) -> (element=w1199:T7)  [unwired: 3 out]
            n426 = Equal?(x=w1190, y=u8 60) -> (x = y?=w1189:bool)
            n427 = case shown="\"None\", Default" w1199 {
              tunnel: [w1206 State_Type_Definitions."True Stop" ("Enum")] -> w1197
              tunnel: [w1205 w1223] -> w1196
              tunnel: [State_Type_Definitions."Idle" ("Enum") State_Type_Definitions."Shutdown" ("Enum")] -> w1198
              tunnel: w1195 -> [w1201 _]
              tunnel: w1191 -> [w1203 _]
              tunnel: w1189 -> [w1200 _]
              frame "None", Default {
                n428 = case shown="False" w1200 {
                  tunnel: [w1211 w1217] -> w1205
                  tunnel: w1203 -> [w1209 w1215]
                  frame False {
                    n429 = for {
                      tunnel: string[] ["Z STEPPER CAM HEIGHT", "READ STEPPER VALUES"] ("element") -> [w1212] mode=indexing
                      shift-right: [w1214] -> w1211
                      shift-left: w1209 -> [w1213]
                      n430 = Enqueue Element(queue=w1213, element=w1212) -> (queue out=w1214:refnum<queue>)  [unwired: 2 in, 2 out]
                    }
                  }
                  frame True {
                    n431 = for {
                      shift-right: [w1219] -> w1217
                      shift-left: w1215 -> [w1220]
                      tunnel: string[] ["CAM ACQ", "OPEN LOG CAM"] -> [w1218] mode=indexing
                      n432 = Enqueue Element(queue=w1220, element=w1218) -> (queue out=w1219:refnum<queue>)  [unwired: 2 in, 2 out]
                    }
                  }
                }
                n433 = Or(x=w1200, y=w1201) -> (x .or. y?=w1202:bool)
                n434 = Select(t=State_Type_Definitions."Task 6_B" ("Enum"), s=w1202, f=State_Type_Definitions."Task 6_A" ("Enum")) -> (s? t:f=w1206:T6)
              }
              frame "Exit" {
                n435 = for {
                  shift-right: [w1226] -> w1223
                  shift-left: _ -> [w1227]
                  tunnel: string[] ["STOP", "RESET ENCODERS", "RESET YAW", "ARDUINO MODE 0"] -> [w1225] mode=indexing
                  n436 = Enqueue Element(queue=w1227, element=w1225) -> (queue out=w1226:refnum<queue>)  [unwired: 2 in, 2 out]
                }
              }
            }
          }
          frame 25 {
            # ">>> yStepper command>>>"
            n437 = Dequeue Element(queue=w1238, timeout in ms (-1)=w1236, error in (no error)=w1237) -> (element=w1235:T7)  [unwired: 3 out]
            n438 = case shown="\"None\", Default" w1235 {
              tunnel: [w1245 State_Type_Definitions."True Stop" ("Enum")] -> w1231
              tunnel: [w1244 w1263] -> w1239
              tunnel: [State_Type_Definitions."Idle" ("Enum") State_Type_Definitions."Shutdown" ("Enum")] -> w1232
              tunnel: w1234 -> [w1240 _]
              tunnel: w1233 -> [w1242 _]
              tunnel: w1230 -> [w1241 w1260]
              frame "None", Default {
                # ">> Manual override >>"
                n439 = case shown="True" w1242 {
                  tunnel: [w1250 w1256] -> w1244
                  tunnel: w1241 -> [w1249 w1254]
                  frame False {
                    n440 = for {
                      shift-right: [w1253] -> w1250
                      shift-left: w1249 -> [w1252]
                      tunnel: string[] ["CAM ACQ", "PROCESS IMAGE", "OPEN CLAW"] -> [w1251] mode=indexing
                      n441 = Enqueue Element(queue=w1252, element=w1251) -> (queue out=w1253:refnum<queue>)  [unwired: 2 in, 2 out]
                    }
                  }
                  frame True {
                    n442 = for {
                      shift-right: [w1258] -> w1256
                      shift-left: w1254 -> [w1259]
                      tunnel: string[] ["CAM ACQ", "PROCESS IMAGE", "CLOSE CLAW"] -> [w1257] mode=indexing
                      n443 = Enqueue Element(queue=w1259, element=w1257) -> (queue out=w1258:refnum<queue>)  [unwired: 2 in, 2 out]
                    }
                  }
                }
                n444 = Select(t=State_Type_Definitions."True Stop" ("Enum"), s=w1240, f=State_Type_Definitions."Task 6_B" ("Enum")) -> (s? t:f=w1245:T6)
              }
              frame "Exit" {
                # ">> State after true stop >>"
                # ">> Goes to true stop >>"
                n445 = for {
                  shift-right: [w1266] -> w1263
                  shift-left: w1260 -> [w1267]
                  tunnel: string[] ["STOP", "RESET ENCODERS", "RESET YAW", ""] -> [w1265] mode=indexing
                  n446 = Enqueue Element(queue=w1267, element=w1265) -> (queue out=w1266:refnum<queue>)  [unwired: 2 in, 2 out]
                }
              }
            }
          }
          frame 26 {
          }
          frame 27 {
            # ">>> yStepper command>>>"
            # ">> Manual override >>"
            n447 = Dequeue Element(queue=w1282, timeout in ms (-1)=w1281, error in (no error)=w1283) -> (element=w1280:T7)  [unwired: 3 out]
            n448 = Equal?(x=w1279, y=u8 60) -> (x = y?=w1277:bool)
            n449 = case shown="\"None\", Default" w1280 {
              tunnel: [w1293 State_Type_Definitions."True Stop" ("Enum")] -> w1284
              tunnel: [w1296 w1313] -> w1285
              tunnel: [State_Type_Definitions."Idle" ("Enum") State_Type_Definitions."Shutdown" ("Enum")] -> w1286
              tunnel: w1277 -> [w1292 _]
              tunnel: w1276 -> [w1291 _]
              tunnel: w1275 -> [w1287 w1310]
              frame "None", Default {
                # "Stays in Task 5_A until stepper reaches desired \nheight"
                # "T: Go back to idle, F: Continue with task\""
                # ">> Manual override >>"
                n450 = case shown="True" w1292 {
                  tunnel: [w1300 w1306] -> w1296
                  tunnel: w1287 -> [w1298 w1304]
                  frame False {
                    n451 = for {
                      tunnel: string[] ["Z STEPPER CAM HEIGHT", "READ STEPPER VALUES"] ("element") -> [w1301] mode=indexing
                      shift-right: [w1303] -> w1300
                      shift-left: w1298 -> [w1302]
                      n452 = Enqueue Element(queue=w1302, element=w1301) -> (queue out=w1303:refnum<queue>)  [unwired: 2 in, 2 out]
                    }
                  }
                  frame True {
                    n453 = for {
                      shift-right: [w1308] -> w1306
                      shift-left: w1304 -> [w1309]
                      tunnel: string[] ["ARDUINO - ULTRASONIC", "READ ULTRASONIC", ""] -> [w1307] mode=indexing
                      n454 = Enqueue Element(queue=w1309, element=w1307) -> (queue out=w1308:refnum<queue>)  [unwired: 2 in, 2 out]
                    }
                  }
                }
                n455 = Or(x=w1292, y=w1291) -> (x .or. y?=w1294:bool)
                n456 = Select(t=State_Type_Definitions."True Stop" ("Enum"), s=w1291, f=State_Type_Definitions."Task 8B: MOVE TO BOX" ("Enum")) -> (s? t:f=w1288:T6)
                n457 = Select(t=w1288, s=w1294, f=State_Type_Definitions."Task 8A: RAISE ARM" ("Enum")) -> (s? t:f=w1293:T6)
              }
              frame "Exit" {
                n458 = for {
                  shift-right: [w1316] -> w1313
                  shift-left: w1310 -> [w1317]
                  tunnel: string[] ["STOP", "RESET ENCODERS", "RESET YAW", "ARDUINO MODE 0"] -> [w1315] mode=indexing
                  n459 = Enqueue Element(queue=w1317, element=w1315) -> (queue out=w1316:refnum<queue>)  [unwired: 2 in, 2 out]
                }
              }
            }
          }
          frame 28 {
            w1324 = u8 20 ("y")
            # ">>> yStepper command>>>"
            n460 = Less?(x=w1321, y=w1324) -> (x < y?=w1322:bool)
            n461 = Dequeue Element(queue=w1328, timeout in ms (-1)=w1327, error in (no error)=w1329) -> (element=w1326:T7)  [unwired: 3 out]
            n462 = Less?(x=w1320, y=w1324) -> (x < y?=w1323:bool)
            n463 = And(x=w1323, y=w1322) -> (x .and. y?=w1319:bool)
            n464 = case shown="\"None\", Default" w1326 {
              tunnel: [w1341 State_Type_Definitions."True Stop" ("Enum")] -> w1331
              tunnel: [w1344 w1361] -> w1330
              tunnel: [State_Type_Definitions."Idle" ("Enum") State_Type_Definitions."Shutdown" ("Enum")] -> w1332
              tunnel: w1334 -> [w1340 _]
              tunnel: w1333 -> [w1336 w1358]
              tunnel: w1319 -> [w1335 _]
              frame "None", Default {
                # "Stays in Task 5_B to capture image over 5 seconds"
                # "T: Go back to idle, F: Continue with task\""
                # ">> Manual override >>"
                n465 = case shown="True" w1335 {
                  tunnel: [w1348 w1354] -> w1344
                  tunnel: w1336 -> [w1346 w1352]
                  frame False {
                    n466 = for {
                      tunnel: string[] ["FORWARD", "READ ULTRASONIC", "READ NAVX"] ("element") -> [w1349] mode=indexing
                      shift-right: [w1351] -> w1348
                      shift-left: w1346 -> [w1350]
                      n467 = Enqueue Element(queue=w1350, element=w1349) -> (queue out=w1351:refnum<queue>)  [unwired: 2 in, 2 out]
                    }
                  }
                  frame True {
                    n468 = for {
                      shift-right: [w1356] -> w1354
                      shift-left: w1352 -> [w1357]
                      tunnel: string[] ["STOP", "RESET ENCODERS", "OPEN LOG CAM", "SET TIMER 2", "OPEN IMAQ REF"] -> [w1355] mode=indexing
                      n469 = Enqueue Element(queue=w1357, element=w1355) -> (queue out=w1356:refnum<queue>)  [unwired: 2 in, 2 out]
                    }
                  }
                }
                n470 = Or(x=w1335, y=w1340) -> (x .or. y?=w1342:bool)
                n471 = Select(t=State_Type_Definitions."True Stop" ("Enum"), s=w1340, f=State_Type_Definitions."Task 8C: CAM BURST" ("Enum")) -> (s? t:f=w1337:T6)
                n472 = Select(t=w1337, s=w1342, f=State_Type_Definitions."Task 8B: MOVE TO BOX" ("Enum")) -> (s? t:f=w1341:T6)
              }
              frame "Exit" {
                n473 = for {
                  shift-right: [w1364] -> w1361
                  shift-left: w1358 -> [w1365]
                  tunnel: string[] ["STOP", "RESET ENCODERS", "RESET YAW", "ARDUINO MODE 0"] -> [w1363] mode=indexing
                  n474 = Enqueue Element(queue=w1365, element=w1363) -> (queue out=w1364:refnum<queue>)  [unwired: 2 in, 2 out]
                }
              }
            }
          }
          frame 29 {
            # ">>> Motor control cluster >>>"
            # ">>> yStepper command>>>"
            # ">> Manual override >>"
            n475 = Dequeue Element(queue=w1375, timeout in ms (-1)=w1374, error in (no error)=w1373) -> (element=w1372:T7)  [unwired: 3 out]
            n476 = case shown="\"None\", Default" w1372 {
              tunnel: [w1384 State_Type_Definitions."True Stop" ("Enum")] -> w1377
              tunnel: [w1387 w1404] -> w1370
              tunnel: [State_Type_Definitions."Idle" ("Enum") State_Type_Definitions."Shutdown" ("Enum")] -> w1369
              tunnel: w1371 -> [w1378 _]
              tunnel: w1376 -> [w1383 w1401]
              tunnel: w1367 -> [w1382 _]
              frame "None", Default {
                # ">> Is time up? >>"
                # "Determines if object is in range to pick up"
                # ">> Manual override >>"
                n477 = case shown="True" w1382 {
                  tunnel: [w1391 w1397] -> w1387
                  tunnel: w1383 -> [w1389 w1395]
                  frame False {
                    n478 = for {
                      tunnel: string[] ["CAM ACQ", "START TIMER"] ("element") -> [w1392] mode=indexing
                      shift-right: [w1394] -> w1391
                      shift-left: w1389 -> [w1393]
                      n479 = Enqueue Element(queue=w1393, element=w1392) -> (queue out=w1394:refnum<queue>)  [unwired: 2 in, 2 out]
                    }
                  }
                  frame True {
                    n480 = for {
                      shift-right: [w1399] -> w1397
                      shift-left: w1395 -> [w1400]
                      tunnel: string[] ["CAM CLOSE", "PROCESS IMAGE", "SET TIMER 5"] -> [w1398] mode=indexing
                      n481 = Enqueue Element(queue=w1400, element=w1398) -> (queue out=w1399:refnum<queue>)  [unwired: 2 in, 2 out]
                    }
                  }
                }
                n482 = Or(x=w1382, y=w1378) -> (x .or. y?=w1385:bool)
                n483 = Select(t=State_Type_Definitions."True Stop" ("Enum"), s=w1378, f=State_Type_Definitions."Task 8D: PROCESS IMAGE" ("Enum")) -> (s? t:f=w1380:T6)
                n484 = Select(t=w1380, s=w1385, f=State_Type_Definitions."Task 8C: CAM BURST" ("Enum")) -> (s? t:f=w1384:T6)
              }
              frame "Exit" {
                n485 = for {
                  shift-right: [w1407] -> w1404
                  shift-left: w1401 -> [w1408]
                  tunnel: string[] ["STOP", "RESET ENCODERS", "RESET YAW", "ARDUINO MODE 0"] -> [w1406] mode=indexing
                  n486 = Enqueue Element(queue=w1408, element=w1406) -> (queue out=w1407:refnum<queue>)  [unwired: 2 in, 2 out]
                }
              }
            }
          }
          frame 30 {
            # ">>> yStepper command>>>"
            n487 = Dequeue Element(queue=w1415, timeout in ms (-1)=w1414, error in (no error)=w1413) -> (element=w1412:T7)  [unwired: 3 out]
            n488 = case shown="\"None\", Default" w1412 {
              tunnel: [w1427 State_Type_Definitions."True Stop" ("Enum")] -> w1419
              tunnel: [w1430 w1447] -> w1418
              tunnel: [State_Type_Definitions."Idle" ("Enum") State_Type_Definitions."Shutdown" ("Enum")] -> w1420
              tunnel: w1416 -> [w1426 _]
              tunnel: w1417 -> [w1422 w1444]
              tunnel: w1410 -> [w1421 _]
              frame "None", Default {
                # ">> T: Breaks out of state loop; F: Stays in loop>>"
                # ">> Manual override >>"
                # ">> Checks if time is up>>"
                # "Stays in Task 5D until the object is detected"
                # "T: Go back to idle, F: Continue with task\""
                # ">> Manual override >>"
                n489 = case shown="False" w1421 {
                  tunnel: [w1434 w1440] -> w1430
                  tunnel: w1422 -> [w1432 w1438]
                  frame False {
                    n490 = for {
                      tunnel: string[] ["START TIMER", "PROCESS IMAGE", ""] ("element") -> [w1435] mode=indexing
                      shift-right: [w1437] -> w1434
                      shift-left: w1432 -> [w1436]
                      n491 = Enqueue Element(queue=w1436, element=w1435) -> (queue out=w1437:refnum<queue>)  [unwired: 2 in, 2 out]
                    }
                  }
                  frame True {
                    n492 = for {
                      shift-right: [w1442] -> w1440
                      shift-left: w1438 -> [w1443]
                      tunnel: string[] ["RESET ENCODERS", "", ""] -> [w1441] mode=indexing
                      n493 = Enqueue Element(queue=w1443, element=w1441) -> (queue out=w1442:refnum<queue>)  [unwired: 2 in, 2 out]
                    }
                  }
                }
                n494 = Or(x=w1421, y=w1426) -> (x .or. y?=w1428:bool)
                n495 = Select(t=State_Type_Definitions."True Stop" ("Enum"), s=w1426, f=State_Type_Definitions."Task 8E: ROBOT ADJUST" ("Enum")) -> (s? t:f=w1423:T6)
                n496 = Select(t=w1423, s=w1428, f=State_Type_Definitions."Task 8D: PROCESS IMAGE" ("Enum")) -> (s? t:f=w1427:T6)
              }
              frame "Exit" {
                n497 = for {
                  shift-right: [w1450] -> w1447
                  shift-left: w1444 -> [w1451]
                  tunnel: string[] ["STOP", "RESET ENCODERS", "RESET YAW", "ARDUINO MODE 0"] -> [w1449] mode=indexing
                  n498 = Enqueue Element(queue=w1451, element=w1449) -> (queue out=w1450:refnum<queue>)  [unwired: 2 in, 2 out]
                }
              }
            }
          }
          frame 31 {
            # ">>> Motor control cluster >>>"
            # ">>> yStepper command>>>"
            n499 = Dequeue Element(queue=w1467, timeout in ms (-1)=w1466, error in (no error)=w1465) -> (element=w1464:T7)  [unwired: 3 out]
            n500 = Subtract(x=w1462, y=300.0) -> (x-y=w1460:dbl)
            "x-y" <- w1460
            n501 = formula code="if (error < -80 && error >-300){\ndistance = -20;\nxSpeed = -30;\n}\n\nelse if (error <= 61&&error >= -80){\ndistance = -15;\nxSpeed = -30;\n}\n\nelse if (error <= -26 && error >= -60){\ndistance = -10;\nxSpeed = -30;\n}\n\nelse if (error >= -25 && error <= 25){\ndistance = 0;\nxSpeed = 0;\n}\n\nelse if (error >= 51 && error <= 80){\ndistance = 10;\nxSpeed = 30;\n}\n\nelse if (error >= 81 && error <= 100){\ndistance = 15;\nxSpeed = 30;\n}\n\nelse if (error >= 101 && error <= 120){\ndistance = 20;\nxSpeed = 30;\n}\n\nelse if (error >= 121 && error <= 150){\ndistance = 25;\nxSpeed = 30;\n}\n\nelse if (error < 250){\ndistance = 30;\nxSpeed = 30;\n}\n\nelse{\ndistance = 0;\nxSpeed = 0;\n}"("error"=w1460) -> ("distance"=w1455:dbl, "xSpeed"=w1457:dbl)
            n502 = formula code="if (target > 0){\nif (current  >= target)\noutput = 1;\n}\n\nelse if (target == 0){\nif (current == target)\noutput = 1;\n}\n\nelse if (target < 0){\nif (current <= target)\noutput = 1;\n}\n\nelse\noutput = 0;"("target"=w1455, "current"=w1456) -> ("output"=w1454:dbl)
            n503 = Bundle By Name(cluster=w1459, "xSpeed"=w1457) -> (w1458:T8)
            n504 = Equal?(x=w1454, y=1.0) -> (x = y?=w1452:bool)
            n505 = case shown="\"None\", Default" w1464 {
              tunnel: [w1479 State_Type_Definitions."True Stop" ("Enum")] -> w1471
              tunnel: [w1482 w1499] -> w1470
              tunnel: [State_Type_Definitions."Idle" ("Enum") State_Type_Definitions."Shutdown" ("Enum")] -> w1472
              tunnel: w1468 -> [w1478 _]
              tunnel: w1469 -> [w1474 w1496]
              tunnel: w1452 -> [w1473 _]
              frame "None", Default {
                # ">> T: Breaks out of state loop; F: Stays in loop>>"
                # ">> Manual override >>"
                # ">> Checks if time is up>>"
                # "Stays in Task 5D until the object is detected"
                # "T: Go back to idle, F: Continue with task\""
                # ">> Manual override >>"
                n506 = case shown="False" w1473 {
                  tunnel: [w1486 w1492] -> w1482
                  tunnel: w1474 -> [w1484 w1490]
                  frame False {
                    n507 = for {
                      tunnel: string[] ["X AXIS - SLOW", "READ ENCODERS", "READ NAVX"] ("element") -> [w1487] mode=indexing
                      shift-right: [w1489] -> w1486
                      shift-left: w1484 -> [w1488]
                      n508 = Enqueue Element(queue=w1488, element=w1487) -> (queue out=w1489:refnum<queue>)  [unwired: 2 in, 2 out]
                    }
                  }
                  frame True {
                    n509 = for {
                      shift-right: [w1494] -> w1492
                      shift-left: w1490 -> [w1495]
                      tunnel: string[] ["SET TIMER 2", "STOP", "READ STEPPER VALUES", ""] -> [w1493] mode=indexing
                      n510 = Enqueue Element(queue=w1495, element=w1493) -> (queue out=w1494:refnum<queue>)  [unwired: 2 in, 2 out]
                    }
                  }
                }
                n511 = Or(x=w1473, y=w1478) -> (x .or. y?=w1480:bool)
                n512 = Select(t=State_Type_Definitions."True Stop" ("Enum"), s=w1478, f=State_Type_Definitions."Task 8H: ARM ADJUST" ("Enum")) -> (s? t:f=w1475:T6)
                n513 = Select(t=w1475, s=w1480, f=State_Type_Definitions."Task 8E: ROBOT ADJUST" ("Enum")) -> (s? t:f=w1479:T6)
              }
              frame "Exit" {
                n514 = for {
                  shift-right: [w1502] -> w1499
                  shift-left: w1496 -> [w1503]
                  tunnel: string[] ["STOP", "RESET ENCODERS", "RESET YAW", "ARDUINO MODE 0"] -> [w1501] mode=indexing
                  n515 = Enqueue Element(queue=w1503, element=w1501) -> (queue out=w1502:refnum<queue>)  [unwired: 2 in, 2 out]
                }
              }
            }
          }
          frame 32 {
            # ">>> Motor control cluster >>>"
            # ">>> yStepper command>>>"
            # ">> Manual override >>"
            n516 = Dequeue Element(queue=w1513, timeout in ms (-1)=w1512, error in (no error)=w1511) -> (element=w1510:T7)  [unwired: 3 out]
            n517 = case shown="\"None\", Default" w1510 {
              tunnel: [w1522 State_Type_Definitions."True Stop" ("Enum")] -> w1515
              tunnel: [w1525 w1542] -> w1508
              tunnel: [State_Type_Definitions."Idle" ("Enum") State_Type_Definitions."Shutdown" ("Enum")] -> w1507
              tunnel: w1509 -> [w1516 _]
              tunnel: w1514 -> [w1521 w1539]
              tunnel: w1505 -> [w1520 _]
              frame "None", Default {
                # ">> Is time up? >>"
                # "Determines if object is in range to pick up"
                # ">> Manual override >>"
                n518 = case shown="True" w1520 {
                  tunnel: [w1529 w1535] -> w1525
                  tunnel: w1521 -> [w1527 w1533]
                  frame False {
                    n519 = for {
                      tunnel: string[] ["CAM ACQ", "START TIMER"] ("element") -> [w1530] mode=indexing
                      shift-right: [w1532] -> w1529
                      shift-left: w1527 -> [w1531]
                      n520 = Enqueue Element(queue=w1531, element=w1530) -> (queue out=w1532:refnum<queue>)  [unwired: 2 in, 2 out]
                    }
                  }
                  frame True {
                    n521 = for {
                      shift-right: [w1537] -> w1535
                      shift-left: w1533 -> [w1538]
                      tunnel: string[] ["CAM CLOSE", "PROCESS IMAGE", "SET TIMER 3"] -> [w1536] mode=indexing
                      n522 = Enqueue Element(queue=w1538, element=w1536) -> (queue out=w1537:refnum<queue>)  [unwired: 2 in, 2 out]
                    }
                  }
                }
                n523 = Or(x=w1520, y=w1516) -> (x .or. y?=w1523:bool)
                n524 = Select(t=State_Type_Definitions."True Stop" ("Enum"), s=w1516, f=State_Type_Definitions."Task 8G: PROCESS IMAGE 2" ("Enum")) -> (s? t:f=w1518:T6)
                n525 = Select(t=w1518, s=w1523, f=State_Type_Definitions."Task 8F: CAM BURST 2" ("Enum")) -> (s? t:f=w1522:T6)
              }
              frame "Exit" {
                n526 = for {
                  shift-right: [w1545] -> w1542
                  shift-left: w1539 -> [w1546]
                  tunnel: string[] ["STOP", "RESET ENCODERS", "RESET YAW", "ARDUINO MODE 0"] -> [w1544] mode=indexing
                  n527 = Enqueue Element(queue=w1546, element=w1544) -> (queue out=w1545:refnum<queue>)  [unwired: 2 in, 2 out]
                }
              }
            }
          }
          frame 33 {
            # ">>> yStepper command>>>"
            n528 = Dequeue Element(queue=w1553, timeout in ms (-1)=w1552, error in (no error)=w1551) -> (element=w1550:T7)  [unwired: 3 out]
            n529 = case shown="\"None\", Default" w1550 {
              tunnel: [w1565 State_Type_Definitions."True Stop" ("Enum")] -> w1557
              tunnel: [w1568 w1585] -> w1556
              tunnel: [State_Type_Definitions."Idle" ("Enum") State_Type_Definitions."Shutdown" ("Enum")] -> w1558
              tunnel: w1554 -> [w1564 _]
              tunnel: w1555 -> [w1560 w1582]
              tunnel: w1548 -> [w1559 _]
              frame "None", Default {
                # ">> T: Breaks out of state loop; F: Stays in loop>>"
                # ">> Manual override >>"
                # ">> Checks if time is up>>"
                # "Stays in Task 5D until the object is detected"
                # "T: Go back to idle, F: Continue with task\""
                # ">> Manual override >>"
                n530 = case shown="False" w1559 {
                  tunnel: [w1572 w1578] -> w1568
                  tunnel: w1560 -> [w1570 w1576]
                  frame False {
                    n531 = for {
                      tunnel: string[] ["START TIMER", "PROCESS IMAGE", ""] ("element") -> [w1573] mode=indexing
                      shift-right: [w1575] -> w1572
                      shift-left: w1570 -> [w1574]
                      n532 = Enqueue Element(queue=w1574, element=w1573) -> (queue out=w1575:refnum<queue>)  [unwired: 2 in, 2 out]
                    }
                  }
                  frame True {
                    n533 = for {
                      shift-right: [w1580] -> w1578
                      shift-left: w1576 -> [w1581]
                      tunnel: string[] ["READ STEPPER VALUES", "Y STEPPER CONTROL", ""] -> [w1579] mode=indexing
                      n534 = Enqueue Element(queue=w1581, element=w1579) -> (queue out=w1580:refnum<queue>)  [unwired: 2 in, 2 out]
                    }
                  }
                }
                n535 = Or(x=w1559, y=w1564) -> (x .or. y?=w1566:bool)
                n536 = Select(t=State_Type_Definitions."True Stop" ("Enum"), s=w1564, f=State_Type_Definitions."Task 8H: ARM ADJUST" ("Enum")) -> (s? t:f=w1561:T6)
                n537 = Select(t=w1561, s=w1566, f=State_Type_Definitions."Task 8G: PROCESS IMAGE 2" ("Enum")) -> (s? t:f=w1565:T6)
              }
              frame "Exit" {
                n538 = for {
                  shift-right: [w1588] -> w1585
                  shift-left: w1582 -> [w1589]
                  tunnel: string[] ["STOP", "RESET ENCODERS", "RESET YAW", "ARDUINO MODE 0"] -> [w1587] mode=indexing
                  n539 = Enqueue Element(queue=w1589, element=w1587) -> (queue out=w1588:refnum<queue>)  [unwired: 2 in, 2 out]
                }
              }
            }
          }
          frame 34 {
            # ">>> yStepper command>>>"
            n540 = Dequeue Element(queue=w1602, timeout in ms (-1)=w1603, error in (no error)=w1604) -> (element=w1606:T7)  [unwired: 3 out]
            n541 = formula code="if (pos <= 81)\ny = 40;\n\nelse if (pos >= 81 &&pos <= 120)\ny = 37;\n\nelse if (pos >= 121 && pos <= 140)\ny = 28;\n\nelse if (pos >= 141 && pos <= 170)\ny = 25;\n\nelse if (pos >= 171 &&pos <= 200) \ny = 20;\n\nelse if (pos >= 201&& pos <= 210)\ny = 15;\n\nelse if (pos >= 211 && pos <= 230)\ny = 10;\n\nelse if (pos >= 231 && pos <= 320)\ny = 8;\n\nelse if (pos > 320)\ny = 0;"("pos"=w1594) -> ("y"=w1597:dbl)
            n542 = To Unsigned Byte Integer(number=w1597) -> (unsigned 8bit integer=w1592:u8)
            n543 = Equal?(x=w1593, y=w1592) -> (x = y?=w1591:bool)
            n544 = case shown="\"None\", Default" w1606 {
              tunnel: [w1613 State_Type_Definitions."True Stop" ("Enum")] -> w1600
              tunnel: [w1616 w1633] -> w1598
              tunnel: [State_Type_Definitions."Idle" ("Enum") State_Type_Definitions."Shutdown" ("Enum")] -> w1599
              tunnel: w1605 -> [w1612 _]
              tunnel: w1601 -> [w1608 w1630]
              tunnel: w1591 -> [w1607 _]
              frame "None", Default {
                # ">> T: Breaks out of state loop; F: Stays in loop>>"
                # ">> Manual override >>"
                # ">> Checks if time is up>>"
                # "Stays in Task 5D until the object is detected"
                # "T: Go back to idle, F: Continue with task\""
                # ">> Manual override >>"
                n545 = case shown="False" w1607 {
                  tunnel: [w1620 w1626] -> w1616
                  tunnel: w1608 -> [w1618 w1624]
                  frame False {
                    n546 = for {
                      tunnel: string[] ["READ STEPPER VALUES", "Y STEPPER CONTROL", ""] ("element") -> [w1621] mode=indexing
                      shift-right: [w1623] -> w1620
                      shift-left: w1618 -> [w1622]
                      n547 = Enqueue Element(queue=w1622, element=w1621) -> (queue out=w1623:refnum<queue>)  [unwired: 2 in, 2 out]
                    }
                  }
                  frame True {
                    n548 = for {
                      shift-right: [w1628] -> w1626
                      shift-left: w1624 -> [w1629]
                      tunnel: string[] ["DISPOSE BUFFERS", "READ STEPPER VALUES", ""] -> [w1627] mode=indexing
                      n549 = Enqueue Element(queue=w1629, element=w1627) -> (queue out=w1628:refnum<queue>)  [unwired: 2 in, 2 out]
                    }
                  }
                }
                n550 = Or(x=w1607, y=w1612) -> (x .or. y?=w1614:bool)
                n551 = Select(t=State_Type_Definitions."True Stop" ("Enum"), s=w1612, f=State_Type_Definitions."Task 8I: ARM GRAB HEIGHT" ("Enum")) -> (s? t:f=w1609:T6)
                n552 = Select(t=w1609, s=w1614, f=State_Type_Definitions."Task 8H: ARM ADJUST" ("Enum")) -> (s? t:f=w1613:T6)
              }
              frame "Exit" {
                n553 = for {
                  shift-right: [w1636] -> w1633
                  shift-left: w1630 -> [w1637]
                  tunnel: string[] ["STOP", "RESET ENCODERS", "RESET YAW", "ARDUINO MODE 0"] -> [w1635] mode=indexing
                  n554 = Enqueue Element(queue=w1637, element=w1635) -> (queue out=w1636:refnum<queue>)  [unwired: 2 in, 2 out]
                }
              }
            }
            n555 = Bundle By Name(cluster=w1596, "yStepper desired"=w1592) -> (w1595:T10)
          }
          frame 35 {
            # ">>> Motor control cluster >>>"
            # ">>> yStepper command>>>"
            # ">> Manual override >>"
            n556 = Dequeue Element(queue=w1647, timeout in ms (-1)=w1646, error in (no error)=w1648) -> (element=w1645:T7)  [unwired: 3 out]
            n557 = Equal?(x=w1644, y=u8 1) -> (x = y?=w1642:bool)
            n558 = case shown="\"None\", Default" w1645 {
              tunnel: [w1658 State_Type_Definitions."True Stop" ("Enum")] -> w1649
              tunnel: [w1661 w1678] -> w1650
              tunnel: [State_Type_Definitions."Idle" ("Enum") State_Type_Definitions."Shutdown" ("Enum")] -> w1651
              tunnel: w1642 -> [w1657 _]
              tunnel: w1641 -> [w1656 _]
              tunnel: w1640 -> [w1652 w1675]
              frame "None", Default {
                # "Stays in Task 5F until stepper reaches desired \nheight"
                # "T: Go back to idle, F: Continue with task\""
                # ">> Manual override >>"
                n559 = case shown="True" w1657 {
                  tunnel: [w1665 w1671] -> w1661
                  tunnel: w1652 -> [w1663 w1669]
                  frame False {
                    n560 = for {
                      tunnel: string[] ["Z STEPPER GRAB HEIGHT", "READ STEPPER VALUES"] ("element") -> [w1666] mode=indexing
                      shift-right: [w1668] -> w1665
                      shift-left: w1663 -> [w1667]
                      n561 = Enqueue Element(queue=w1667, element=w1666) -> (queue out=w1668:refnum<queue>)  [unwired: 2 in, 2 out]
                    }
                  }
                  frame True {
                    n562 = for {
                      shift-right: [w1673] -> w1671
                      shift-left: w1669 -> [w1674]
                      tunnel: string[] ["SET TIMER 2", "CLOSE CLAW", ""] -> [w1672] mode=indexing
                      n563 = Enqueue Element(queue=w1674, element=w1672) -> (queue out=w1673:refnum<queue>)  [unwired: 2 in, 2 out]
                    }
                  }
                }
                n564 = Or(x=w1657, y=w1656) -> (x .or. y?=w1659:bool)
                n565 = Select(t=State_Type_Definitions."True Stop" ("Enum"), s=w1656, f=State_Type_Definitions."Task 8J: CLOSE CLAW" ("Enum")) -> (s? t:f=w1653:T6)
                n566 = Select(t=w1653, s=w1659, f=State_Type_Definitions."Task 8I: ARM GRAB HEIGHT" ("Enum")) -> (s? t:f=w1658:T6)
              }
              frame "Exit" {
                n567 = for {
                  shift-right: [w1681] -> w1678
                  shift-left: w1675 -> [w1682]
                  tunnel: string[] ["STOP", "RESET ENCODERS", "RESET YAW", "ARDUINO MODE 0"] -> [w1680] mode=indexing
                  n568 = Enqueue Element(queue=w1682, element=w1680) -> (queue out=w1681:refnum<queue>)  [unwired: 2 in, 2 out]
                }
              }
            }
          }
          frame 36 {
            # ">>> yStepper command>>>"
            # ">> Manual override >>"
            n569 = Dequeue Element(queue=w1692, timeout in ms (-1)=w1691, error in (no error)=w1690) -> (element=w1689:T7)  [unwired: 3 out]
            n570 = case shown="\"None\", Default" w1689 {
              tunnel: [w1701 State_Type_Definitions."True Stop" ("Enum")] -> w1694
              tunnel: [w1704 w1721] -> w1687
              tunnel: [State_Type_Definitions."Idle" ("Enum") State_Type_Definitions."Shutdown" ("Enum")] -> w1686
              tunnel: w1688 -> [w1695 _]
              tunnel: w1693 -> [w1700 w1718]
              tunnel: w1684 -> [w1699 _]
              frame "None", Default {
                # ">> Is time up? >>"
                # "Determines if object is in range to pick up"
                # ">> Manual override >>"
                n571 = case shown="True" w1699 {
                  tunnel: [w1708 w1714] -> w1704
                  tunnel: w1700 -> [w1706 w1712]
                  frame False {
                    n572 = for {
                      tunnel: string[] ["CLOSE CLAW", "START TIMER"] ("element") -> [w1709] mode=indexing
                      shift-right: [w1711] -> w1708
                      shift-left: w1706 -> [w1710]
                      n573 = Enqueue Element(queue=w1710, element=w1709) -> (queue out=w1711:refnum<queue>)  [unwired: 2 in, 2 out]
                    }
                  }
                  frame True {
                    n574 = for {
                      shift-right: [w1716] -> w1714
                      shift-left: w1712 -> [w1717]
                      tunnel: string[] ["READ STEPPER VALUES", "", ""] -> [w1715] mode=indexing
                      n575 = Enqueue Element(queue=w1717, element=w1715) -> (queue out=w1716:refnum<queue>)  [unwired: 2 in, 2 out]
                    }
                  }
                }
                n576 = Or(x=w1699, y=w1695) -> (x .or. y?=w1702:bool)
                n577 = Select(t=State_Type_Definitions."True Stop" ("Enum"), s=w1695, f=State_Type_Definitions."Task 8K: RAISE MY SWORD" ("Enum")) -> (s? t:f=w1697:T6)
                n578 = Select(t=w1697, s=w1702, f=State_Type_Definitions."Task 8J: CLOSE CLAW" ("Enum")) -> (s? t:f=w1701:T6)
              }
              frame "Exit" {
                n579 = for {
                  shift-right: [w1724] -> w1721
                  shift-left: w1718 -> [w1725]
                  tunnel: string[] ["STOP", "RESET ENCODERS", "RESET YAW", "ARDUINO MODE 0"] -> [w1723] mode=indexing
                  n580 = Enqueue Element(queue=w1725, element=w1723) -> (queue out=w1724:refnum<queue>)  [unwired: 2 in, 2 out]
                }
              }
            }
          }
          frame 37 {
            # ">>> yStepper command>>>"
            # ">> Manual override >>"
            n581 = Dequeue Element(queue=w1735, timeout in ms (-1)=w1734, error in (no error)=w1736) -> (element=w1733:T7)  [unwired: 3 out]
            n582 = Equal?(x=w1732, y=u8 60) -> (x = y?=w1730:bool)
            n583 = case shown="\"None\", Default" w1733 {
              tunnel: [w1746 State_Type_Definitions."True Stop" ("Enum")] -> w1737
              tunnel: [w1749 w1766] -> w1738
              tunnel: [State_Type_Definitions."Idle" ("Enum") State_Type_Definitions."Shutdown" ("Enum")] -> w1739
              tunnel: w1730 -> [w1745 _]
              tunnel: w1729 -> [w1744 _]
              tunnel: w1728 -> [w1740 w1763]
              frame "None", Default {
                # "Stays in Task 5_A until stepper reaches desired \nheight"
                # "T: Go back to idle, F: Continue with task\""
                # ">> Manual override >>"
                n584 = case shown="True" w1745 {
                  tunnel: [w1753 w1759] -> w1749
                  tunnel: w1740 -> [w1751 w1757]
                  frame False {
                    n585 = for {
                      tunnel: string[] ["Z STEPPER CAM HEIGHT", "READ STEPPER VALUES"] ("element") -> [w1754] mode=indexing
                      shift-right: [w1756] -> w1753
                      shift-left: w1751 -> [w1755]
                      n586 = Enqueue Element(queue=w1755, element=w1754) -> (queue out=w1756:refnum<queue>)  [unwired: 2 in, 2 out]
                    }
                  }
                  frame True {
                    n587 = for {
                      shift-right: [w1761] -> w1759
                      shift-left: w1757 -> [w1762]
                      tunnel: string[] ["CAM CLOSE", "DISPOSE ALL BUFFERS", ""] -> [w1760] mode=indexing
                      n588 = Enqueue Element(queue=w1762, element=w1760) -> (queue out=w1761:refnum<queue>)  [unwired: 2 in, 2 out]
                    }
                  }
                }
                n589 = Or(x=w1745, y=w1744) -> (x .or. y?=w1747:bool)
                n590 = Select(t=State_Type_Definitions."True Stop" ("Enum"), s=w1744, f=State_Type_Definitions."True Stop" ("Enum")) -> (s? t:f=w1741:T6)
                n591 = Select(t=w1741, s=w1747, f=State_Type_Definitions."Task 8K: RAISE MY SWORD" ("Enum")) -> (s? t:f=w1746:T6)
              }
              frame "Exit" {
                n592 = for {
                  shift-right: [w1769] -> w1766
                  shift-left: w1763 -> [w1770]
                  tunnel: string[] ["STOP", "RESET ENCODERS", "RESET YAW", "ARDUINO MODE 0"] -> [w1768] mode=indexing
                  n593 = Enqueue Element(queue=w1770, element=w1768) -> (queue out=w1769:refnum<queue>)  [unwired: 2 in, 2 out]
                }
              }
            }
          }
          frame 38 {
            # ">> Stepper height reeached >>"
            # ">>> yStepper command>>>"
            # ">> Manual override >>"
            n594 = Dequeue Element(queue=w1781, timeout in ms (-1)=w1776, error in (no error)=w1780) -> (element=w1784:T7)  [unwired: 3 out]
            n595 = Equal?(x=w1778, y=u8 60) -> (x = y?=w1782:bool)
            n596 = case shown="\"None\", Default" w1784 {
              tunnel: [w1795 State_Type_Definitions."True Stop" ("Enum")] -> w1774
              tunnel: [w1793 w1810] -> w1773
              tunnel: w1777 -> [w1792 _]
              tunnel: w1779 -> [w1786 _]
              tunnel: [State_Type_Definitions."Idle" ("Enum") State_Type_Definitions."Shutdown" ("Enum")] -> w1775
              tunnel: w1782 -> [w1785 _]
              frame "None", Default {
                # ">> WIill proceed to part ii if not manual override >>"
                # ">>If ENABLE or Trigger is set to true>>"
                n597 = Or(x=w1785, y=w1786) -> (x .or. y?=w1787:bool)
                n598 = case shown="True" w1785 {
                  tunnel: [w1798 w1804] -> w1793
                  tunnel: w1792 -> [w1797 w1803]
                  frame False {
                    n599 = for {
                      shift-right: [w1800] -> w1798
                      shift-left: w1797 -> [w1801]
                      tunnel: string[] ["Z STEPPER CAM HEIGHT", "READ STEPPER VALUES"] ("element") -> [w1799] mode=indexing
                      n600 = Enqueue Element(queue=w1801, element=w1799) -> (queue out=w1800:refnum<queue>)  [unwired: 2 in, 2 out]
                    }
                  }
                  frame True {
                    n601 = for {
                      shift-right: [w1806] -> w1804
                      shift-left: w1803 -> [w1807]
                      tunnel: string[] ["ARDUINO - ULTRASONIC", "READ ULTRASONIC", "", "", "", ""] -> [w1805] mode=indexing
                      n602 = Enqueue Element(queue=w1807, element=w1805) -> (queue out=w1806:refnum<queue>)  [unwired: 2 in, 2 out]
                    }
                  }
                }
                n603 = Select(t=State_Type_Definitions."True Stop" ("Enum"), s=w1786, f=State_Type_Definitions."Task 9B: Rotate to Angle" ("Enum")) -> (s? t:f=w1789:T6)
                n604 = Select(t=w1789, s=w1787, f=State_Type_Definitions."Task 9A: Raise Arm" ("Enum")) -> (s? t:f=w1795:T6)
              }
              frame "Exit" {
                n605 = for {
                  shift-right: [w1813] -> w1810
                  shift-left: _ -> [w1814]
                  tunnel: string[] ["STOP", "RESET ENCODERS", "RESET YAW", ""] -> [w1812] mode=indexing
                  n606 = Enqueue Element(queue=w1814, element=w1812) -> (queue out=w1813:refnum<queue>)  [unwired: 2 in, 2 out]
                }
              }
            }
          }
          frame 39 {
            # ">>> yStepper command>>>"
            n607 = Dequeue Element(queue=w1827, timeout in ms (-1)=w1826, error in (no error)=w1825) -> (element=w1829:T7)  [unwired: 3 out]
            n608 = In Range and Coerce(upper limit=65.0, x=w1819, lower limit=55.0) -> (In Range?=w1816:bool)  [unwired: 1 out]
            n609 = case shown="\"None\", Default" w1829 {
              tunnel: w1820 -> [w1832 _]
              tunnel: [w1840 State_Type_Definitions."True Stop" ("Enum")] -> w1822
              tunnel: w1828 -> [w1838 w1856]
              tunnel: [w1837 w1855] -> w1821
              tunnel: [State_Type_Definitions."Idle" ("Enum") State_Type_Definitions."Shutdown" ("Enum")] -> w1823
              tunnel: w1816 -> [w1830 _]
              frame "None", Default {
                n610 = Or(x=w1830, y=w1832) -> (x .or. y?=w1831:bool)
                n611 = case shown="True" w1830 {
                  tunnel: w1838 -> [w1843 w1849]
                  tunnel: [w1842 w1847] -> w1837
                  frame False {
                    n612 = for {
                      shift-right: [w1845] -> w1842
                      shift-left: w1843 -> [w1846]
                      tunnel: string[] ["READ NAVX", "R-ACW"] ("element") -> [w1844] mode=indexing
                      n613 = Enqueue Element(queue=w1846, element=w1844) -> (queue out=w1845:refnum<queue>)  [unwired: 2 in, 2 out]
                    }
                  }
                  frame True {
                    n614 = for {
                      shift-right: [w1851] -> w1847
                      shift-left: w1849 -> [w1852]
                      tunnel: string[] ["STOP", "RESET ENCODERS", "RESET YAW", ""] -> [w1850] mode=indexing
                      n615 = Enqueue Element(queue=w1852, element=w1850) -> (queue out=w1851:refnum<queue>)  [unwired: 2 in, 2 out]
                    }
                  }
                }
                n616 = Select(t=State_Type_Definitions."True Stop" ("Enum"), s=w1832, f=State_Type_Definitions."Task 9C: Rotation alignmnet") -> (s? t:f=w1834:u16)
                n617 = Select(t=w1834, s=w1831, f=State_Type_Definitions."Task 9B: Rotate to Angle" ("Enum")) -> (s? t:f=w1840:u16)
              }
              frame "Exit" {
                n618 = for {
                  shift-right: [w1859] -> w1855
                  shift-left: w1856 -> [w1860]
                  tunnel: string[] ["STOP", "RESET ENCODERS", "RESET YAW", ""] -> [w1858] mode=indexing
                  n619 = Enqueue Element(queue=w1860, element=w1858) -> (queue out=w1859:refnum<queue>)  [unwired: 2 in, 2 out]
                }
              }
            }
          }
          frame 39 {
            # ">>> yStepper command>>>"
            n620 = Dequeue Element(queue=w1870, timeout in ms (-1)=w1869, error in (no error)=w1868) -> (element=w1871:T7)  [unwired: 3 out]
            n621 = case shown="\"None\", Default" w1871 {
              tunnel: w1866 -> [w1872 _]
              tunnel: [w1880 State_Type_Definitions."True Stop" ("Enum")] -> w1863
              tunnel: w1867 -> [w1878 w1896]
              tunnel: [w1877 w1895] -> w1862
              tunnel: [State_Type_Definitions."Idle" ("Enum") State_Type_Definitions."Shutdown" ("Enum")] -> w1865
              frame "None", Default {
                n622 = case shown="False" w1872 {
                  tunnel: w1878 -> [w1883 w1889]
                  tunnel: [w1882 w1887] -> w1877
                  frame False {
                    n623 = for {
                      shift-right: [w1885] -> w1882
                      shift-left: w1883 -> [w1886]
                      tunnel: string[] ["READ IR", "FORWARD - IR ASSIST"] ("element") -> [w1884] mode=indexing
                      n624 = Enqueue Element(queue=w1886, element=w1884) -> (queue out=w1885:refnum<queue>)  [unwired: 2 in, 2 out]
                    }
                  }
                  frame True {
                    n625 = for {
                      shift-right: [w1891] -> w1887
                      shift-left: w1889 -> [w1892]
                      tunnel: string[] ["STOP", "RESET ENCODERS", "RESET YAW", ""] -> [w1890] mode=indexing
                      n626 = Enqueue Element(queue=w1892, element=w1890) -> (queue out=w1891:refnum<queue>)  [unwired: 2 in, 2 out]
                    }
                  }
                }
                n627 = Select(t=State_Type_Definitions."True Stop" ("Enum"), s=w1872, f=State_Type_Definitions."True Stop") -> (s? t:f=w1874:T6)
                n628 = Select(t=w1874, s=w1872, f=State_Type_Definitions."Task 9C: Rotation alignmnet" ("Enum")) -> (s? t:f=w1880:u16)
              }
              frame "Exit" {
                n629 = for {
                  shift-right: [w1899] -> w1895
                  shift-left: w1896 -> [w1900]
                  tunnel: string[] ["STOP", "RESET ENCODERS", "RESET YAW", ""] -> [w1898] mode=indexing
                  n630 = Enqueue Element(queue=w1900, element=w1898) -> (queue out=w1899:refnum<queue>)  [unwired: 2 in, 2 out]
                }
              }
            }
          }
          frame 40 {
            # ">> Stepper height reeached >>"
            # ">>> yStepper command>>>"
            # ">> Manual override >>"
            n631 = Dequeue Element(queue=w1911, timeout in ms (-1)=w1906, error in (no error)=w1910) -> (element=w1914:T7)  [unwired: 3 out]
            n632 = Equal?(x=w1908, y=u8 40) -> (x = y?=w1912:bool)
            n633 = case shown="\"None\", Default" w1914 {
              tunnel: [w1925 State_Type_Definitions."True Stop" ("Enum")] -> w1904
              tunnel: [w1923 w1941] -> w1903
              tunnel: w1907 -> [w1922 w1938]
              tunnel: w1909 -> [w1916 _]
              tunnel: [State_Type_Definitions."Idle" ("Enum") State_Type_Definitions."Shutdown" ("Enum")] -> w1905
              tunnel: w1912 -> [w1915 _]
              frame "None", Default {
                # ">> WIill proceed to part ii if not manual override >>"
                # ">>If ENABLE or Trigger is set to true>>"
                n634 = Or(x=w1915, y=w1916) -> (x .or. y?=w1917:bool)
                n635 = case shown="False" w1915 {
                  tunnel: [w1928 w1934] -> w1923
                  tunnel: w1922 -> [w1927 w1933]
                  frame False {
                    n636 = for {
                      shift-right: [w1930] -> w1928
                      shift-left: w1927 -> [w1931]
                      tunnel: string[] ["Z STEPPER BOX HEIGHT", "READ STEPPER VALUES"] ("element") -> [w1929] mode=indexing
                      n637 = Enqueue Element(queue=w1931, element=w1929) -> (queue out=w1930:refnum<queue>)  [unwired: 2 in, 2 out]
                    }
                  }
                  frame True {
                    n638 = for {
                      shift-right: [w1936] -> w1934
                      shift-left: w1933 -> [w1937]
                      tunnel: string[] ["READ IR", "", "", "", "", ""] -> [w1935] mode=indexing
                      n639 = Enqueue Element(queue=w1937, element=w1935) -> (queue out=w1936:refnum<queue>)  [unwired: 2 in, 2 out]
                    }
                  }
                }
                n640 = Select(t=State_Type_Definitions."True Stop" ("Enum"), s=w1916, f=State_Type_Definitions."Task A: MOVE FORWARD" ("Enum")) -> (s? t:f=w1919:u16)
                n641 = Select(t=w1919, s=w1917, f=State_Type_Definitions."Task A: RAISE ARM TO HEIGHT" ("Enum")) -> (s? t:f=w1925:u16)
              }
              frame "Exit" {
                n642 = for {
                  shift-right: [w1944] -> w1941
                  shift-left: w1938 -> [w1945]
                  tunnel: string[] ["STOP", "RESET ENCODERS", "RESET YAW", ""] -> [w1943] mode=indexing
                  n643 = Enqueue Element(queue=w1945, element=w1943) -> (queue out=w1944:refnum<queue>)  [unwired: 2 in, 2 out]
                }
              }
            }
          }
          frame 41 {
            # ">>> Motor control cluster >>>"
            # ">>> yStepper command>>>"
            # ">>Object detected>>"
            n644 = Dequeue Element(queue=w1954, timeout in ms (-1)=w1953, error in (no error)=w1952) -> (element=w1959:T7)  [unwired: 3 out]
            n645 = Less Or Equal?(x=w1948, y=30.0) -> (x <= y?=w1946:bool)
            "Table obstruct" <- w1946
            n646 = case shown="\"None\", Default" w1959 {
              tunnel: w1946 -> [w1962 _]
              tunnel: [w1969 State_Type_Definitions."True Stop" ("Enum")] -> w1958
              tunnel: w1951 -> [w1961 _]
              tunnel: w1955 -> [w1968 w1985]
              tunnel: [w1967 w1986] -> w1957
              tunnel: [State_Type_Definitions."Idle" ("Enum") State_Type_Definitions."Shutdown" ("Enum")] -> w1956
              frame "None", Default {
                n647 = case shown="False" w1962 {
                  tunnel: w1968 -> [w1972 w1979]
                  tunnel: [w1973 w1978] -> w1967
                  frame False {
                    n648 = for {
                      tunnel: string[] ["READ IR", "FORWARD", "READ NAVX"] ("element") -> [w1974] mode=indexing
                      shift-right: [w1976] -> w1973
                      shift-left: w1972 -> [w1975]
                      n649 = Enqueue Element(queue=w1975, element=w1974) -> (queue out=w1976:refnum<queue>)  [unwired: 2 in, 2 out]
                    }
                  }
                  frame True {
                    n650 = for {
                      shift-right: [w1981] -> w1978
                      shift-left: w1979 -> [w1982]
                      tunnel: string[] ["RESET ENCODERS", "READ NAVX", "READ ENCODERS"] -> [w1980] mode=indexing
                      n651 = Enqueue Element(queue=w1982, element=w1980) -> (queue out=w1981:refnum<queue>)  [unwired: 2 in, 2 out]
                    }
                  }
                }
                n652 = Or(x=w1962, y=w1961) -> (x .or. y?=w1960:bool)
                n653 = Select(t=State_Type_Definitions."True Stop" ("Enum"), s=w1961, f=State_Type_Definitions."True Stop" ("Enum")) -> (s? t:f=w1963:T6)
                n654 = Select(t=w1963, s=w1960, f=State_Type_Definitions."Task A: MOVE FORWARD" ("Enum")) -> (s? t:f=w1969:u16)
              }
              frame "Exit" {
                n655 = for {
                  shift-right: [w1989] -> w1986
                  shift-left: w1985 -> [w1990]
                  tunnel: string[] ["STOP", "RESET ENCODERS", "RESET YAW", "ARDUINO MODE 0"] -> [w1988] mode=indexing
                  n656 = Enqueue Element(queue=w1990, element=w1988) -> (queue out=w1989:refnum<queue>)  [unwired: 2 in, 2 out]
                }
              }
            }
          }
        }
      }
    }
    n657 = local write "Green LED"(w187) -> ()
  }
  n658 = while {
    tunnel: w45 -> [w2587]
    tunnel: w44 -> [w2584]
    stop <- w2581 stop-if-true
    # "Status Loop for Action Queues"
    n659 = Get Queue Status(queue=w2587, return elements? (F)=TRUE) -> (error out=w2583:errorcluster, # elements in queue=→"Action Queue Items":i32, elements=→"Action Queues items":string[])  [unwired: 1 in, 5 out]
    n660 = Get Queue Status(queue=w2584, return elements? (F)=TRUE) -> (# pending remove=→"State Logic Queue Items":i32, error out=w2582:errorcluster, elements=→"elements":T7[])  [unwired: 1 in, 5 out]
    n661 = Merge Errors(w2583, w2582) -> (w2581:errorcluster)
    n662 = Wait (ms)(milliseconds to wait=u32 500) -> ()  [unwired: 1 out]
  }
  n663 = call <vilib>:"DIO Close.vi"("error in (no error)"=w21, "DIO Info In"=w24) -> ()  [unwired: 9 in, 1 out]
  n664 = call <vilib>:"DIO Close.vi"("error in (no error)"=w31, "DIO Info In"=w33) -> ()  [unwired: 9 in, 1 out]
  n665 = call <vilib>:"NavX Close.vi"("error in (no error)"=w8, "NavX Info In"=w7) -> ()  [unwired: 9 in, 1 out]
  n666 = call <vilib>:"DIO Close.vi"("error in (no error)"=w26, "DIO Info In"=w28) -> ()  [unwired: 9 in, 1 out]
  n667 = call <vilib>:"DIO Close.vi"("error in (no error)"=w15, "DIO Info In"=w16) -> ()  [unwired: 9 in, 1 out]
  n668 = call <vilib>:"DIO Close.vi"("error in (no error)"=w10, "DIO Info In"=w11) -> ()  [unwired: 9 in, 1 out]
  n669 = while {
    stop <- w2591 stop-if-true
    n670 = call <vilib>:"RT Get CPU Loads.vi"() -> ("CPU loads"=→"CPU loads":T5[])  [unwired: 10 in, 1 out]
    n671 = Wait (ms)(milliseconds to wait=u32 100) -> ()  [unwired: 1 out]
    n672 = call "FGV Bool.vi"("Init/Read/Write State"=States_for_Action_Engine."Read") -> ("Output node"=w2591:bool)  [unwired: 2 in, 1 out]
  }
  n673 = while {
    stop <- w2595 stop-if-true
    n674 = call "MOTOR CONTROL WITH PID AE.vi"("AE Mode"=MOTOR_CONTROL_WITH_PID_AE_DATA_MODE_TYPE_DEF."Read from AE") -> ("Speed & distance"=→"Speed & distance":T1)  [unwired: 3 in]
    n675 = call "FGV Bool.vi"("Init/Read/Write State"=States_for_Action_Engine."Read") -> ("Output node"=w2595:bool)  [unwired: 2 in, 1 out]
    n676 = Wait (ms)(milliseconds to wait=u32 5) -> ()  [unwired: 1 out]
  }
  n677 = Merge Errors "Merge Errors"(w61, w60) -> (w43:errorcluster)
  n678 = Merge Errors(w47, w43) -> (w42:errorcluster)
  n679 = Destroy User Event(user event=w64, error in=w42) -> ()  [unwired: 1 out]
  n680 = Destroy User Event(user event=w65, error in=w42) -> ()  [unwired: 1 out]
  n681 = Unregister For Events(event registration refnum=w56, error in=w42) -> ()  [unwired: 1 out]
  n682 = Release Queue(queue=w38, error in (no error)=w42) -> (error out=→"error out":errorcluster)  [unwired: 1 in, 2 out]
  n683 = Release Queue(queue=w55, error in (no error)=w42) -> ()  [unwired: 1 in, 3 out]
